vi "LNK223-429BLF-No2.vi"() -> ()   [LabVIEW 2018]
uses:
  vi/DualHeadTestStage.ctl
  <vilib>/DAQmx/write.llb/DAQmx Write (Digital Bool 1Line 1Point).vi
  <vilib>/DAQmx/write.llb/DAQmx Write (Digital 1D Bool 1Chan 1Samp).vi
  <vilib>/DAQmx/read.llb/DAQmx Read (Digital 1D Bool 1Chan 1Samp).vi
  <vilib>/DAQmx/read.llb/DAQmx Read (Digital Bool 1Line 1Point).vi
  <vilib>/DAQmx/miscellaneous.llb/DAQmx Fill In Error Info.vi
panel:
  in  "Operator Mode:":enum32{"Admin", "Technician", "Operator"}(radio)=enum."Operator" caption="Radio Buttons"
  out "message":string
  out "AllowToTest":bool
  in  "DataIn":T1={"W0-SN"="2022-09", "W1-CUSTOMER"="LNK", "W2-TEST_DATE"="11/07/2019-14:51:57", "W3-TESTER"="LNK908-220309LF", "W4-RESULT"="P", "W5-TEXT1"="10CB6S194-C-2 10193406", "W6-TEXT2"="995982-3406", "W7-TEXT3"="", "W8-TEXT4"="", "W9-OPNAME"="FCT1", "W10-CDATE"="11/07/2019-14:51:57", "W11-CRITERIA"="", "W12-SYMPTOM"="", "W13-OPERATOR"="", "W14-WORKORDER"="", "W15-FIXTURE_ID"="", "W16-APIWO"="", "W17-TESTDURATION"=""}
  out "NOTE":string
  out "Check SUM HEX":string
  out "Serial number (Hex)":string
  out "TestTimeStr":string
  out "ProjectShort":string
  out "Project908":string
  out "number 2":i32
  out "length":i32
  out "TESTING HEAD#":string
  out "LowLimit 2":string
  out "standard error":string
  out "standard output":string
  out "Avg4V8":dbl
  out "Avg2V9":dbl
  out "Avg2V1":dbl
  out "Avg1V3":dbl
  out "text":string
  out "PWIDTH":dbl format="%#_6f"
  out "MAX AMP":dbl format="%#_6f"
  out "E3643A":refnum<visa-resource-name>="USB0::0x0957::0xB318::MY52420094::INSTR"
  out "DSO1052B":refnum<visa-resource-name>="USB0::0x0957::0x0588::CN55040431::INSTR"
  out "Result(Boolean)":bool
  out "TDS2002B":refnum<visa-resource-name>="GPIB0::7::INSTR"
  out "concatenated string":string
  out "LogfileHeaderXLS":string
  out "LowLimitForIntValue":string
  out "HighLimitForIntValue":string
  out "LowLimitForPulseCnt+400":string
  out "HighLimitForPulseCnt+400":string
  out "SSI_HighLimit":string
  out "SSI_LowLimit":string
  out "Position Get SSI-Pos":sgl format="%.2f"
  out "Position Get SSI-Neg*-1":sgl format="%.2f"
  out "ADC val":sgl format="%.2f"
  out "DriveEnable":bool
  out "Result(Boolean) 4":bool
  out "Result(Boolean) 3":bool
  out "Result(Boolean) 2":bool
  out "Result(DecimalPoint)2":dbl
  out "MicroFlexRS232":refnum<visa-resource-name>="COM5"
  out "33210A":refnum<visa-resource-name>="USB0::0x0957::0xB318::MY52420094::INSTR"
  out "34461A":refnum<visa-resource-name>="USB0::0x0957::0xB318::MY52420094::INSTR"
  out "E3643A#3":refnum<visa-resource-name>="USB0::0x0957::0xB318::MY52420094::INSTR"
  out "E3643A#2":refnum<visa-resource-name>="USB0::0x0957::0xB318::MY52420094::INSTR"
  out "E3643A#1":refnum<visa-resource-name>="USB0::0x0957::0xB318::MY52420094::INSTR"
  out "KA3003P":refnum<visa-resource-name>
  out "Project index":i32
  out "KA6003P":refnum<visa-resource-name>
  out "A5114-12":refnum<visa-resource-name>
  out "A5116-02":refnum<visa-resource-name>
  out "SN-STS":i16
  out "TDS3012C":refnum<visa-resource-name>
  out "Result":string
  out "E3631A":refnum<visa-resource-name>="USB0::0x0957::0xB318::MY52420094::INSTR"
  out "Index TestTime":i16
  out "Break Step#":string
  in  "Clear list of break step":string[](array[string])
  out "RowSize":i32
  out "TestPlanDimensions":i32[](array[numeric])
  out "BreakStep#":string[](array[string])
  out "CMD":string
  out "Remark":string
  out "Equipment":string
  out "SetDelayResChk":i8
  out "Step#":string
  out "FailedFlag":i8
  out "TestLoop":string
  out "Return CMD":string
  out "Status of Set CMD":bool
  out "COMPST":string
  out "Reading":string
  out "UPL":string
  out "LWL":string
  out "Step&Description":string
  out "SeqFileSts":bool
  out "Start Time":dbl
  out "Comment":string
  out "StartTime":string
  out "Project":string
  out "CUSTOMER":string
  out "FIRMWARE REV":string
  out "SOFTWARE REV":string
  out "UNIT  PASS/FAIL STATUS":string
  out "TESTER ID":string
  out "LineLogFile":string
  out "SumDisp_Low_Inc":i32
  out "All Test Status in Sum Disp":string
  out "Test Step# >> Sum Disp":string
  out "Action":string
  out "Unit":string
  out "HighLimit":string
  out "LowLimit":string
  out "FailedCode":string
  out "Status >> Sum Disp":string
  out "Reading >> Sum Disp":string
  out "TESTPLAN ARRAY":string[][](array[string])
  out "BarCode Exit":bool
  out "TestPlan_Row_Inc":i32
  out "Ok STS":bool
  out "Project Model":string
  in  "Tab Control":T2(tab)
  out "TESTPLAN ARRAY Display":string[][](table) caption="Table Control"
  in  "Test Modes":enum32{"Auto", "Step"}(radio) caption="Test Mode:"
  out "ID STS":bool
  in  "ID OK":bool
  in  "Operator ID":string
  in  "stop":bool
  out "PASS/FAIL STATUS":bool caption="PASSED"
  out "Test Time (Sec)":dbl
  out "Serial Number":string
  in  "RunAllSeq?":bool
  in  "Break step#":string(combo)="Index"
  out "Index":string
  out "InitialValueAfter":i32
  out "FailedCdDisp":string
  out "ProjectFull":string
  out "Result(Boolean) 1":bool
  in  "RS485 RECEIVER":refnum<visa-resource-name>="COM7"
  out "Numeric":i32
  out "trimmed string":string
  out "number":dbl
  out "Username":string
  in  "Tab Control 2":enum32{"Test result", "Waveform"}(tab)
  out "Summary Display":string[][](table) caption="Table Control"
  out "WF_CCW":cluster{"Numeric":dbl, "Numeric":dbl}[](graph)
  out "WF_CW":cluster{"Numeric":dbl, "Numeric":dbl}[](graph)
  in  "SERIAL NUMBER HEAD 1":string
  in  "SERIAL NUMBER HEAD 2":string
  out "Test Time HEAD 1":dbl
  out "Test Time HEAD 2":dbl
  out "HEAD 1":u8(slide) scale=0.0..71.0
  out "HEAD 2":u8(slide) scale=0.0..71.0
  out "PASS/FAIL STATUS  HEAD 1":bool caption="PASSED"
  out "PASS/FAIL STATUS  HEAD 2":bool
  out "FailedCdDisp H1":string
  out "FailedCdDisp H2":string
  out "Result(DecimalPoint)":sgl format="%#_10g"
  out "Description":string
  out "App Firmware":string=" -openD:\\20161122\\LNK01E-213300ALF\\LNK213-300ALF\\SW0077076V1-04.hex"
  out "MUX RELAY":refnum<visa-resource-name>
  out "34450A":refnum<visa-resource-name>="USB0::0x0957::0xB318::MY52420094::INSTR"
  in  "34410A":refnum<visa-resource-name>="USB0::0x0957::0x0607::MY53018867::INSTR"
  out "Test time report":string[][](array[string])
  out "TestDesc+TestTime":string
  out "GeneralHeader":string
  out "TestDataHeader":string
  out "LogfileHeaderCSV":string
  out "FailedStep":string
  out "InitialValue":i32
  in  "Station":string="FCT1"
  in  "Fixture/PalletteID":string="1"
  in  "Note":string
  in  "Reserve#1":string
  in  "Reserve#2":string
  in  "TestSoftwareVersion":string="V1.0"
  out "Result(Number)":i32
  out "Result(string)":string
  out "VAR_TYPE":string
  out "Result(Number)2":i32
  in  "RUNTEST":bool
  in  "RESET_ICT100":bool
  in  "OK Button 2":bool
  in  "OK Button":bool
  out "Fail Test Param":string
  out "Stop_Buffer":bool
  # "1"
  # "0"
  # "USB0::0x0957::0x0607::MY53018867::INSTR"
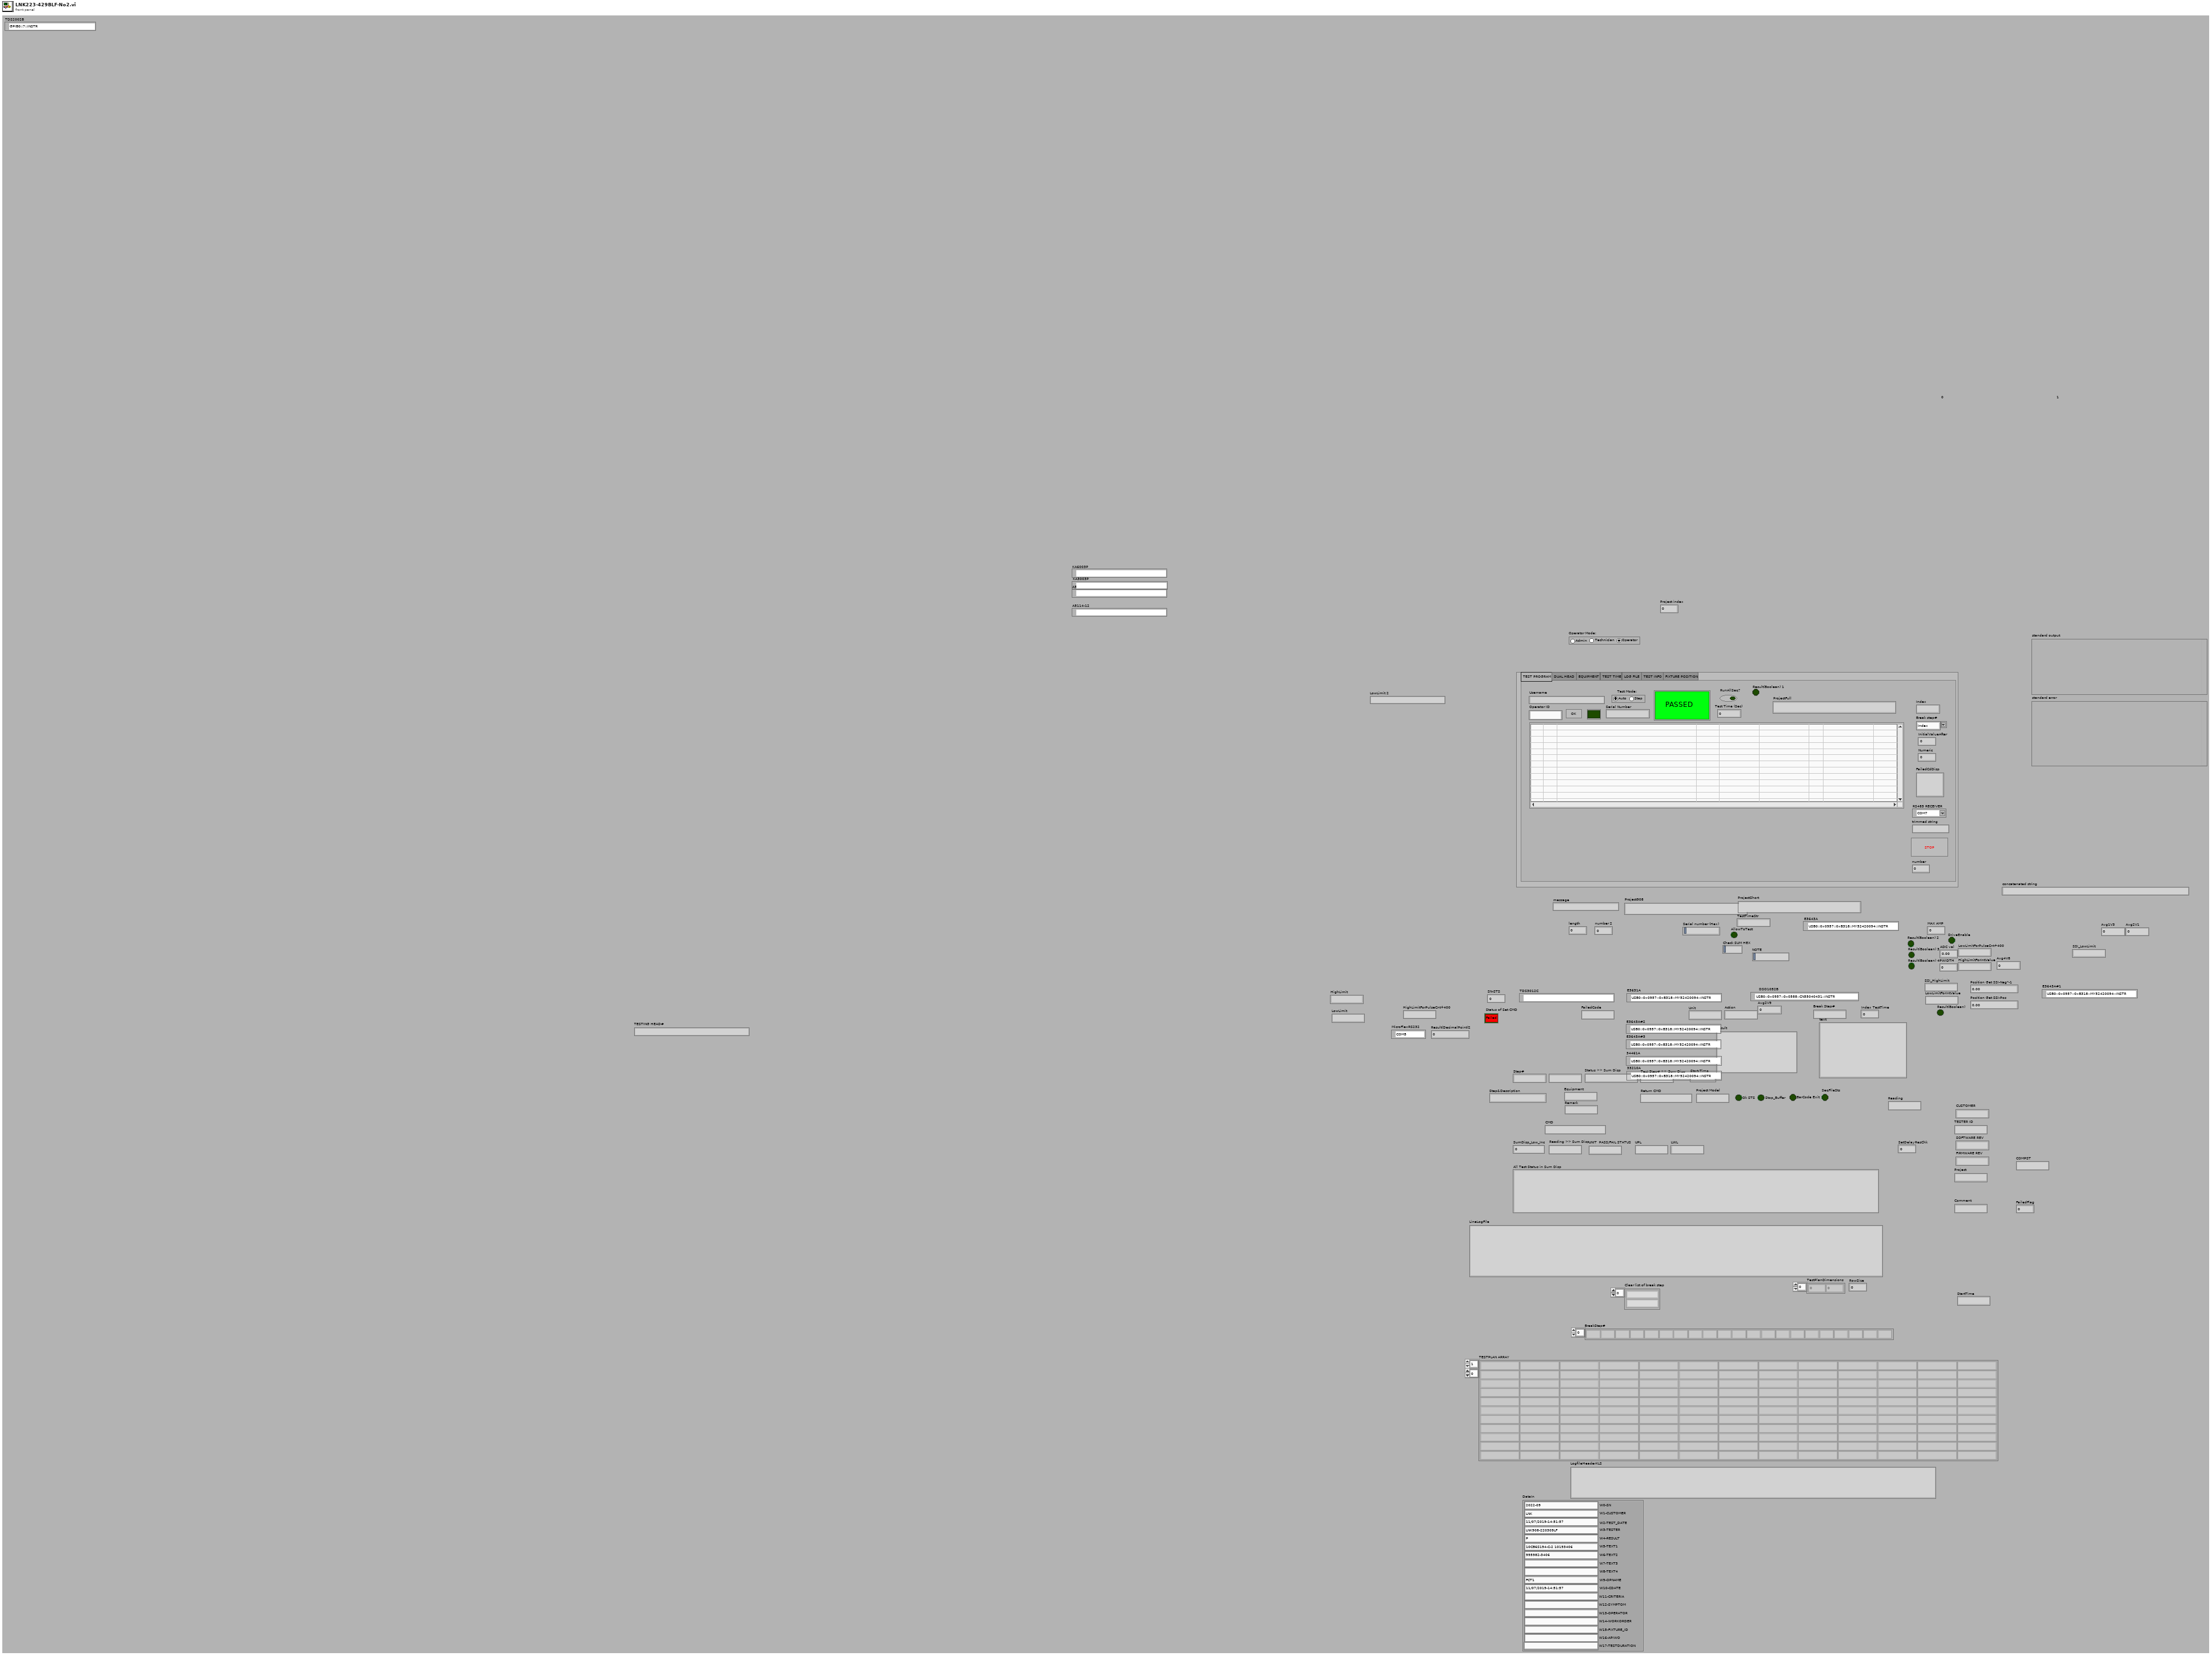
[diagram p1: front panel]
types:
  T1 = cluster{"W0-SN":string, "W1-CUSTOMER":string, "W2-TEST_DATE":string, "W3-TESTER":string, "W4-RESULT":string, "W5-TEXT1":string, "W6-TEXT2":string, "W7-TEXT3":string, "W8-TEXT4":string, "W9-OPNAME":string, "W10-CDATE":string, "W11-CRITERIA":string, "W12-SYMPTOM":string, "W13-OPERATOR":string, "W14-WORKORDER":string, "W15-FIXTURE_ID":string, "W16-APIWO":string, "W17-TESTDURATION":string}
  T2 = enum32{"TEST PROGRAM", "DUAL HEAD", "EQUIPMENT", "TEST TIME", "LOG FILE", "TEST INFO", "FIXTURE POSITION"}
  T3 = enum32{"1", "10", "20", "50", "100", "500", "1000"}
  T4 = enum32{"Set Relay", "Append Relay", "Clear Relay", "Manual Cmd"}
  T5 = typedef "DualHeadTestStage.ctl" = enum16{"Initial", "CheckHead1", "CheckHead2", "LoadTestPlanHead1", "LoadTestPlanHead2", "StartTest"}
  T6 = enum16{"FREQUENCY", "MEAN", "PERIOD", "PK2PK", "MIN", "MAX", "RISE", "FALL", "CRMS", "PWIDTH", "NWIDTH", "NONE"}
  T7 = enum16{"MEAS1", "MEAS2", "MEAS3", "MEAS4", "MEAS5"}
  T8 = cluster{"disabled index (col)":i32, "disabled index (col)":i32}
  T9 = cluster{"TestPlan_Row_Inc":i32, "disabled index (col)":i32}
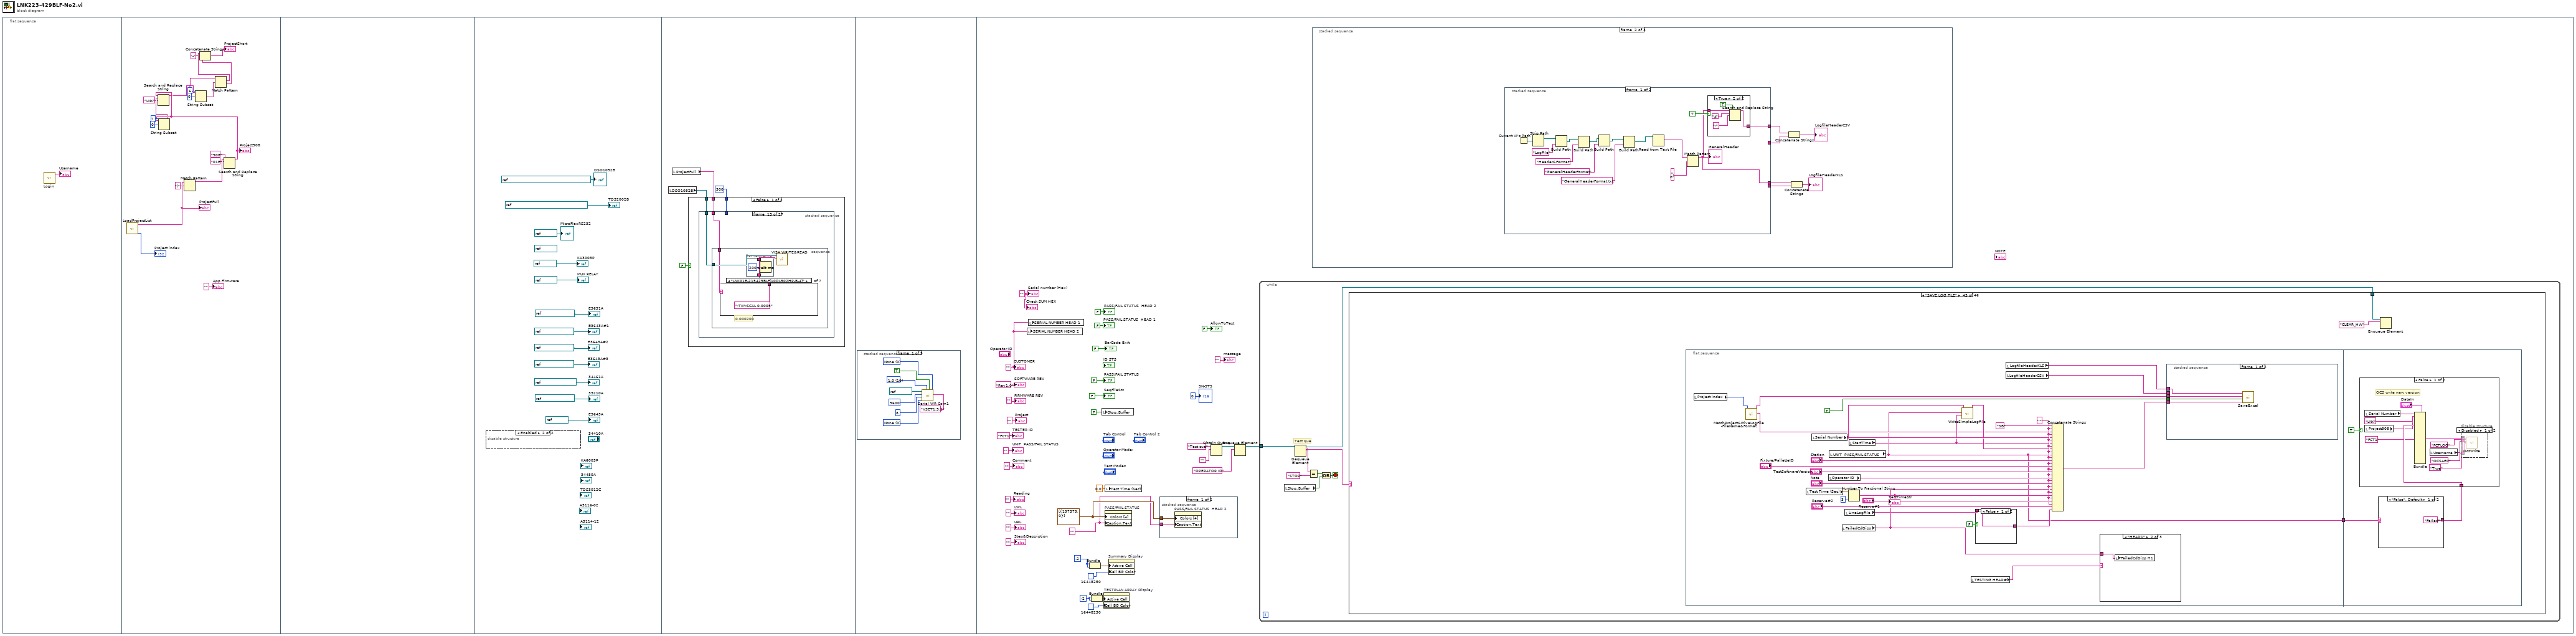
[diagram p0: block diagram]
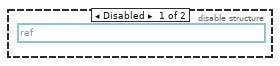
[diagram p2: hidden frame]
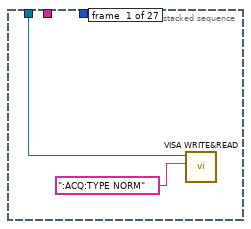
[diagram p3: hidden frame]
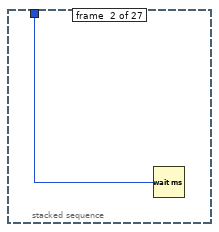
[diagram p4: hidden frame]
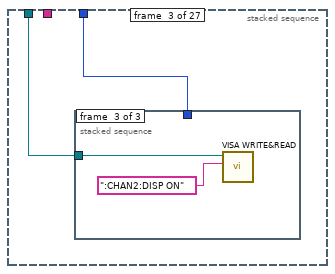
[diagram p5: hidden frame]
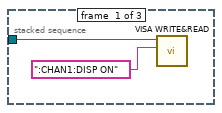
[diagram p6: hidden frame]
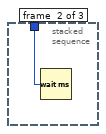
[diagram p7: hidden frame]
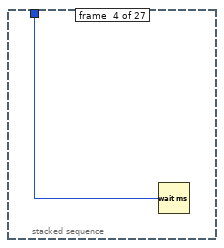
[diagram p8: hidden frame]
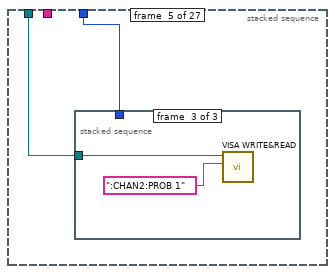
[diagram p9: hidden frame]
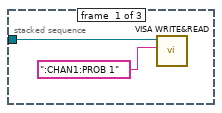
[diagram p10: hidden frame]
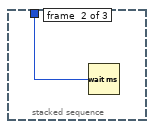
[diagram p11: hidden frame]
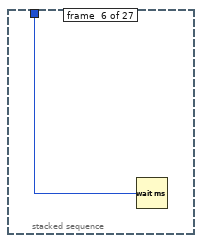
[diagram p12: hidden frame]
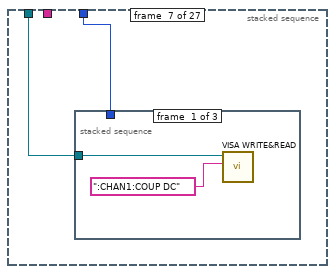
[diagram p13: hidden frame]
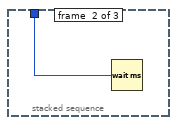
[diagram p14: hidden frame]
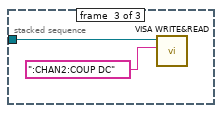
[diagram p15: hidden frame]
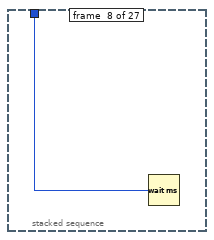
[diagram p16: hidden frame]
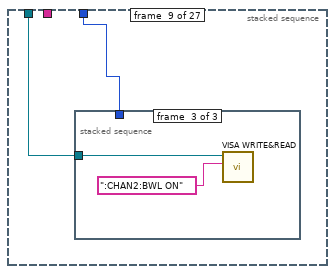
[diagram p17: hidden frame]
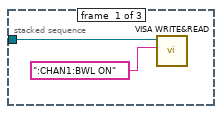
[diagram p18: hidden frame]
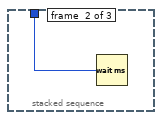
[diagram p19: hidden frame]
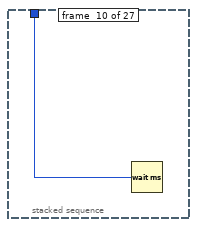
[diagram p20: hidden frame]
diagram:
  n1 = flat-sequence {
    frame #0 {
      n2 = call "Login.vi"() -> ("Username"=→"Username":string)  [unwired: 11 in]
    }
    frame #1 {
      n3 = call "LoadProjectList.vi"() -> ("Index"=→"Project index":i32, "SelectedProject"=w20:string)  [unwired: 10 out]
      "ProjectFull" <- w20
      n4 = Match Pattern(string=w20, regular expression="(") -> (before substring=w18:string)  [unwired: 1 in, 3 out]
      n5 = Search and Replace String(input string=w18, search string="01E", replace string="908" ("replace string (\"\")")) -> (result string=w12:string)  [unwired: 5 in, 3 out]
      "Project908" <- w12
      n6 = String Subset(string=w12, offset (0)=0, length (rest)=7 ("length (rest)")) -> (substring=w13:string)
      n7 = Search and Replace String(input string=w12, search string=w13, replace string="LNK" ("replace string (\"\")")) -> (result string=w8:string)  [unwired: 5 in, 3 out]
      n8 = String Subset(string=w8, offset (0)=0, length (rest)=6 ("length (rest)")) -> (substring=w7:string)
      n9 = Match Pattern(string=w8, regular expression=w7) -> (match substring=w6:string, after substring=w5:string)  [unwired: 1 in, 2 out]
      n10 = Concatenate Strings(w6, "-" ("string"), w5) -> (→"ProjectShort":string)
      "App Firmware" <- "" ("App Firmware")
    }
    frame #2 {
    }
    frame #3 {
      (unwired) refnum<visa-resource-name> "COM1" ("SPK RELAY")
      n11 = disable-structure shown="Enabled" {
        frame Disabled {
          (unwired) refnum<visa-resource-name> "USB0::0x0957::0x0607::MY53018867::INSTR" ("E3631A")
        }
        frame Enabled {
        }
      }
      "MUX RELAY" <- refnum<visa-resource-name> "COM1" ("SPK RELAY")
      "E3631A" <- refnum<visa-resource-name> "GPIB0::1::INSTR" ("E3631A")
      "KA3003P" <- refnum<visa-resource-name> "COM2" ("SPK RELAY")
      "E3643A#1" <- refnum<visa-resource-name> "GPIB0::2::INSTR" ("E3631A")
      "E3643A#2" <- refnum<visa-resource-name> "GPIB0::3::INSTR" ("E3631A")
      "E3643A#3" <- refnum<visa-resource-name> "GPIB0::4::INSTR" ("E3631A")
      "34461A" <- refnum<visa-resource-name> "GPIB0::22::INSTR" ("E3631A")
      "33210A" <- refnum<visa-resource-name> "GPIB0::6::INSTR" ("E3631A")
      "MicroFlexRS232" <- refnum<visa-resource-name> "COM5" ("SPK RELAY")
      "TDS2002B" <- refnum<visa-resource-name> "USB0::0x0699::0x03A1::C041443::INSTR" ("TDS1001B")
      "DSO1052B" <- refnum<visa-resource-name> "USB0::0x0957::0x0588::CN56489397::INSTR" ("VISA resource name In")
      "E3643A" <- refnum<visa-resource-name> "COM3" ("E3643A#1 2")
    }
    frame #4 {
      n12 = local read "DSO1052B"() -> (w36:refnum<visa-resource-name>)
      n13 = local read "ProjectFull"() -> (w34:string)
      n14 = case shown="False" FALSE {
        tunnel: w36 -> [w40 _]
        tunnel: u32 300 ("milliseconds to wait") -> [w39 _]
        tunnel: w34 -> [w38 _]
        frame False {
          n15 = stacked-sequence {
            tunnel: w40 -> [w42 _ w45 _ w53 _ w61 _ w69 _ w77 _ w85 _ w100 _ w104 _ w108 _ w113 _ w123 _ w132 w148 w154]
            tunnel: w39 -> [_ w43 w44 w51 w52 w59 w60 w67 w68 w75 w76 w83 _ w99 _ w103 _ w107 _ w111 _ w121 w122 w129 w131 w149 w153]
            tunnel: w38 -> [_ _ _ _ _ _ _ _ _ _ _ _ w84 _ _ _ _ _ _ _ w112 _ _ _ w130 _ _]
            frame #0 {
              n16 = call "VISA WRITE&READ.vi"("write buffer"=":ACQ:TYPE NORM", "VISA resource name In"=w42) -> ()  [unwired: 7 in, 3 out]
            }
            frame #1 {
              n17 = Wait (ms)(milliseconds to wait=w43) -> ()  [unwired: 1 out]
            }
            frame #2 {
              n18 = stacked-sequence {
                tunnel: w45 -> [w47 _ w50]
                tunnel: w44 -> [_ w48 _]
                frame #0 {
                  n19 = call "VISA WRITE&READ.vi"("write buffer"=":CHAN1:DISP ON", "VISA resource name In"=w47) -> ()  [unwired: 7 in, 3 out]
                }
                frame #1 {
                  n20 = Wait (ms)(milliseconds to wait=w48) -> ()  [unwired: 1 out]
                }
                frame #2 {
                  n21 = call "VISA WRITE&READ.vi"("write buffer"=":CHAN2:DISP ON", "VISA resource name In"=w50) -> ()  [unwired: 7 in, 3 out]
                }
              }
            }
            frame #3 {
              n22 = Wait (ms)(milliseconds to wait=w51) -> ()  [unwired: 1 out]
            }
            frame #4 {
              n23 = stacked-sequence {
                tunnel: w53 -> [w55 _ w58]
                tunnel: w52 -> [_ w56 _]
                frame #0 {
                  n24 = call "VISA WRITE&READ.vi"("write buffer"=":CHAN1:PROB 1", "VISA resource name In"=w55) -> ()  [unwired: 7 in, 3 out]
                }
                frame #1 {
                  n25 = Wait (ms)(milliseconds to wait=w56) -> ()  [unwired: 1 out]
                }
                frame #2 {
                  n26 = call "VISA WRITE&READ.vi"("write buffer"=":CHAN2:PROB 1", "VISA resource name In"=w58) -> ()  [unwired: 7 in, 3 out]
                }
              }
            }
            frame #5 {
              n27 = Wait (ms)(milliseconds to wait=w59) -> ()  [unwired: 1 out]
            }
            frame #6 {
              n28 = stacked-sequence {
                tunnel: w61 -> [w63 _ w66]
                tunnel: w60 -> [_ w64 _]
                frame #0 {
                  n29 = call "VISA WRITE&READ.vi"("write buffer"=":CHAN1:COUP DC", "VISA resource name In"=w63) -> ()  [unwired: 7 in, 3 out]
                }
                frame #1 {
                  n30 = Wait (ms)(milliseconds to wait=w64) -> ()  [unwired: 1 out]
                }
                frame #2 {
                  n31 = call "VISA WRITE&READ.vi"("write buffer"=":CHAN2:COUP DC", "VISA resource name In"=w66) -> ()  [unwired: 7 in, 3 out]
                }
              }
            }
            frame #7 {
              n32 = Wait (ms)(milliseconds to wait=w67) -> ()  [unwired: 1 out]
            }
            frame #8 {
              n33 = stacked-sequence {
                tunnel: w69 -> [w71 _ w74]
                tunnel: w68 -> [_ w72 _]
                frame #0 {
                  n34 = call "VISA WRITE&READ.vi"("write buffer"=":CHAN1:BWL ON", "VISA resource name In"=w71) -> ()  [unwired: 7 in, 3 out]
                }
                frame #1 {
                  n35 = Wait (ms)(milliseconds to wait=w72) -> ()  [unwired: 1 out]
                }
                frame #2 {
                  n36 = call "VISA WRITE&READ.vi"("write buffer"=":CHAN2:BWL ON", "VISA resource name In"=w74) -> ()  [unwired: 7 in, 3 out]
                }
              }
            }
            frame #9 {
              n37 = Wait (ms)(milliseconds to wait=w75) -> ()  [unwired: 1 out]
            }
            frame #10 {
              n38 = stacked-sequence {
                tunnel: w77 -> [w79 _ w82]
                tunnel: w76 -> [_ w80 _]
                frame #0 {
                  n39 = call "VISA WRITE&READ.vi"("write buffer"=":CHAN1:INV OFF", "VISA resource name In"=w79) -> ()  [unwired: 7 in, 3 out]
                }
                frame #1 {
                  n40 = Wait (ms)(milliseconds to wait=w80) -> ()  [unwired: 1 out]
                }
                frame #2 {
                  n41 = call "VISA WRITE&READ.vi"("write buffer"=":CHAN2:INV OFF", "VISA resource name In"=w82) -> ()  [unwired: 7 in, 3 out]
                }
              }
            }
            frame #11 {
              n42 = Wait (ms)(milliseconds to wait=w83) -> ()  [unwired: 1 out]
            }
            frame #12 {
              n43 = stacked-sequence {
                tunnel: w85 -> [w89]
                tunnel: w84 -> [w88]
                frame #0 {
                  # "0.000200"
                  n44 = case shown="\"LNK01E-215429BLF(10DL502HP-B-4)\"" w88 {
                    tunnel: [":TIM:SCAL 0.01" ("write buffer") ":TIM:SCAL 0.005" ("write buffer") ":TIM:SCAL 0.01" ("write buffer") ":TIM:SCAL 0.0005" ("write buffer") ":TIM:SCAL 0.0005" ("write buffer") ":TIM:SCAL 0.0005" ("write buffer") ":TIM:SCAL 0.0005" ("write buffer")] -> w86
                    frame "False", Default {
                    }
                    frame "LNK01E-213299LF(10DL5H)" {
                    }
                    frame "LNK01E-213301LF(10DL4H)" {
                    }
                    frame "LNK01E-213300ALF(10DL12H)" {
                    }
                    frame "LNK01E-215429ALF(10DL502HP)" {
                    }
                    frame "LNK01E-223429BLF(10DL502HP-D-0)" {
                    }
                    frame "LNK01E-215429BLF(10DL502HP-B-4)" {
                    }
                  }
                  n45 = flat-sequence {
                    tunnel: [w91] -> w87
                    tunnel: w86 -> [w91]
                    frame #0 {
                      n46 = Wait (ms)(milliseconds to wait=u32 200) -> ()  [unwired: 1 out]
                    }
                  }
                  n47 = call "VISA WRITE&READ.vi"("write buffer"=w87, "VISA resource name In"=w89) -> ()  [unwired: 7 in, 3 out]
                }
              }
            }
            frame #13 {
              n48 = Wait (ms)(milliseconds to wait=w99) -> ()  [unwired: 1 out]
            }
            frame #14 {
              n49 = stacked-sequence {
                tunnel: w100 -> [w102]
                frame #0 {
                  n50 = call "VISA WRITE&READ.vi"("write buffer"=":TRIG:MODE EDGE", "VISA resource name In"=w102) -> ()  [unwired: 7 in, 3 out]
                }
              }
            }
            frame #15 {
              n51 = Wait (ms)(milliseconds to wait=w103) -> ()  [unwired: 1 out]
            }
            frame #16 {
              n52 = stacked-sequence {
                tunnel: w104 -> [w106]
                frame #0 {
                  n53 = call "VISA WRITE&READ.vi"("write buffer"=":TRIG:EDGE:SLOP POS", "VISA resource name In"=w106) -> ()  [unwired: 7 in, 3 out]
                }
              }
            }
            frame #17 {
              n54 = Wait (ms)(milliseconds to wait=w107) -> ()  [unwired: 1 out]
            }
            frame #18 {
              n55 = stacked-sequence {
                tunnel: w108 -> [w110]
                frame #0 {
                  n56 = call "VISA WRITE&READ.vi"("write buffer"=":TRIG:EDGE:SOUR CHAN2", "VISA resource name In"=w110) -> ()  [unwired: 7 in, 3 out]
                }
              }
            }
            frame #19 {
              n57 = Wait (ms)(milliseconds to wait=w111) -> ()  [unwired: 1 out]
            }
            frame #20 {
              n58 = stacked-sequence {
                tunnel: w113 -> [w116]
                tunnel: w112 -> [w114]
                frame #0 {
                  n59 = case shown="\"LNK01E-213300LF(10DL12H)\"" w114 {
                    tunnel: [":TRIG:EDGE:LEV 2.5" ("write buffer") ":TRIG:EDGE:LEV 8" ("write buffer") ":TRIG:EDGE:LEV 2.5" ("write buffer") ":TRIG:EDGE:LEV 4" ("write buffer")] -> w115
                    frame "False", Default {
                    }
                    frame "LNK01E-213299LF(10DL5H)" {
                    }
                    frame "LNK01E-213301LF(10DL4H)" {
                    }
                    frame "LNK01E-213300LF(10DL12H)" {
                    }
                  }
                  n60 = call "VISA WRITE&READ.vi"("write buffer"=w115, "VISA resource name In"=w116) -> ()  [unwired: 7 in, 3 out]
                }
              }
            }
            frame #21 {
              n61 = Wait (ms)(milliseconds to wait=w121) -> ()  [unwired: 1 out]
            }
            frame #22 {
              n62 = stacked-sequence {
                tunnel: w123 -> [w125 _ w128]
                tunnel: w122 -> [_ w126 _]
                frame #0 {
                  n63 = call "VISA WRITE&READ.vi"("write buffer"=":CHAN1:SCAL 2", "VISA resource name In"=w125) -> ()  [unwired: 7 in, 3 out]
                }
                frame #1 {
                  n64 = Wait (ms)(milliseconds to wait=w126) -> ()  [unwired: 1 out]
                }
                frame #2 {
                  n65 = call "VISA WRITE&READ.vi"("write buffer"=":CHAN2:SCAL 2", "VISA resource name In"=w128) -> ()  [unwired: 7 in, 3 out]
                }
              }
            }
            frame #23 {
              n66 = Wait (ms)(milliseconds to wait=w129) -> ()  [unwired: 1 out]
            }
            frame #24 {
              n67 = stacked-sequence {
                tunnel: w132 -> [w135 _ w143]
                tunnel: w131 -> [_ w140 _]
                tunnel: w130 -> [w134 _ w141]
                frame #0 {
                  n68 = case shown="\"LNK01E-213300LF(10DL12H)\"" w134 {
                    tunnel: [":CHAN1:OFFS -6" ("write buffer") ":CHAN1:OFFS -6" ("write buffer") ":CHAN1:OFFS -6" ("write buffer") ":CHAN1:OFFS 0" ("write buffer")] -> w133
                    frame "False", Default {
                    }
                    frame "LNK01E-213299LF(10DL5H)" {
                    }
                    frame "LNK01E-213301LF(10DL4H)" {
                    }
                    frame "LNK01E-213300LF(10DL12H)" {
                    }
                  }
                  n69 = call "VISA WRITE&READ.vi"("write buffer"=w133, "VISA resource name In"=w135) -> ()  [unwired: 7 in, 3 out]
                }
                frame #1 {
                  n70 = Wait (ms)(milliseconds to wait=w140) -> ()  [unwired: 1 out]
                }
                frame #2 {
                  n71 = case shown="\"LNK01E-213300LF(10DL12H)\"" w141 {
                    tunnel: [":CHAN2:OFFS -6" ("write buffer") ":CHAN2:OFFS -6" ("write buffer") ":CHAN2:OFFS -6" ("write buffer") ":CHAN2:OFFS 0" ("write buffer")] -> w142
                    frame "False", Default {
                    }
                    frame "LNK01E-213299LF(10DL5H)" {
                    }
                    frame "LNK01E-213301LF(10DL4H)" {
                    }
                    frame "LNK01E-213300LF(10DL12H)" {
                    }
                  }
                  n72 = call "VISA WRITE&READ.vi"("write buffer"=w142, "VISA resource name In"=w143) -> ()  [unwired: 7 in, 3 out]
                }
              }
            }
            frame #25 {
              n73 = stacked-sequence {
                tunnel: w149 -> [w150 _]
                tunnel: w148 -> [_ w152]
                frame #0 {
                  n74 = Wait (ms)(milliseconds to wait=w150) -> ()  [unwired: 1 out]
                }
                frame #1 {
                  n75 = call "VISA WRITE&READ.vi"("write buffer"=":TIM:MAIN:OFFS  0", "VISA resource name In"=w152) -> ()  [unwired: 7 in, 3 out]
                }
              }
            }
            frame #26 {
              n76 = stacked-sequence {
                tunnel: w154 -> [w156 _ w159]
                tunnel: w153 -> [_ w157 _]
                frame #0 {
                  n77 = call "DSO1072B_WaveformCMD1.vi"("DSO1072B CMD"=":WAV:POIN:MODE MAX", "VISA resource name In"=w156) -> ()  [unwired: 7 in, 3 out]
                }
                frame #1 {
                  n78 = Wait (ms)(milliseconds to wait=w157) -> ()  [unwired: 1 out]
                }
                frame #2 {
                  n79 = call "DSO1072B_WaveformCMD1.vi"("DSO1072B CMD"=":WAV:FORM BYTE", "VISA resource name In"=w159) -> ()  [unwired: 7 in, 3 out]
                }
              }
            }
          }
        }
        frame True {
          n80 = stacked-sequence {
            frame #0 {
              n81 = local read "TDS2002B"() -> (w160:refnum<visa-resource-name>)
              n82 = call "RUN-STOP-SING SEQ.vi"("VISA"=w160, "ACQUIRE"=enum32{"RUN", "SINGLE SEQ"}."RUN") -> ()
            }
            frame #1 {
              n83 = local read "TDS2002B"() -> (w163:refnum<visa-resource-name>)
              n84 = call "ACQMODE.vi"("ACQ MODE"=enum16{"SAMPLE", "PEAK DETECT", "AVERAGE"}."PEAK DETECT", "VISA resource name"=w163) -> ()  [unwired: 1 in]
            }
            frame #2 {
              n85 = local read "TDS2002B"() -> (w164:refnum<visa-resource-name>)
              n86 = call "SELECT_CHANEL.vi"("VISA resource name"=w164, "CH4"=FALSE, "CH3"=FALSE, "CH2"=TRUE, "CH1"=TRUE) -> ()
            }
            frame #3 {
              n87 = stacked-sequence {
                frame #0 {
                  n88 = local read "TDS2002B"() -> (w171:refnum<visa-resource-name>)
                  n89 = call "PROB ATTEN SETTING.vi"("ATTENUATIONs:"=T3."1", "CHANNEL"=enum32{"CH 1", "CH 2", "CH 3", "CH 4"}."CH 1", "VISA resource name 2"=w171) -> ()  [unwired: 9 in]
                }
                frame #1 {
                  n90 = local read "TDS2002B"() -> (w174:refnum<visa-resource-name>)
                  n91 = call "PROB ATTEN SETTING.vi"("ATTENUATIONs:"=T3."1", "CHANNEL"=enum32{"CH 1", "CH 2", "CH 3", "CH 4"}."CH 2", "VISA resource name 2"=w174) -> ()  [unwired: 9 in]
                }
              }
            }
            frame #4 {
              n92 = stacked-sequence {
                frame #0 {
                  n93 = local read "TDS2002B"() -> (w177:refnum<visa-resource-name>)
                  n94 = call "CH COUPLING SETTING.vi"("COUPLING:"=enum32{"AC", "DC", "GND"}."DC", "CHANNEL"=enum32{"CH 1", "CH 2", "CH 3", "CH 4"}."CH 1", "VISA resource name 2"=w177) -> ()  [unwired: 9 out]
                }
                frame #1 {
                  n95 = local read "TDS2002B"() -> (w180:refnum<visa-resource-name>)
                  n96 = call "CH COUPLING SETTING.vi"("COUPLING:"=enum32{"AC", "DC", "GND"}."DC", "CHANNEL"=enum32{"CH 1", "CH 2", "CH 3", "CH 4"}."CH 2", "VISA resource name 2"=w180) -> ()  [unwired: 9 out]
                }
              }
            }
            frame #5 {
              n97 = stacked-sequence {
                frame #0 {
                  n98 = local read "TDS2002B"() -> (w181:refnum<visa-resource-name>)
                  n99 = call "PROBE INV SETTING.vi"("INV / NON INV"=enum16{"NON INV", "INV"}."NON INV", "CH"=enum16{"CH 1", "CH 2", "CH 3", "CH 4"}."CH 1", "VISA TSD2014B"=w181) -> ()  [unwired: 9 in]
                }
                frame #1 {
                  n100 = local read "TDS2002B"() -> (w184:refnum<visa-resource-name>)
                  n101 = call "PROBE INV SETTING.vi"("INV / NON INV"=enum16{"NON INV", "INV"}."NON INV", "CH"=enum16{"CH 1", "CH 2", "CH 3", "CH 4"}."CH 2", "VISA TSD2014B"=w184) -> ()  [unwired: 9 out]
                }
              }
            }
            frame #6 {
              n102 = local read "TDS2002B"() -> (w187:refnum<visa-resource-name>)
              n103 = call "HOR_POS_SETTING.vi"("VISA TDS1012"=w187, "HOR_POS (SEC)   LEFT=+  RIGHT=-"="0") -> ()
            }
            frame #7 {
              n104 = local read "TDS2002B"() -> (w190:refnum<visa-resource-name>)
              n105 = call "HOR_SCALE_SETTING.vi"("VISA TDS1012"=w190, "HOR_SCAIL"="5E-3") -> ()
            }
            frame #8 {
              n106 = local read "TDS2002B"() -> (w193:refnum<visa-resource-name>)
              n107 = call "TRIGER_EDGE.vi"("TRIGGER EDGE"=enum32{"SLOPE RISE", "SLOPE FALL"}."SLOPE RISE", "SOURCE"=enum32{"CH 1", "CH 2", "CH 3", "CH 4"}."CH 1", "VISA TDS1012"=w193) -> ()
            }
            frame #9 {
              n108 = local read "TDS2002B"() -> (w196:refnum<visa-resource-name>)
              n109 = call "TRIGER_LEVEL.vi"("VISA resource name"=w196, "V Unit"=enum32{"mVOLT", "VOLT"}."VOLT", "TRIGER MAIN LEVEL"="2.5") -> ()
            }
            frame #10 {
              n110 = stacked-sequence {
                frame #0 {
                  n111 = local read "TDS2002B"() -> (w199:refnum<visa-resource-name>)
                  n112 = call "VER_POS_SETTING.vi"("VER POS"="1", "VOLTS/DIV"=enum32{"CH1", "CH2", "CH3", "CH4"}."CH1", "VISA resource name"=w199) -> ()
                }
                frame #1 {
                  n113 = local read "TDS2002B"() -> (w202:refnum<visa-resource-name>)
                  n114 = call "VER_SCALE_SETTING.vi"("VER RANGE"="2", "VOLTS/DIV"=enum32{"CH 1", "CH 2", "CH 3", "CH 4"}."CH 1", "VISA resource name"=w202) -> ()
                }
              }
            }
            frame #11 {
              n115 = stacked-sequence {
                frame #0 {
                  n116 = local read "TDS2002B"() -> (w205:refnum<visa-resource-name>)
                  n117 = call "VER_POS_SETTING.vi"("VER POS"="-3", "VOLTS/DIV"=enum32{"CH1", "CH2", "CH3", "CH4"}."CH2", "VISA resource name"=w205) -> ()
                }
                frame #1 {
                  n118 = local read "TDS2002B"() -> (w208:refnum<visa-resource-name>)
                  n119 = call "VER_SCALE_SETTING.vi"("VER RANGE"="2", "VOLTS/DIV"=enum32{"CH 1", "CH 2", "CH 3", "CH 4"}."CH 2", "VISA resource name"=w208) -> ()
                }
              }
            }
          }
        }
      }
    }
    frame #5 {
      n120 = stacked-sequence {
        frame #0 {
          w211 = u16 0 items=["None"=0, "XON/XOFF"=1, "RTS/CTS"=2, "DTR/DSR"=4] ("flow control")
          w213 = u16 10 items=["1.0"=10, "1.5"=15, "2.0"=20] ("stop bits")
          w214 = u16 0 items=["None", "Odd", "Even", "Mark", "Space"] ("parity")
          n121 = call "Serial WR Com1.vi"("string to write"="VSET1:5.1", "flow control"=w211, "write"=TRUE, "stop bits"=w213, "parity"=w214, "data bits"=u16 8, "baud rate"=u32 9600, "VISA resource name"=refnum<visa-resource-name> "COM2") -> ()  [unwired: 2 in, 2 out]
        }
        frame #1 {
          w222 = u16 0 items=["None"=0, "XON/XOFF"=1, "RTS/CTS"=2, "DTR/DSR"=4] ("flow control")
          w220 = u16 10 items=["1.0"=10, "1.5"=15, "2.0"=20] ("stop bits")
          w219 = u16 0 items=["None", "Odd", "Even", "Mark", "Space"] ("parity")
          n122 = call "Serial WR Com1.vi"("string to write"="ISET1:0.05", "flow control"=w222, "write"=TRUE, "stop bits"=w220, "parity"=w219, "data bits"=u16 8, "baud rate"=u32 9600, "VISA resource name"=refnum<visa-resource-name> "COM2") -> ()  [unwired: 2 in, 2 out]
        }
        frame #2 {
          w227 = u16 0 items=["None"=0, "XON/XOFF"=1, "RTS/CTS"=2, "DTR/DSR"=4] ("flow control")
          w229 = u16 10 items=["1.0"=10, "1.5"=15, "2.0"=20] ("stop bits")
          w230 = u16 0 items=["None", "Odd", "Even", "Mark", "Space"] ("parity")
          n123 = call "Serial WR Com1.vi"("string to write"="OUT1", "flow control"=w227, "write"=TRUE, "stop bits"=w229, "parity"=w230, "data bits"=u16 8, "baud rate"=u32 9600, "VISA resource name"=refnum<visa-resource-name> "COM2") -> ()  [unwired: 2 in, 2 out]
        }
        frame #3 {
          w241 = u16 0 items=["None"=0, "XON/XOFF"=1, "RTS/CTS"=2, "DTR/DSR"=4] ("flow control")
          w239 = u16 10 items=["1.0"=10, "1.5"=15, "2.0"=20] ("stop bits")
          w238 = u16 0 items=["None", "Odd", "Even", "Mark", "Space"] ("parity")
          n124 = Concatenate Strings("APPL 13.2,0.1" ("string to write"), "\r\n") -> (w234:string)
          n125 = call "Serial WR Com1.vi"("string to write"=w234, "flow control"=w241, "write"=TRUE, "stop bits"=w239, "parity"=w238, "data bits"=u16 8, "baud rate"=u32 9600, "VISA resource name"=refnum<visa-resource-name> "COM3") -> ()  [unwired: 2 in, 2 out]
        }
        frame #4 {
          w251 = u16 0 items=["None"=0, "XON/XOFF"=1, "RTS/CTS"=2, "DTR/DSR"=4] ("flow control")
          w249 = u16 10 items=["1.0"=10, "1.5"=15, "2.0"=20] ("stop bits")
          w248 = u16 0 items=["None", "Odd", "Even", "Mark", "Space"] ("parity")
          n126 = Concatenate Strings("OUTP ON" ("string to write"), "\r\n") -> (w244:string)
          n127 = call "Serial WR Com1.vi"("string to write"=w244, "flow control"=w251, "write"=TRUE, "stop bits"=w249, "parity"=w248, "data bits"=u16 8, "baud rate"=u32 9600, "VISA resource name"=refnum<visa-resource-name> "COM3") -> ()  [unwired: 2 in, 2 out]
        }
      }
    }
    frame #6 {
      w255 = "" ("Serial number (Hex)")
      w262 = -2 ("disabled index (col)")
      w266 = -2
      w257 = "" ("Caption.Text")
      w258 = cluster{u32, u32}[] [{197379, 0}] ("Colors [4]")
      w256 = "" ("SOFTWARE REV")
      n128 = local write "SERIAL NUMBER HEAD 2"(w256) -> ()
      n129 = local write "SERIAL NUMBER HEAD 1"(w256) -> ()
      n130 = Bundle(w266, w266) -> (w267:cluster{i32, i32})  [unwired: 1 out]
      n131 = Bundle("disabled index (col)"=w262, "disabled index (col)"=w262) -> (w263:T8)  [unwired: 1 out]
      n132 = local write "Stop_Buffer"(FALSE ("Stop_Buffer")) -> ()
      n133 = property on="TESTPLAN ARRAY Display" class="Tbl (strict)"("Active Cell"=w263, "Cell BG Color"=u32 16448250) -> ()  [unwired: 2 in, 2 out]
      n134 = property on="PASS/FAIL STATUS" class="Bool (strict)"("Colors [4]"=w258, "Caption.Text"=w257) -> ()  [unwired: 2 in, 2 out]
      n135 = local write "Test Time (Sec)"(0.0 ("Cycle Time (Sec)")) -> ()
      n136 = property on="Summary Display" class="Tbl (strict)"("Active Cell"=w267, "Cell BG Color"=u32 16448250) -> ()  [unwired: 2 in, 2 out]
      n137 = stacked-sequence {
        tunnel: w258 -> [w289 w291]
        tunnel: w257 -> [w288 w290]
        frame #0 {
          n138 = property on="PASS/FAIL STATUS  HEAD 2" class="Bool (strict)"("Colors [4]"=w289, "Caption.Text"=w288) -> ()  [unwired: 2 in, 2 out]
        }
        frame #1 {
          n139 = property on="PASS/FAIL STATUS  HEAD 1" class="Bool (strict)"("Colors [4]"=w291, "Caption.Text"=w290) -> ()  [unwired: 2 in, 2 out]
        }
      }
      n140 = Obtain Queue(name (unnamed)="Test cue", element data type="") -> (queue out=w286:refnum<queue>)  [unwired: 3 in, 2 out]
      n141 = Enqueue Element(queue=w286, element="OPERATOR ID") -> (queue out=w283:refnum<queue>)  [unwired: 1 in, 3 out]
      n142 = while {
        tunnel: w283 -> [w416]
        stop <- w412 stop-if-true
        # "Test que"
        n143 = local read "Stop_Buffer"() -> (w411:bool)
        n144 = Dequeue Element(queue=w416) -> (queue out=w413:refnum<queue>, element=w414:string)  [unwired: 1 in, 3 out]
        n145 = Equal?(x=w414, y="STOP") -> (x = y?=w410:bool)
        n146 = Or(x=w410, y=w411) -> (x .or. y?=w412:bool)
        n147 = case shown="\"SAVE LOG FILE\"" w414 {
          tunnel: w413 -> [_ w418 w572 w639 w806 w930 w947 w959 w990 w1018 w1034 w1046 w1152 w1377 w1430 w1449 w1563 w1571 w1583 w1586 w1588 w1596 w1610 w1613 w1636 w1671 w1706 w1741 w1776 w1807 w1832 w1843 w1858 w1903 w2036 w2051 w2087 w2173 w2184 w2186 w2319 w2473 w2509 _ w2595 w2606]
          frame "False", Default {
            n148 = One Button Dialog(message="There is a wrong command or text error in test sequence file, Please check! ") -> ()  [unwired: 2 out]
          }
          frame "DUAL-HEAD-TESTING" {
            n149 = while {
              shift-right: [w422] -> _
              shift-left: DualHeadTestStage."Initial" ("DualHeadTestStage") -> [w423]
              tunnel: w418 -> [w421]
              stop <- w420 stop-if-true
              n150 = case shown="\"CheckHead2\"" w423 {
                tunnel: [DualHeadTestStage."CheckHead1" ("DualHeadTestStage") w434 w451 w463 w478 DualHeadTestStage."Initial" ("DualHeadTestStage")] -> w422
                tunnel: w421 -> [_ _ _ _ _ w570]
                tunnel: [FALSE FALSE FALSE FALSE FALSE TRUE] -> w420
                frame "Initial", Default {
                  w424 = u8 0 ("HEAD 2")
                  n151 = local write "HEAD 1"(w424) -> ()
                  n152 = local write "HEAD 2"(w424) -> ()
                  "TESTING HEAD#" <- "" ("TESTING HEAD#")
                }
                frame "CheckHead1" {
                  n153 = local read "ProjectFull"() -> (w439:string)
                  n154 = case shown="\"False\", Default" w439 {
                    tunnel: [0 ("y") 37 ("y") 17 ("y")] -> w428
                    frame "False", Default {
                    }
                    frame "LNK01E-223429BLF(10DL502HP-D-0)" {
                    }
                    frame "LNK01E-215429BLF(10DL502HP-B-4)" {
                    }
                  }
                  "number 2" <- w428
                  n155 = String Length(string="SERIAL NUMBER HEAD 1") -> (length=w432:i32)
                  "length" <- w432
                  n156 = call "DAQ Assistant"() -> ("data"=w437:bool[])  [unwired: 17 in, 2 out]
                  n157 = Equal?(x=w432, y=w428) -> (x = y?=w431:bool)
                  n158 = Index Array(array=w437, index=0) -> (element=w429:bool)
                  n159 = Not(x=w429) -> (.not. x?=w430:bool)
                  n160 = And(x=w431, y=w430) -> (x .and. y?=w435:bool)
                  n161 = case shown="True" w435 {
                    tunnel: [DualHeadTestStage."CheckHead2" ("DualHeadTestStage") DualHeadTestStage."LoadTestPlanHead1" ("DualHeadTestStage")] -> w434
                    frame False {
                    }
                    frame True {
                    }
                  }
                }
                frame "CheckHead2" {
                  n162 = local read "ProjectFull"() -> (w455:string)
                  n163 = case shown="\"LNK01E-223429BLF(10DL502HP-D-0)\"" w455 {
                    tunnel: [0 ("y") 17 ("y") 37 ("y")] -> w445
                    frame "False", Default {
                    }
                    frame "LNK01E-215429BLF(10DL502HP-B-4)" {
                    }
                    frame "LNK01E-223429BLF(10DL502HP-D-0)" {
                    }
                  }
                  n164 = String Length(string="SERIAL NUMBER HEAD 2") -> (length=w449:i32)
                  n165 = call "DAQ Assistant2"() -> ("data"=w454:bool[])  [unwired: 17 in, 2 out]
                  n166 = Equal?(x=w449, y=w445) -> (x = y?=w448:bool)
                  n167 = Index Array(array=w454, index=0) -> (element=w446:bool)
                  n168 = Not(x=w446) -> (.not. x?=w447:bool)
                  n169 = And(x=w448, y=w447) -> (x .and. y?=w452:bool)
                  n170 = case shown="False" w452 {
                    tunnel: [DualHeadTestStage."CheckHead1" ("DualHeadTestStage") DualHeadTestStage."LoadTestPlanHead2" ("DualHeadTestStage")] -> w451
                    frame False {
                    }
                    frame True {
                    }
                  }
                }
                frame "LoadTestPlanHead1" {
                  n171 = stacked-sequence {
                    tunnel: [_ _ DualHeadTestStage."StartTest" ("DualHeadTestStage")] -> w463
                    frame #0 {
                    }
                    frame #1 {
                    }
                    frame #2 {
                      n172 = flat-sequence {
                        frame #0 {
                          w466 = "" ("Caption.Text")
                          w465 = cluster{u32, u32}[] [{197379, 197379}] ("Colors [4]")
                          n173 = property on="PASS/FAIL STATUS" class="Bool (strict)"("Colors [4]"=w465, "Caption.Text"=w466) -> ()  [unwired: 2 in, 2 out]
                          n174 = property on="PASS/FAIL STATUS  HEAD 1" class="Bool (strict)"("Colors [4]"=w465, "Caption.Text"=w466) -> ()  [unwired: 2 in, 2 out]
                        }
                        frame #1 {
                          n175 = local read "MUX RELAY"() -> (w468:refnum<visa-resource-name>)
                          n176 = call "ControlRelay_ver10.vi"("VISA session"=w468, "write buffer"="Bb000", "Relay Setting"=T4."Manual Cmd") -> ()  [unwired: 10 in, 7 out]
                        }
                        frame #2 {
                          n177 = local write "TESTING HEAD#"("HEAD1" ("TESTING HEAD#")) -> ()
                          "FailedCdDisp H1" <- "" ("FailedCdDisp H1")
                        }
                        frame #3 {
                          n178 = while {
                            i -> [w476]
                            stop <- w473 stop-if-true
                            n179 = Wait (ms)(milliseconds to wait=u32 1) -> ()  [unwired: 1 out]
                            n180 = property on="SERIAL NUMBER HEAD 2" class="Str"("Key Focus"=TRUE) -> ()  [unwired: 2 in, 2 out]
                            n181 = Equal?(x=w476, y=5) -> (x = y?=w473:bool)
                          }
                        }
                      }
                    }
                  }
                }
                frame "LoadTestPlanHead2" {
                  n182 = stacked-sequence {
                    tunnel: [_ _ DualHeadTestStage."StartTest" ("DualHeadTestStage")] -> w478
                    frame #0 {
                    }
                    frame #1 {
                    }
                    frame #2 {
                      n183 = flat-sequence {
                        frame #0 {
                          w481 = "" ("Caption.Text")
                          w480 = cluster{u32, u32}[] [{197379, 197379}] ("Colors [4]")
                          n184 = property on="PASS/FAIL STATUS" class="Bool (strict)"("Colors [4]"=w480, "Caption.Text"=w481) -> ()  [unwired: 2 in, 2 out]
                          n185 = property on="PASS/FAIL STATUS  HEAD 2" class="Bool (strict)"("Colors [4]"=w480, "Caption.Text"=w481) -> ()  [unwired: 2 in, 2 out]
                        }
                        frame #1 {
                          n186 = local read "MUX RELAY"() -> (w483:refnum<visa-resource-name>)
                          n187 = call "ControlRelay_ver10.vi"("VISA session"=w483, "write buffer"="Bb000", "Relay Setting"=T4."Manual Cmd") -> ()  [unwired: 10 in, 7 out]
                        }
                        frame #2 {
                          n188 = local write "TESTING HEAD#"("HEAD2" ("TESTING HEAD#")) -> ()
                          n189 = Wait (ms)(milliseconds to wait=u32 50) -> ()  [unwired: 1 out]
                          "FailedCdDisp H2" <- "" ("FailedCdDisp H2")
                        }
                        frame #3 {
                          n190 = local read "ProjectFull"() -> (w488:string)
                          n191 = case shown="\"LNK01E-223429BLF(10DL502HP-D-0)\"" w488 {
                            frame "False", Default {
                            }
                            frame "LNK01E-213299LF(10DL5H)" {
                              # "SWAP TO TEST HEAD 2"
                              n192 = local read "MUX RELAY"() -> (w490:refnum<visa-resource-name>)
                              n193 = call "ControlRelay_ver10.vi"("VISA session"=w490, "write buffer"="@b041t", "Relay Setting"=T4."Manual Cmd") -> ()  [unwired: 10 in, 7 out]
                            }
                            frame "LNK01E-213300LF(10DL12H)" {
                              # "SWAP TO TEST HEAD 2"
                              n194 = flat-sequence {
                                tunnel: [w494] -> w493
                                tunnel: w493 -> [w498]
                                tunnel: [w498] -> w492
                                tunnel: w492 -> [w499]
                                frame #0 {
                                n195 = local read "MUX RELAY"() -> (w494:refnum<visa-resource-name>)
                                n196 = call "ControlRelay_ver10.vi"("VISA session"=w494, "write buffer"="@b013t", "Relay Setting"=T4."Manual Cmd") -> ()  [unwired: 10 in, 7 out]
                                }
                                frame #1 {
                                n197 = Wait (ms)(milliseconds to wait=u32 1000) -> ()  [unwired: 1 out]
                                }
                                frame #2 {
                                n198 = call "ControlRelay_ver10.vi"("VISA session"=w499, "write buffer"="@b020t", "Relay Setting"=T4."Manual Cmd") -> ()  [unwired: 10 in, 7 out]
                                }
                              }
                            }
                            frame "LNK01E-213300ALF(10DL12H)" {
                              # "SWAP TO TEST HEAD 2"
                              n199 = flat-sequence {
                                tunnel: [w504] -> w503
                                tunnel: w503 -> [w508]
                                tunnel: [w508] -> w502
                                tunnel: w502 -> [w509]
                                frame #0 {
                                n200 = local read "MUX RELAY"() -> (w504:refnum<visa-resource-name>)
                                n201 = call "ControlRelay_ver10.vi"("VISA session"=w504, "write buffer"="@b013t", "Relay Setting"=T4."Manual Cmd") -> ()  [unwired: 10 in, 7 out]
                                }
                                frame #1 {
                                n202 = Wait (ms)(milliseconds to wait=u32 1000) -> ()  [unwired: 1 out]
                                }
                                frame #2 {
                                n203 = call "ControlRelay_ver10.vi"("VISA session"=w509, "write buffer"="@b020t", "Relay Setting"=T4."Manual Cmd") -> ()  [unwired: 10 in, 7 out]
                                }
                              }
                            }
                            frame "LNK01E-215429ALF(10DL502HP)" {
                              # "SWAP TO TEST HEAD 2"
                              n204 = flat-sequence {
                                tunnel: [w515] -> w513
                                tunnel: w513 -> [w519]
                                tunnel: [w519] -> w512
                                tunnel: w512 -> [w521]
                                frame #0 {
                                n205 = local read "MUX RELAY"() -> (w515:refnum<visa-resource-name>)
                                n206 = call "ControlRelay_ver10.vi"("VISA session"=w515, "baud rate (9600)"=u32 19200, "write buffer"="Bb013t", "Relay Setting"=T4."Manual Cmd") -> ()  [unwired: 9 in, 7 out]
                                }
                                frame #1 {
                                n207 = Wait (ms)(milliseconds to wait=u32 1000) -> ()  [unwired: 1 out]
                                }
                                frame #2 {
                                n208 = call "ControlRelay_ver10.vi"("VISA session"=w521, "baud rate (9600)"=u32 19200, "write buffer"="Bb020t", "Relay Setting"=T4."Manual Cmd") -> ()  [unwired: 9 in, 7 out]
                                }
                              }
                            }
                            frame "LNK01E-223429BLF(10DL502HP-D-0)" {
                              # "SWAP TO TEST HEAD 2"
                              n209 = flat-sequence {
                                tunnel: [w527] -> w525
                                tunnel: w525 -> [w531]
                                tunnel: [w531] -> w524
                                tunnel: w524 -> [w533]
                                frame #0 {
                                n210 = local read "MUX RELAY"() -> (w527:refnum<visa-resource-name>)
                                n211 = call "ControlRelay_ver10.vi"("VISA session"=w527, "baud rate (9600)"=u32 19200, "write buffer"="Bb013t", "Relay Setting"=T4."Manual Cmd") -> ()  [unwired: 9 in, 7 out]
                                }
                                frame #1 {
                                n212 = Wait (ms)(milliseconds to wait=u32 1000) -> ()  [unwired: 1 out]
                                }
                                frame #2 {
                                n213 = call "ControlRelay_ver10.vi"("VISA session"=w533, "baud rate (9600)"=u32 19200, "write buffer"="Bb020t", "Relay Setting"=T4."Manual Cmd") -> ()  [unwired: 9 in, 7 out]
                                }
                              }
                            }
                            frame "LNK01E-215429BLF(10DL502HP-B-4)" {
                              # "SWAP TO TEST HEAD 2"
                              n214 = flat-sequence {
                                tunnel: [w539] -> w537
                                tunnel: w537 -> [w543]
                                tunnel: [w543] -> w536
                                tunnel: w536 -> [w545]
                                frame #0 {
                                n215 = local read "MUX RELAY"() -> (w539:refnum<visa-resource-name>)
                                n216 = call "ControlRelay_ver10.vi"("VISA session"=w539, "baud rate (9600)"=u32 19200, "write buffer"="Bb013t", "Relay Setting"=T4."Manual Cmd") -> ()  [unwired: 9 in, 7 out]
                                }
                                frame #1 {
                                n217 = Wait (ms)(milliseconds to wait=u32 1000) -> ()  [unwired: 1 out]
                                }
                                frame #2 {
                                n218 = call "ControlRelay_ver10.vi"("VISA session"=w545, "baud rate (9600)"=u32 19200, "write buffer"="Bb020t", "Relay Setting"=T4."Manual Cmd") -> ()  [unwired: 9 in, 7 out]
                                }
                              }
                            }
                            frame "LNK908-215429LF(10DL501HP)" {
                              # "SWAP TO TEST HEAD 2"
                              n219 = flat-sequence {
                                frame #0 {
                                n220 = local read "MUX RELAY"() -> (w548:refnum<visa-resource-name>)
                                n221 = call "ControlRelay_ver10.vi"("VISA session"=w548, "write buffer"="@b007t", "Relay Setting"=T4."Manual Cmd") -> ()  [unwired: 10 in, 7 out]
                                }
                                frame #1 {
                                n222 = Wait (ms)(milliseconds to wait=u32 1000) -> ()  [unwired: 1 out]
                                }
                                frame #2 {
                                n223 = local read "MUX RELAY"() -> (w554:refnum<visa-resource-name>)
                                n224 = call "ControlRelay_ver10.vi"("VISA session"=w554, "write buffer"="@b013t", "Relay Setting"=T4."Manual Cmd") -> ()  [unwired: 10 in, 7 out]
                                }
                                frame #3 {
                                n225 = Wait (ms)(milliseconds to wait=u32 1000) -> ()  [unwired: 1 out]
                                }
                                frame #4 {
                                n226 = local read "MUX RELAY"() -> (w556:refnum<visa-resource-name>)
                                n227 = call "ControlRelay_ver10.vi"("VISA session"=w556, "write buffer"="@b043t", "Relay Setting"=T4."Manual Cmd") -> ()  [unwired: 10 in, 7 out]
                                }
                              }
                            }
                            frame "LNK01E-213301LF(10DL4H)" {
                              # "SWAP TO TEST HEAD 2"
                              n228 = local read "MUX RELAY"() -> (w560:refnum<visa-resource-name>)
                              n229 = call "ControlRelay_ver10.vi"("VISA session"=w560, "write buffer"="@b042t", "Relay Setting"=T4."Manual Cmd") -> ()  [unwired: 10 in, 7 out]
                            }
                          }
                        }
                        frame #4 {
                          n230 = while {
                            i -> [w565]
                            stop <- w562 stop-if-true
                            n231 = Wait (ms)(milliseconds to wait=u32 1) -> ()  [unwired: 1 out]
                            n232 = property on="SERIAL NUMBER HEAD 1" class="Str"("Key Focus"=TRUE) -> ()  [unwired: 2 in, 2 out]
                            n233 = Equal?(x=w565, y=5) -> (x = y?=w562:bool)
                          }
                        }
                      }
                    }
                  }
                }
                frame "StartTest" {
                  w567 = 0.0
                  n234 = local write "Test Time HEAD 2"(w567) -> ()
                  n235 = local write "Test Time HEAD 1"(w567) -> ()
                  n236 = Enqueue Element(queue=w570, element="BARCODE SCANER") -> ()  [unwired: 1 in, 4 out]
                }
              }
            }
          }
          frame "OPERATOR ID" {
            n237 = flat-sequence {
              tunnel: w572 -> [w626]
              frame #0 {
                n238 = while {
                  stop <- w575 stop-if-true
                  n239 = flat-sequence {
                    tunnel: [w584] -> w576
                    tunnel: w576 -> [w606]
                    tunnel: [w605] -> w574
                    frame #0 {
                      n240 = while {
                        i -> [w582]
                        stop <- w580 stop-if-true
                        n241 = Equal?(x=3, y=w582) -> (x = y?=w580:bool)
                        n242 = property on="Operator ID" class="Str"("Key Focus"=TRUE) -> ()  [unwired: 2 in, 2 out]
                        n243 = Wait (ms)(milliseconds to wait=u32 250) -> ()  [unwired: 1 out]
                      }
                      n244 = local write "Operator ID"("" ("Operator ID")) -> ()
                      n245 = local write "ID STS"(FALSE ("Boolean")) -> ()
                    }
                    frame #1 {
                      n246 = while {
                        tunnel: [w586] -> w584
                        stop <- w587 stop-if-true
                        n247 = local read "SeqFileSts"() -> (w585:bool)
                        n248 = case shown="False" w585 {
                          tunnel: ["ID OK" w590] -> w586
                          frame False {
                          }
                          frame True {
                            n249 = flat-sequence {
                              tunnel: [FALSE ("ID OK")] -> w590
                              frame #0 {
                                n250 = Stop(stop? (T)=TRUE) -> ()
                              }
                              frame #1 {
                              }
                            }
                          }
                        }
                        n251 = local read "Stop_Buffer"() -> (w588:bool)
                        n252 = Or(x=w586, y=w588) -> (x .or. y?=w587:bool)
                      }
                    }
                    frame #2 {
                      n253 = Current VI's Path() -> (path=w594:path)
                      n254 = local read "Operator Mode:"() -> (w607:enum32{"Admin", "Technician", "Operator"})
                      n255 = Strip Path(path=w594) -> (stripped path=w595:path)  [unwired: 1 out]
                      n256 = Build Path(base path=w595, name or relative path="SwConfig") -> (appended path=w598:path)
                      n257 = Build Path(base path=w598, name or relative path="SoftwareConfigulation.txt") -> (appended path=w599:path)
                      n258 = Read from Text File(file (use dialog)=w599) -> (text=w600:string)  [unwired: 1 in, 5 out]
                      n259 = Match Pattern(string=w600, regular expression="OperatorId=" ("name or relative path")) -> (after substring=w602:string)  [unwired: 4 out]
                      n260 = Match Pattern(string=w602, regular expression="\n" ("name or relative path")) -> (before substring=w604:string)  [unwired: 4 out]
                      n261 = Decimal String To Number(string=w604) -> (number=w593:i32)  [unwired: 3 out]
                      n262 = case shown="\"Operator\"" w607 {
                        tunnel: w606 -> [w608 w609 w612]
                        tunnel: [w608 w609 w611] -> w605
                        tunnel: w593 -> [_ _ w610]
                        frame "Admin", Default {
                        }
                        frame "Technician" {
                        }
                        frame "Operator" {
                          n263 = case shown="True" w612 {
                            tunnel: [FALSE w615] -> w611
                            tunnel: w610 -> [_ w614]
                            frame False {
                            }
                            frame True {
                              n264 = local read "Operator ID"() -> (w618:string)
                              n265 = String Length(string=w618) -> (length=w617:i32)
                              n266 = Equal?(x=w617, y=w614) -> (x = y?=w616:bool)
                              n267 = case shown="False" w616 {
                                tunnel: [w619 w623] -> w615
                                frame False {
                                n268 = stacked-sequence {
                                tunnel: [_ _ FALSE] -> w619
                                frame #0 {
                                n269 = One Button Dialog(message="Please enter 5 digits of operator ID!\nFor example : 12345      ") -> ()  [unwired: 2 out]
                                }
                                frame #1 {
                                n270 = local write "ID STS"(FALSE ("Boolean")) -> ()
                                }
                                frame #2 {
                                }
                                }
                                }
                                frame True {
                                n271 = stacked-sequence {
                                tunnel: [_ TRUE] -> w623
                                frame #0 {
                                n272 = local write "ID STS"(TRUE ("Boolean")) -> ()
                                }
                                frame #1 {
                                }
                                }
                                }
                              }
                            }
                          }
                        }
                      }
                    }
                  }
                  n273 = local read "Stop_Buffer"() -> (w573:bool)
                  n274 = Or(x=w574, y=w573) -> (x .or. y?=w575:bool)
                }
              }
              frame #1 {
                n275 = flat-sequence {
                  tunnel: w626 -> [w634]
                  frame #0 {
                    n276 = Wait (ms)(milliseconds to wait=u32 500) -> ()  [unwired: 1 out]
                  }
                  frame #1 {
                    n277 = while {
                      i -> [w632]
                      stop <- w629 stop-if-true
                      n278 = Wait (ms)(milliseconds to wait=u32 1) -> ()  [unwired: 1 out]
                      n279 = property on="SERIAL NUMBER HEAD 1" class="Str"("Key Focus"=TRUE) -> ()  [unwired: 2 in, 2 out]
                      n280 = Equal?(x=w632, y=15) -> (x = y?=w629:bool)
                    }
                  }
                  frame #2 {
                    n281 = local read "Stop_Buffer"() -> (w633:bool)
                    n282 = case shown="False" w633 {
                      tunnel: w634 -> [w636 w637]
                      frame False {
                        (unwired) "BARCODE SCANER" ("element")
                        n283 = Enqueue Element(queue=w636, element="DUAL-HEAD-TESTING") -> ()  [unwired: 1 in, 4 out]
                      }
                      frame True {
                        n284 = Enqueue Element(queue=w637, element="STOP") -> ()  [unwired: 1 in, 4 out]
                      }
                    }
                  }
                }
              }
            }
          }
          frame "BARCODE SCANER" {
            n285 = flat-sequence {
              tunnel: w639 -> [w729]
              frame #0 {
                n286 = case shown="True" FALSE {
                  frame False {
                    n287 = disable-structure shown="Enabled" {
                      frame Disabled {
                        n288 = local read "SERIAL NUMBER HEAD 1"() -> (w649:string)
                        n289 = Empty String/Path?(string/path=w649) -> (empty?=w644:bool)
                        n290 = case shown="True" w644 {
                          tunnel: w649 -> [w654 _]
                          tunnel: [w654 w655] -> w648
                          frame False {
                          }
                          frame True {
                            n291 = local read "SERIAL NUMBER HEAD 2"() -> (w655:string)
                          }
                        }
                        n292 = local read "Username"() -> (w642:string)
                        n293 = call "APIGet-Mis.vi"("SerialNumber"=w648, "OpName"="FCT1", "Operator"=w642, "PopUp"="False", "OcsSever"="OCSAEC") -> ("AllowToTest"=w645:bool, "Message"=w643:string)  [unwired: 9 in, 4 out]
                        n294 = case shown="False" w645 {
                          tunnel: w644 -> [w651 _]
                          tunnel: w643 -> [w650 _]
                          frame False {
                            n295 = case shown="True" w651 {
                              frame False {
                                n296 = local write "SERIAL NUMBER HEAD 1"("" ("SERIAL NUMBER HEAD 1")) -> ()
                              }
                              frame True {
                                n297 = local write "SERIAL NUMBER HEAD 2"("" ("SERIAL NUMBER HEAD 2")) -> ()
                              }
                            }
                            n298 = One Button Dialog(message=w650) -> ()  [unwired: 1 in, 1 out]
                          }
                          frame True {
                          }
                        }
                        n299 = local write "AllowToTest"(w645) -> ()
                      }
                      frame Enabled {
                        n300 = local write "AllowToTest"(TRUE ("AllowToTest")) -> ()
                      }
                    }
                  }
                  frame True {
                    n301 = stacked-sequence {
                      frame #0 {
                        n302 = local read "Test Modes"() -> (w657:enum32{"Auto", "Step"})
                        n303 = case shown="\"Auto\", Default" w657 {
                          frame "Auto", Default {
                            # "OperatorId=5\nSerialNumber=1\nSerialNumber299=1\nSerialNumber300=2\nSerialNumber301=3"
                            n304 = local read "ProjectFull"() -> (w660:string)
                            n305 = Current VI's Path() -> (path=w670:path)
                            n306 = Strip Path(path=w670) -> (stripped path=w669:path)  [unwired: 1 out]
                            n307 = case shown="\"LNK01E-223429BLF(10DL502HP-D-0)\"" w660 {
                              tunnel: ["" ("name or relative path") "SerialNumber299=" ("name or relative path") "SerialNumber299=" ("name or relative path") "SerialNumber300=" ("name or relative path") "SerialNumber300A=" ("name or relative path") "SerialNumber429=" ("name or relative path") "SerialNumber429A=" ("name or relative path") "SerialNumber429B=" ("name or relative path") "SerialNumber429B=" ("name or relative path")] -> w659
                              frame "False", Default {
                              }
                              frame "LNK01E-213299LF(10DL5H)" {
                              }
                              frame "LNK01E-213301LF(10DL4H)" {
                              }
                              frame "LNK01E-213300LF(10DL12H)" {
                              }
                              frame "LNK01E-213300ALF(10DL12H)" {
                              }
                              frame "LNK908-215429LF(10DL501HP)" {
                              }
                              frame "LNK01E-215429ALF(10DL502HP)" {
                              }
                              frame "LNK01E-215429BLF(10DL502HP-B-4)" {
                              }
                              frame "LNK01E-223429BLF(10DL502HP-D-0)" {
                              }
                            }
                            n308 = Build Path(base path=w669, name or relative path="SwConfig") -> (appended path=w666:path)
                            n309 = Build Path(base path=w666, name or relative path="SoftwareConfigulation.txt") -> (appended path=w665:path)
                            n310 = Read from Text File(file (use dialog)=w665) -> (text=w664:string)  [unwired: 1 in, 5 out]
                            "text" <- w664
                            n311 = Match Pattern(string=w664, regular expression=w659) -> (after substring=w663:string)  [unwired: 4 out]
                            n312 = call "BarCode.vi"("BC DIGIT"=1) -> ("Project Model"=→"Project Model":string, "Ok STS"=→"Ok STS":bool, "BarCode_Out"=→"Serial Number":string, "BarCode Exit"=w672:bool)  [unwired: 4 out]
                            n313 = local write "BarCode Exit"(w672) -> ()
                            n314 = Match Pattern(string=w663, regular expression="\n" ("name or relative path")) -> (before substring=w661:string)  [unwired: 4 out]
                            n315 = Decimal String To Number(string=w661) -> ()  [unwired: 4 out]
                          }
                          frame "Step" {
                          }
                        }
                      }
                      frame #1 {
                      }
                      frame #2 {
                      }
                    }
                  }
                }
              }
              frame #1 {
                w684 = "" ("Serial number (Hex)")
                w687 = i8 0 ("FailFlag")
                w685 = "" ("Result")
                w689 = "" ("FailedParam")
                n316 = local write "Serial number (Hex)"(w684) -> ()
                n317 = local write "Check SUM HEX"(w684) -> ()
                n318 = disable-structure shown="Enabled" {
                  frame Disabled {
                    w709 = "" ("Caption.Text")
                    w708 = cluster{u32, u32}[] [{197379, 197379}] ("Colors [4]")
                    n319 = property on="PASS/FAIL STATUS" class="Bool (strict)"("Colors [4]"=w708, "Caption.Text"=w709) -> ()  [unwired: 2 in, 2 out]
                    n320 = stacked-sequence {
                      tunnel: w708 -> [w711 w713]
                      tunnel: w709 -> [w710 w712]
                      frame #0 {
                        n321 = property on="PASS/FAIL STATUS  HEAD 2" class="Bool (strict)"("Colors [4]"=w711, "Caption.Text"=w710) -> ()  [unwired: 2 in, 2 out]
                      }
                      frame #1 {
                        n322 = property on="PASS/FAIL STATUS  HEAD 1" class="Bool (strict)"("Colors [4]"=w713, "Caption.Text"=w712) -> ()  [unwired: 2 in, 2 out]
                      }
                    }
                  }
                  frame Enabled {
                  }
                }
                n323 = stacked-sequence {
                  frame #0 {
                    w715 = 0
                    n324 = Bundle(w715, w715) -> (w714:cluster{i32, i32})  [unwired: 1 out]
                    n325 = property on="TESTPLAN ARRAY Display" class="Tbl (strict)"("Active Cell"=w714, "Index Values"=w714) -> ()  [unwired: 2 in, 2 out]
                    n326 = property on="Summary Display" class="Tbl (strict)"("Active Cell"=w714, "Index Values"=w714) -> ()  [unwired: 2 in, 2 out]
                  }
                  frame #1 {
                    n327 = Initialize Array("" ("Project"), 1000 ("dimension size"), 3 ("dimension size")) -> (→"Test time report":string[][])
                  }
                  frame #2 {
                    w722 = -2 ("disabled index (col)")
                    n328 = Bundle("disabled index (col)"=w722, "disabled index (col)"=w722) -> (w721:T8)  [unwired: 1 out]
                    n329 = property on="TESTPLAN ARRAY Display" class="Tbl (strict)"("Active Cell"=w721, "Cell BG Color"=u32 16448250) -> ()  [unwired: 2 in, 2 out]
                  }
                  frame #3 {
                    w724 = -2
                    n330 = Bundle(w724, w724) -> (w725:cluster{i32, i32})  [unwired: 1 out]
                    n331 = property on="Summary Display" class="Tbl (strict)"("Active Cell"=w725, "Cell BG Color"=u32 16448250) -> ()  [unwired: 2 in, 2 out]
                  }
                }
                n332 = Initialize Array("") -> (w695:string[][])  [unwired: 2 out]
                n333 = property on="Summary Display" class="Tbl (strict)"("Val(Sgnl)"=string[][] [] ("Value (Signaling)")) -> ()  [unwired: 2 in, 2 out]
                n334 = local write "LineLogFile"("" ("LineLogFile")) -> ()
                n335 = local write "UNIT  PASS/FAIL STATUS"("" ("UNIT  PASS/FAIL STATUS TXT")) -> ()
                n336 = Spreadsheet String To Array(delimiter (Tab)="\t", format string="%s", spreadsheet string="", array type (2D Dbl)=w695) -> (array=w697:string[][])
                n337 = local write "Step#"(w689) -> ()
                n338 = local write "Summary Display"(w697) -> ()
                n339 = Format Date/Time String(time format string (%c)="%d/%m/%Y-%H:%M:%S") -> (date/time string=→"StartTime":string)  [unwired: 2 out]
                "TestPlan_Row_Inc" <- 6 ("TestPlan_Row_Inc")
                "Reading >> Sum Disp" <- "" ("Result")
                "Status >> Sum Disp" <- "" ("Status")
                "Test Step# >> Sum Disp" <- "" ("Test Step#>>Sum Disp")
                "All Test Status in Sum Disp" <- "" ("Test Step#>>Sum Disp")
                "SumDisp_Low_Inc" <- 0 ("Summ")
                "LineLogFile" <- "" ("Result")
                "FailedStep" <- w689
                "FailedCdDisp" <- w685
                "Fail Test Param" <- "" ("Project")
                "TestDesc+TestTime" <- w685
                "FailedFlag" <- w687
                "SetDelayResChk" <- w687
                "Index TestTime" <- i16 0 ("Index TestTime")
              }
              frame #2 {
                n340 = local read "Stop_Buffer"() -> (w726:bool)
                n341 = local read "BarCode Exit"() -> (w727:bool)
                n342 = Or(x=w727, y=w726) -> (x .or. y?=w728:bool)
                n343 = case shown="False" w728 {
                  tunnel: w729 -> [w731 w745]
                  frame False {
                    n344 = local read "Test Modes"() -> (w730:enum32{"Auto", "Step"})
                    n345 = case shown="\"Auto\", Default" w730 {
                      tunnel: w731 -> [w739 w743]
                      frame "Auto", Default {
                        n346 = local read "TESTING HEAD#"() -> (w737:string)
                        n347 = case shown="\"HEAD1\"" w737 {
                          tunnel: ["" ("BARCODE HEAD 2") w741 w742] -> w736
                          frame "False", Default {
                          }
                          frame "HEAD1" {
                            n348 = local read "SERIAL NUMBER HEAD 1"() -> (w741:string)
                          }
                          frame "HEAD2" {
                            n349 = local read "SERIAL NUMBER HEAD 2"() -> (w742:string)
                          }
                        }
                        n350 = local write "Serial Number"(w736) -> ()
                        n351 = local read "AllowToTest"() -> (w734:bool)
                        n352 = Tick Count (ms)() -> (millisecond timer value=→"Start Time":u32)
                        n353 = Select(t="START" ("element"), s=w734, f="DUAL-HEAD-TESTING" ("element")) -> (s? t:f=w732:string)
                        n354 = Enqueue Element(queue=w739, element=w732) -> ()  [unwired: 1 in, 4 out]
                      }
                      frame "Step" {
                        n355 = Enqueue Element(queue=w743, element="SINGLE STEP") -> ()  [unwired: 1 in, 4 out]
                      }
                    }
                  }
                  frame True {
                    n356 = Enqueue Element(queue=w745, element="STOP") -> ()  [unwired: 1 in, 4 out]
                  }
                }
              }
            }
          }
          frame "START" {
            w768 = "" ("y")
            n357 = stacked-sequence {
              tunnel: [w844 _] -> w770
              tunnel: [w843 _] -> w751
              frame #0 {
                n358 = flat-sequence {
                  tunnel: [w845] -> w844
                  tunnel: [w864] -> w843
                  frame #0 {
                    n359 = stacked-sequence {
                      tunnel: [w847 _] -> w845
                      frame #0 {
                        n360 = local read "Start Time"() -> (w851:dbl)
                        n361 = Tick Count (ms)() -> (millisecond timer value=w852:u32)
                        n362 = local read "TESTING HEAD#"() -> (w848:string)
                        n363 = Subtract(x=w852, y=w851) -> (x-y=w849:dbl)
                        n364 = Divide(x=w849, y=1000.0) -> (x/y=w846:dbl)
                        "Test Time (Sec)" <- w846
                        n365 = case shown="\"HEAD2\"" w848 {
                          tunnel: [w853 w854 w855] -> w847
                          tunnel: w846 -> [w853 w854 w855]
                          frame "False", Default {
                          }
                          frame "HEAD1" {
                            "Test Time HEAD 1" <- w854
                          }
                          frame "HEAD2" {
                            "Test Time HEAD 2" <- w855
                          }
                        }
                      }
                      frame #1 {
                        w856 = "TESTING" ("Caption.Text")
                        w857 = cluster{u32, u32}[] [{15759887, 15759887}] ("Colors [4]")
                        n366 = local write "UNIT  PASS/FAIL STATUS"(w856) -> ()
                        n367 = property on="PASS/FAIL STATUS" class="Bool (strict)"("Colors [4]"=w857, "Caption.Text"=w856) -> ()  [unwired: 2 in, 2 out]
                        n368 = local read "TESTING HEAD#"() -> (w858:string)
                        n369 = case shown="\"HEAD2\"" w858 {
                          tunnel: w857 -> [_ w860 w862]
                          tunnel: w856 -> [_ w859 w861]
                          frame "False", Default {
                          }
                          frame "HEAD1" {
                            n370 = property on="PASS/FAIL STATUS  HEAD 1" class="Bool (strict)"("Colors [4]"=w860, "Caption.Text"=w859) -> ()  [unwired: 2 in, 2 out]
                          }
                          frame "HEAD2" {
                            n371 = property on="PASS/FAIL STATUS  HEAD 2" class="Bool (strict)"("Colors [4]"=w862, "Caption.Text"=w861) -> ()  [unwired: 2 in, 2 out]
                          }
                        }
                      }
                    }
                  }
                  frame #1 {
                    n372 = local read "TestPlan_Row_Inc"() -> (w864:i32)
                    n373 = Bundle("TestPlan_Row_Inc"=w864, "disabled index (col)"=-2) -> (w866:T9)  [unwired: 1 out]
                    n374 = property on="TESTPLAN ARRAY Display" class="Tbl (strict)"("Active Cell"=w866, "Cell BG Color"=u32 16777224) -> ()  [unwired: 2 in, 2 out]
                  }
                }
              }
              frame #1 {
                n375 = flat-sequence {
                  frame #0 {
                  }
                  frame #1 {
                    n376 = property on="Break step#" class="CmbBox"() -> ("Value"=→"Break Step#":string)  [unwired: 2 in, 2 out]
                  }
                }
              }
            }
            n377 = local read "TESTPLAN ARRAY Display"() -> (w758:string[][])
            n378 = Bundle("TestPlan_Row_Inc"=w751, "disabled index (col)"=0) -> (w804:T9)  [unwired: 1 out]
            n379 = property on="TESTPLAN ARRAY Display" class="Tbl (strict)"("Active Cell"=w804, "Index Values"=w804) -> ()  [unwired: 2 in, 2 out]
            n380 = call "ArrayToElement.vi"("disabled index (row)"=w751, "disabled index (col)"=2, "array"=w758) -> ("element"=w764:string)
            "Description" <- w764
            n381 = call "ArrayToElement.vi"("disabled index (row)"=w751, "disabled index (col)"=0, "array"=w758) -> ("element"=w748:string)
            "Index" <- w748
            n382 = call "ArrayToElement.vi"("disabled index (row)"=w751, "disabled index (col)"=1, "array"=w758) -> ("element"=w765:string)
            "Step#" <- w765
            n383 = call "ArrayToElement.vi"("disabled index (row)"=w751, "disabled index (col)"=3, "array"=w758) -> ("element"=→"FailedCode":string)
            n384 = call "ArrayToElement.vi"("disabled index (row)"=w751, "disabled index (col)"=4, "array"=w758) -> ("element"=w760:string)
            n385 = call "ArrayToElement.vi"("disabled index (row)"=w751, "disabled index (col)"=5, "array"=w758) -> ("element"=w779:string)
            n386 = call "ArrayToElement.vi"("disabled index (row)"=w751, "disabled index (col)"=6, "array"=w758) -> ("element"=w778:string)
            n387 = call "ArrayToElement.vi"("disabled index (row)"=w751, "disabled index (col)"=7, "array"=w758) -> ("element"=→"LowLimit":string)
            n388 = call "ArrayToElement.vi"("disabled index (row)"=w751, "disabled index (col)"=8, "array"=w758) -> ("element"=→"HighLimit":string)
            n389 = call "ArrayToElement.vi"("disabled index (row)"=w751, "disabled index (col)"=9, "array"=w758) -> ("element"=→"Unit":string)
            n390 = call "ArrayToElement.vi"("disabled index (row)"=w751, "disabled index (col)"=11, "array"=w758) -> ("element"=→"TestLoop":string)
            n391 = call "ArrayToElement.vi"("disabled index (row)"=w751, "disabled index (col)"=12, "array"=w758) -> ("element"=w775:string)
            n392 = call "ArrayToElement.vi"("disabled index (row)"=w751, "disabled index (col)"=13, "array"=w758) -> ("element"=→"Remark":string)
            n393 = call "ArrayToElement.vi"("disabled index (row)"=w751, "disabled index (col)"=10, "array"=w758) -> ("element"=→"VAR_TYPE":string)
            n394 = To Upper Case(1:w778) -> (0:w792:string)
            n395 = To Upper Case(1:w760) -> (0:w761:string)
            "Equipment" <- w761
            n396 = Search and Replace String(input string=w775, search string="\"", replace string="" ("replace string (\"\")")) -> (result string=w788:string)  [unwired: 1 in, 7 out]
            n397 = Search and Replace String(input string=w792, search string="\"", replace string="" ("replace string (\"\")")) -> (result string=w797:string)  [unwired: 1 in, 7 out]
            n398 = Search and Replace String(input string=w779, search string="\"", replace string="" ("replace string (\"\")")) -> (result string=w799:string)  [unwired: 1 in, 7 out]
            n399 = Search and Replace String(input string=w788, search string="\"", replace string="" ("replace string (\"\")")) -> (result string=→"COMPST":string)  [unwired: 1 in, 7 out]
            n400 = Search and Replace String(input string=w797, search string="\"", replace string="" ("replace string (\"\")")) -> (result string=w771:string)  [unwired: 1 in, 7 out]
            "Action" <- w771
            n401 = Search and Replace String(input string=w799, search string="\"", replace string="" ("replace string (\"\")")) -> (result string=→"CMD":string)  [unwired: 1 in, 7 out]
            n402 = Decimal String To Number(string=w748) -> (number=w747:i32)  [unwired: 2 in, 1 out]
            n403 = local read "TESTING HEAD#"() -> (w749:string)
            n404 = case shown="\"HEAD2\"" w749 {
              tunnel: w747 -> [_ w814 w815]
              frame "False", Default {
              }
              frame "HEAD1" {
                "HEAD 1" <- w814
              }
              frame "HEAD2" {
                "HEAD 2" <- w815
              }
            }
            n405 = Number To Fractional String(number=w770) -> (F-format string=w767:string)  [unwired: 3 out]
            n406 = local read "TestDesc+TestTime"() -> (w766:string)
            n407 = local read "Break Step#"() -> (w757:string)
            n408 = Equal?(x=w766, y=w768) -> (x = y?=w769:bool)
            n409 = Not Equal?(x=w764, y=w768) -> (x != y?=w791:bool)
            n410 = Equal?(x=w748, y=w757) -> (x = y?=w756:bool)
            n411 = case shown="True" w791 {
              tunnel: w765 -> [_ w885]
              frame False {
              }
              frame True {
                n412 = local read "Description"() -> (w886:string)
                n413 = Concatenate Strings("[", w885, "]", "-", w886) -> (w887:string)
                n414 = local write "Step&Description"(w887) -> ()
              }
            }
            n415 = case shown="\"TEST\"" w771 {
              tunnel: w806 -> [w895 w897 w905 _ w912]
              tunnel: w761 -> [_ w896 _ _ _]
              frame "FALSE", Default {
                n416 = local read "TestPlan_Row_Inc"() -> (w893:i32)
                n417 = Increment(x=w893) -> (x+1=w892:i32)
                n418 = local write "TestPlan_Row_Inc"(w892) -> ()
                n419 = One Button Dialog(message="No action  ?????? ") -> ()  [unwired: 1 in, 1 out]
                n420 = Enqueue Element(queue=w895, element="START") -> ()  [unwired: 1 in, 4 out]
              }
              frame "TEST" {
                n421 = local read "TestPlan_Row_Inc"() -> (w899:i32)
                n422 = Increment(x=w899) -> (x+1=w898:i32)
                n423 = local write "TestPlan_Row_Inc"(w898) -> ()
                n424 = Enqueue Element(queue=w897, element=w896) -> ()  [unwired: 1 in, 4 out]
              }
              frame "STEP" {
                n425 = local read "Description"() -> (w901:string)
                n426 = local read "TestPlan_Row_Inc"() -> (w907:i32)
                n427 = Concatenate Strings("[", w901, "]") -> (w900:string)
                n428 = Increment(x=w907) -> (x+1=w906:i32)
                n429 = local write "Test Step# >> Sum Disp"(w900) -> ()
                n430 = local write "TestPlan_Row_Inc"(w906) -> ()
                n431 = Enqueue Element(queue=w905, element="STATUS DATA") -> ()  [unwired: 1 in, 4 out]
              }
              frame "BREAK" {
              }
              frame "END" {
                n432 = local read "FailedFlag"() -> (w909:i8)
                n433 = Equal?(x=w909, y=i8 0) -> (x = y?=w910:bool)
                n434 = case shown="True" w910 {
                  frame False {
                    w913 = "FAILED" ("Caption.Text")
                    w914 = cluster{u32, u32}[] [{16711680, 16711680}] ("Colors [4]")
                    n435 = local write "PASS/FAIL STATUS"(FALSE ("PASS/FAIL STATUS LED")) -> ()
                    n436 = property on="PASS/FAIL STATUS" class="Bool (strict)"("Colors [4]"=w914, "Caption.Text"=w913) -> ()  [unwired: 2 in, 2 out]
                    n437 = local read "TESTING HEAD#"() -> (w915:string)
                    n438 = local write "UNIT  PASS/FAIL STATUS"(w913) -> ()
                    n439 = case shown="\"HEAD1\"" w915 {
                      tunnel: w914 -> [_ w918 w920]
                      tunnel: w913 -> [_ w917 w919]
                      frame "False", Default {
                      }
                      frame "HEAD1" {
                        n440 = property on="PASS/FAIL STATUS  HEAD 1" class="Bool (strict)"("Colors [4]"=w918, "Caption.Text"=w917) -> ()  [unwired: 2 in, 2 out]
                      }
                      frame "HEAD2" {
                        n441 = property on="PASS/FAIL STATUS  HEAD 2" class="Bool (strict)"("Colors [4]"=w920, "Caption.Text"=w919) -> ()  [unwired: 2 in, 2 out]
                      }
                    }
                  }
                  frame True {
                    w922 = "PASSED" ("Caption.Text")
                    w921 = cluster{u32, u32}[] [{65295, 65295}] ("Colors [4]")
                    n442 = local write "UNIT  PASS/FAIL STATUS"(w922) -> ()
                    n443 = local write "PASS/FAIL STATUS"(TRUE ("PASS/FAIL STATUS LED")) -> ()
                    n444 = local read "TESTING HEAD#"() -> (w923:string)
                    n445 = property on="PASS/FAIL STATUS" class="Bool (strict)"("Colors [4]"=w921, "Caption.Text"=w922) -> ()  [unwired: 2 in, 2 out]
                    n446 = case shown="\"HEAD1\"" w923 {
                      tunnel: w921 -> [_ w926 w928]
                      tunnel: w922 -> [_ w925 w927]
                      frame "False", Default {
                      }
                      frame "HEAD1" {
                        n447 = property on="PASS/FAIL STATUS  HEAD 1" class="Bool (strict)"("Colors [4]"=w926, "Caption.Text"=w925) -> ()  [unwired: 2 in, 2 out]
                      }
                      frame "HEAD2" {
                        n448 = property on="PASS/FAIL STATUS  HEAD 2" class="Bool (strict)"("Colors [4]"=w928, "Caption.Text"=w927) -> ()  [unwired: 2 in, 2 out]
                      }
                    }
                  }
                }
                n449 = Enqueue Element(queue=w912, element="SAVE LOG FILE") -> ()  [unwired: 1 in, 4 out]
              }
            }
            n450 = case shown="False" w769 {
              tunnel: w764 -> [w870 w880]
              tunnel: w767 -> [w869 w879]
              tunnel: [w875 w882] -> w755
              tunnel: w766 -> [w877 _]
              tunnel: [w870 w880] -> w753
              tunnel: [w869 w879] -> w752
              tunnel: [w868 i16 0] -> w754
              frame False {
                n451 = local read "Index TestTime"() -> (w871:i16)
                n452 = Increment(x=w871) -> (x+1=w868:i16)
                n453 = Concatenate Strings(w870, "\t", w869) -> (w876:string)
                n454 = local write "Index TestTime"(w868) -> ()
                n455 = Concatenate Strings(w877, w876) -> (w874:string)
                n456 = Concatenate Strings(w874, "\n" ("string")) -> (w875:string)
              }
              frame True {
                n457 = Concatenate Strings(w880, "\t", w879) -> (w884:string)
                n458 = Concatenate Strings(w884, "\n" ("string")) -> (w882:string)
              }
            }
            n459 = case shown="True" w756 {
              frame False {
              }
              frame True {
                n460 = One Button Dialog(message="BREAK !!!") -> ()  [unwired: 1 in, 1 out]
              }
            }
            n461 = stacked-sequence {
              tunnel: w755 -> [_ _ _]
              tunnel: w754 -> [w816 w821 w828]
              tunnel: w753 -> [w817 _ _]
              tunnel: w752 -> [_ w822 _]
              frame #0 {
                n462 = local read "Test time report"() -> (w819:string[][])
                n463 = Replace Array Subset(array=w819, new element=w817, index (row)=w816, index (col)=0 ("disabled index (col)")) -> (w820:string[][])
                n464 = local write "Test time report"(w820) -> ()
              }
              frame #1 {
                n465 = local read "Test time report"() -> (w824:string[][])
                n466 = Replace Array Subset(array=w824, new element=w822, index (row)=w821, index (col)=1 ("disabled index (col)")) -> (w825:string[][])
                n467 = local write "Test time report"(w825) -> ()
              }
              frame #2 {
                n468 = Equal?(x=w828, y=i16 0) -> (x = y?=w826:bool)
                n469 = case shown="True" w826 {
                  frame False {
                    w840 = 1 ("disabled index (col)")
                    n470 = local read "Test time report"() -> (w841:string[][])
                    n471 = local read "Index TestTime"() -> (w839:i16)
                    n472 = Decrement(x=w839) -> (x-1=w831:i16)
                    n473 = Index Array(array=w841, index (row)=w831, index (col)=w840) -> (element=w838:string)
                    n474 = Index Array(array=w841, index (row)=w839, index (col)=w840) -> (element=w837:string)
                    n475 = Fract/Exp String To Number(string=w837) -> (number=w836:dbl)  [unwired: 4 out]
                    n476 = Fract/Exp String To Number(string=w838) -> (number=w835:dbl)  [unwired: 4 out]
                    n477 = Subtract(x=w836, y=w835) -> (x-y=w834:dbl)
                    n478 = Number To Fractional String(number=w834, precision (6)=i16 5) -> (F-format string=w829:string)  [unwired: 2 out]
                    n479 = Replace Array Subset(array=w841, new element=w829, index (row)=w831, index (col)=2 ("disabled index (col)")) -> (w832:string[][])
                    n480 = local write "Test time report"(w832) -> ()
                  }
                  frame True {
                  }
                }
              }
            }
            n481 = local write "TestDesc+TestTime"(w755) -> ()
          }
          frame "RELAY" {
            n482 = local read "CMD"() -> (w929:string)
            n483 = flat-sequence {
              tunnel: w929 -> [w932]
              tunnel: w930 -> [w941]
              frame #0 {
                n484 = case shown="True" TRUE {
                  tunnel: w932 -> [_ w934]
                  frame False {
                  }
                  frame True {
                    n485 = local read "MUX RELAY"() -> (w935:refnum<visa-resource-name>)
                    n486 = call "ControlRelay_ver10.vi"("VISA session"=w935, "baud rate (9600)"=u32 19200, "write buffer"=w934, "Relay Setting"=T4."Manual Cmd") -> ("Status of Set CMD"=→"Status of Set CMD":bool, "ReturnCMD"=→"Return CMD":string)  [unwired: 9 in, 5 out]
                  }
                }
              }
              frame #1 {
                n487 = case shown="True" TRUE {
                  frame False {
                  }
                  frame True {
                    n488 = Wait (ms)(milliseconds to wait=u32 150) -> ()  [unwired: 1 out]
                  }
                }
              }
              frame #2 {
                n489 = local read "Test Modes"() -> (w942:enum32{"Auto", "Step"})
                n490 = case shown="\"Auto\", Default" w942 {
                  tunnel: w941 -> [w943 w945]
                  frame "Auto", Default {
                    n491 = Enqueue Element(queue=w943, element="START") -> ()  [unwired: 1 in, 4 out]
                  }
                  frame "Step" {
                    n492 = Enqueue Element(queue=w945, element="SINGLE STEP") -> ()  [unwired: 1 in, 4 out]
                  }
                }
              }
            }
          }
          frame "DELAY" {
            n493 = flat-sequence {
              tunnel: w947 -> [w950]
              frame #0 {
                n494 = local read "CMD"() -> (w949:string)
                n495 = Decimal String To Number(string=w949) -> (number=w948:i32)  [unwired: 3 out]
                n496 = Wait (ms)(milliseconds to wait=w948) -> ()  [unwired: 1 out]
              }
              frame #1 {
                n497 = local read "Test Modes"() -> (w951:enum32{"Auto", "Step"})
                n498 = case shown="\"Auto\", Default" w951 {
                  tunnel: w950 -> [w952 w954]
                  frame "Auto", Default {
                    n499 = Enqueue Element(queue=w952, element="START") -> ()  [unwired: 1 in, 4 out]
                  }
                  frame "Step" {
                    n500 = Enqueue Element(queue=w954, element="SINGLE STEP") -> ()  [unwired: 1 in, 4 out]
                  }
                }
              }
            }
          }
          frame "KA6003P" {
            # "OUT0"
            # "OUT1"
            # "ISET1:2.225"
            # "VSET1:20.50"
            n501 = local read "KA6003P"() -> (w957:refnum<visa-resource-name>)
            n502 = local read "CMD"() -> (w956:string)
            n503 = while {
              tunnel: [w966] -> w958
              tunnel: w957 -> [w965]
              tunnel: w956 -> [w963]
              i -> [w962]
              stop <- w960 stop-if-true
              w974 = "?" ("regular expression")
              w972 = u16 0 items=["None"=0, "XON/XOFF"=1, "RTS/CTS"=2, "DTR/DSR"=4] ("flow control")
              w970 = u16 10 items=["1.0"=10, "1.5"=15, "2.0"=20] ("stop bits")
              w969 = u16 0 items=["None", "Odd", "Even", "Mark", "Space"] ("parity")
              n504 = Match Pattern(string=w963, regular expression=w974) -> (match substring=w973:string)  [unwired: 4 out]
              n505 = Equal?(x=w973, y=w974) -> (x = y?=w975:bool)
              n506 = case shown="True" w975 {
                tunnel: [FALSE ("read") TRUE ("read")] -> w966
                tunnel: [u32 0 ("delay before read (ms)") u32 1000 ("delay before read (ms)")] -> w976
                frame False {
                }
                frame True {
                }
              }
              n507 = call "Serial WR Com1.vi"("string to write"=w963, "flow control"=w972, "read"=w966, "write"=TRUE, "delay before read (ms)"=w976, "stop bits"=w970, "parity"=w969, "data bits"=u16 8, "baud rate"=u32 9600, "VISA resource name"=w965) -> ("read string"=w977:string)  [unwired: 1 out]
              n508 = call <vilib>:"Trim Whitespace.vi"("string"=w977) -> ("trimmed string"=w964:string)  [unwired: 1 in]
              n509 = local write "Result"(w964) -> ()
              n510 = stacked-sequence {
                frame #0 {
                  n511 = Wait (ms)(milliseconds to wait=u32 500) -> ()  [unwired: 1 out]
                }
              }
              n512 = Equal?(x=w962, y=2) -> (x = y?=w960:bool)
            }
            n513 = case shown="True" w958 {
              tunnel: w959 -> [w983 w985]
              frame False {
                n514 = Enqueue Element(queue=w983, element="START") -> ()  [unwired: 1 in, 4 out]
              }
              frame True {
                n515 = Enqueue Element(queue=w985, element="COMPARE") -> ()  [unwired: 1 in, 4 out]
              }
            }
          }
          frame "KA3003P" {
            # "OUT0"
            # "OUT1"
            # "ISET1:2.225"
            # "VSET1:20.50"
            n516 = local read "KA3003P"() -> (w988:refnum<visa-resource-name>)
            n517 = local read "CMD"() -> (w987:string)
            n518 = while {
              tunnel: [w997] -> w989
              tunnel: w988 -> [w996]
              tunnel: w987 -> [w994]
              i -> [w993]
              stop <- w991 stop-if-true
              w1005 = "?" ("regular expression")
              w1003 = u16 0 items=["None"=0, "XON/XOFF"=1, "RTS/CTS"=2, "DTR/DSR"=4] ("flow control")
              w1001 = u16 10 items=["1.0"=10, "1.5"=15, "2.0"=20] ("stop bits")
              w1000 = u16 0 items=["None", "Odd", "Even", "Mark", "Space"] ("parity")
              n519 = Match Pattern(string=w994, regular expression=w1005) -> (match substring=w1004:string)  [unwired: 4 out]
              n520 = Equal?(x=w1004, y=w1005) -> (x = y?=w1006:bool)
              n521 = case shown="True" w1006 {
                tunnel: [FALSE ("read") TRUE ("read")] -> w997
                tunnel: [u32 0 ("delay before read (ms)") u32 1000 ("delay before read (ms)")] -> w1007
                frame False {
                }
                frame True {
                }
              }
              n522 = call "Serial WR Com1.vi"("string to write"=w994, "flow control"=w1003, "read"=w997, "write"=TRUE, "delay before read (ms)"=w1007, "stop bits"=w1001, "parity"=w1000, "data bits"=u16 8, "baud rate"=u32 9600, "VISA resource name"=w996) -> ("read string"=w1008:string)  [unwired: 1 out]
              n523 = call <vilib>:"Trim Whitespace.vi"("string"=w1008) -> ("trimmed string"=w995:string)  [unwired: 1 in]
              n524 = local write "Result"(w995) -> ()
              n525 = stacked-sequence {
                frame #0 {
                  n526 = Wait (ms)(milliseconds to wait=u32 500) -> ()  [unwired: 1 out]
                }
              }
              n527 = Equal?(x=w993, y=2) -> (x = y?=w991:bool)
            }
            n528 = case shown="True" w989 {
              tunnel: w990 -> [w1014 w1016]
              frame False {
                n529 = Enqueue Element(queue=w1014, element="START") -> ()  [unwired: 1 in, 4 out]
              }
              frame True {
                n530 = Enqueue Element(queue=w1016, element="COMPARE") -> ()  [unwired: 1 in, 4 out]
              }
            }
          }
          frame "A5116-02" {
            w1030 = u16 0 items=["None"=0, "XON/XOFF"=1, "RTS/CTS"=2, "DTR/DSR"=4] ("flow control")
            w1026 = u16 10 items=["1.0"=10, "1.5"=15, "2.0"=20] ("stop bits")
            w1025 = u16 0 items=["None", "Odd", "Even", "Mark", "Space"] ("parity")
            n531 = local read "A5116-02"() -> (w1020:refnum<visa-resource-name>)
            n532 = local read "CMD"() -> (w1021:string)
            n533 = Concatenate Strings(w1021, "\r\n") -> (w1032:string)
            n534 = call "Serial WR Com1.vi"("string to write"=w1032, "flow control"=w1030, "read"=TRUE, "write"=TRUE, "delay before read (ms)"=u32 40, "stop bits"=w1026, "parity"=w1025, "data bits"=u16 8, "baud rate"=u32 9600, "VISA resource name"=w1020) -> ("read string"=w1033:string)  [unwired: 1 out]
            n535 = call <vilib>:"Trim Whitespace.vi"("string"=w1033) -> ("trimmed string"=w1022:string)  [unwired: 1 in]
            n536 = local write "Result"(w1022) -> ()
            n537 = Enqueue Element(queue=w1018, element="COMPARE") -> ()  [unwired: 1 in, 4 out]
          }
          frame "A5114-12" {
            w1041 = "<=" ("regular expression")
            n538 = local read "A5114-12"() -> (w1037:refnum<visa-resource-name>)
            n539 = call "A5114-2.vi"("device_id"=u8 23, "Comport"=w1037) -> ("Volt_data"=w1039:string)  [unwired: 9 out]
            n540 = Match Pattern(string=w1039, regular expression=w1041) -> (match substring=w1042:string)  [unwired: 4 out]
            n541 = Equal?(x=w1042, y=w1041) -> (x = y?=w1040:bool)
            n542 = case shown="False" w1040 {
              tunnel: [w1044 "OPEN" ("Volt_data")] -> w1038
              tunnel: w1039 -> [w1044 _]
              frame False {
              }
              frame True {
              }
            }
            n543 = call <vilib>:"Trim Whitespace.vi"("string"=w1038) -> ("trimmed string"=w1036:string)  [unwired: 1 in]
            n544 = local write "Result"(w1036) -> ()
            n545 = Enqueue Element(queue=w1034, element="COMPARE") -> ()  [unwired: 1 in, 4 out]
          }
          frame "NXT_MV_E100" {
            n546 = local read "CMD"() -> (w1047:string)
            n547 = case shown="\"ReadZLatch1\"" w1047 {
              tunnel: w1046 -> [_ w1048 w1053 w1065 w1080 w1082 w1093 w1105 w1110 w1115 w1120 w1125 w1130 w1135 w1140 w1145 w1150]
              frame "False", Default {
              }
              frame "SetUSBlink-ChkBuild&FwVer" {
                n548 = call "SetUSB-LINK&ChkBuild-FwVer.vi"() -> ("Error?"=→"Result(Boolean) 1":bool, "AAABuild"=→"Result(Number)":i32, "FirmwareVersion"=→"Result(string)":string)  [unwired: 11 in, 2 out]
                n549 = Enqueue Element(queue=w1048, element="START") -> ()  [unwired: 1 in, 4 out]
              }
              frame "DRIVE_ENABLE2" {
                n550 = while {
                  i -> [w1059]
                  stop <- w1060 stop-if-true
                  n551 = call "PBI_MFA_Interface_DriveEnable2.vi"() -> ("DriveEnableStatus"=w1055:bool, "DriveEnableError"=w1063:bool)  [unwired: 10 in]
                  n552 = Not(x=w1055) -> (.not. x?=w1056:bool)
                  n553 = Equal?(x=w1055, y=TRUE) -> (x = y?=w1061:bool)
                  n554 = Equal?(x=w1059, y=2) -> (x = y?=w1057:bool)
                  n555 = local write "Result(Boolean) 3"(w1063) -> ()
                  n556 = local write "Result(Boolean) 4"(w1056) -> ()
                  n557 = Or(x=w1061, y=w1057) -> (x .or. y?=w1060:bool)
                  n558 = flat-sequence {
                    frame #0 {
                      n559 = Wait (ms)(milliseconds to wait=u32 300) -> ()  [unwired: 1 out]
                    }
                  }
                }
                n560 = Enqueue Element(queue=w1053, element="START") -> ()  [unwired: 1 in, 4 out]
              }
              frame "DRIVE_ENABLE2-Axis1" {
                n561 = while {
                  i -> [w1071]
                  stop <- w1072 stop-if-true
                  n562 = call "PBI_MFA_Interface_DriveEnable2-Axis1.vi"() -> ("DriveEnableStatus"=w1067:bool, "DriveEnableError"=w1075:bool)  [unwired: 10 in]
                  n563 = Not(x=w1067) -> (.not. x?=w1068:bool)
                  n564 = Equal?(x=w1067, y=TRUE) -> (x = y?=w1073:bool)
                  n565 = Equal?(x=w1071, y=2) -> (x = y?=w1069:bool)
                  n566 = local write "Result(Boolean) 3"(w1075) -> ()
                  n567 = local write "Result(Boolean) 4"(w1068) -> ()
                  n568 = Or(x=w1073, y=w1069) -> (x .or. y?=w1072:bool)
                  n569 = flat-sequence {
                    frame #0 {
                      n570 = Wait (ms)(milliseconds to wait=u32 300) -> ()  [unwired: 1 out]
                    }
                  }
                }
                n571 = Enqueue Element(queue=w1065, element="START") -> ()  [unwired: 1 in, 4 out]
              }
              frame "ENC0-SET-ZERO" {
                n572 = call "FB_MFA_Set_Position1Enc0 -NxtMve.vi"("Position Put"=sgl 0.0) -> ("Position Get"=w1077:sgl, "SetPositionError"=w1078:bool)  [unwired: 9 in]
                n573 = local write "Result(Boolean) 1"(w1078) -> ()
                n574 = local write "Result(DecimalPoint)"(w1077) -> ()
                n575 = Enqueue Element(queue=w1080, element="START") -> ()  [unwired: 1 in, 4 out]
              }
              frame "ReadZLatch0" {
                n576 = while {
                  i -> [w1090]
                  stop <- w1088 stop-if-true
                  n577 = call "FB_MFA_Read_Z_Latch1 - NxtMv.vi"() -> ("EncoderZLatch"=w1086:bool)  [unwired: 11 in]
                  n578 = Equal?(x=w1086, y=FALSE) -> (x = y?=w1084:bool)
                  n579 = Not(x=w1086) -> (.not. x?=w1091:bool)
                  n580 = local write "Result(Boolean) 1"(w1091) -> ()
                  n581 = Equal?(x=w1090, y=3) -> (x = y?=w1087:bool)
                  n582 = flat-sequence {
                    frame #0 {
                      n583 = Wait (ms)(milliseconds to wait=u32 350) -> ()  [unwired: 1 out]
                    }
                  }
                  n584 = Or(x=w1084, y=w1087) -> (x .or. y?=w1088:bool)
                }
                n585 = Enqueue Element(queue=w1082, element="START") -> ()  [unwired: 1 in, 4 out]
              }
              frame "ReadZLatch1" {
                n586 = while {
                  i -> [w1101]
                  stop <- w1099 stop-if-true
                  n587 = call "FB_MFA_Read_Z_Latch1 - NxtMv.vi"() -> ("EncoderZLatch"=w1097:bool)  [unwired: 11 in]
                  n588 = Equal?(x=w1097, y=TRUE) -> (x = y?=w1095:bool)
                  n589 = Not(x=w1097) -> (.not. x?=w1102:bool)
                  n590 = local write "Result(Boolean) 1"(w1102) -> ()
                  n591 = Equal?(x=w1101, y=3) -> (x = y?=w1098:bool)
                  n592 = flat-sequence {
                    frame #0 {
                      n593 = Wait (ms)(milliseconds to wait=u32 350) -> ()  [unwired: 1 out]
                    }
                  }
                  n594 = Or(x=w1095, y=w1098) -> (x .or. y?=w1099:bool)
                }
                n595 = Enqueue Element(queue=w1093, element="START") -> ()  [unwired: 1 in, 4 out]
              }
              frame "Enc0-Read" {
                n596 = call "FB_MFA_Read_Position_ENC.vi"() -> ("Position Get"=w1104:sgl)  [unwired: 11 in]
                n597 = local write "Result(DecimalPoint)"(w1104) -> ()
                n598 = Enqueue Element(queue=w1105, element="START") -> ()  [unwired: 1 in, 4 out]
              }
              frame "STEPPER-MOVE(56000)" {
                n599 = call "FB_MFA_StepperMove -NxtMv.vi"("Position Put"=sgl 56000.0) -> ("DoGOError"=w1107:bool, "SetMoveError"=w1108:bool)  [unwired: 9 in]
                n600 = local write "Result(Boolean) 1"(w1108) -> ()
                n601 = local write "Result(Boolean) 2"(w1107) -> ()
                n602 = Enqueue Element(queue=w1110, element="START") -> ()  [unwired: 1 in, 4 out]
              }
              frame "STEPPER-MOVE(56000)-Axis1" {
                n603 = call "FB_MFA_StepperMove -NxtMv Axis1.vi"("Position Put"=sgl 56000.0) -> ("DoGOError"=w1112:bool, "SetMoveError"=w1113:bool)  [unwired: 9 in]
                n604 = local write "Result(Boolean) 1"(w1113) -> ()
                n605 = local write "Result(Boolean) 2"(w1112) -> ()
                n606 = Enqueue Element(queue=w1115, element="START") -> ()  [unwired: 1 in, 4 out]
              }
              frame "STEPPER-MOVE(-56000)" {
                n607 = call "FB_MFA_StepperMove -NxtMv.vi"("Position Put"=sgl -56000.0) -> ("DoGOError"=w1117:bool, "SetMoveError"=w1118:bool)  [unwired: 9 in]
                n608 = local write "Result(Boolean) 1"(w1118) -> ()
                n609 = local write "Result(Boolean) 2"(w1117) -> ()
                n610 = Enqueue Element(queue=w1120, element="START") -> ()  [unwired: 1 in, 4 out]
              }
              frame "STEPPER-MOVE(-56000)-Axis1" {
                n611 = call "FB_MFA_StepperMove -NxtMv Axis1.vi"("Position Put"=sgl -56000.0) -> ("DoGOError"=w1122:bool, "SetMoveError"=w1123:bool)  [unwired: 9 in]
                n612 = local write "Result(Boolean) 1"(w1123) -> ()
                n613 = local write "Result(Boolean) 2"(w1122) -> ()
                n614 = Enqueue Element(queue=w1125, element="START") -> ()  [unwired: 1 in, 4 out]
              }
              frame "STEPPER-MOVE(4500)" {
                n615 = call "FB_MFA_StepperMove -NxtMv.vi"("Position Put"=sgl 4500.0) -> ("DoGOError"=w1128:bool, "SetMoveError"=w1129:bool)  [unwired: 9 in]
                n616 = local write "Result(Boolean) 1"(w1129) -> ()
                n617 = local write "Result(Boolean) 2"(w1128) -> ()
                n618 = Enqueue Element(queue=w1130, element="START") -> ()  [unwired: 1 in, 4 out]
              }
              frame "STEPPER-MOVE(9000)" {
                n619 = call "FB_MFA_StepperMove -NxtMv.vi"("Position Put"=sgl 9000.0) -> ("DoGOError"=w1133:bool, "SetMoveError"=w1134:bool)  [unwired: 9 in]
                n620 = local write "Result(Boolean) 1"(w1134) -> ()
                n621 = local write "Result(Boolean) 2"(w1133) -> ()
                n622 = Enqueue Element(queue=w1135, element="START") -> ()  [unwired: 1 in, 4 out]
              }
              frame "STEPPER-MOVE(13500)" {
                n623 = call "FB_MFA_StepperMove -NxtMv.vi"("Position Put"=sgl 13500.0) -> ("DoGOError"=w1138:bool, "SetMoveError"=w1139:bool)  [unwired: 9 in]
                n624 = local write "Result(Boolean) 1"(w1139) -> ()
                n625 = local write "Result(Boolean) 2"(w1138) -> ()
                n626 = Enqueue Element(queue=w1140, element="START") -> ()  [unwired: 1 in, 4 out]
              }
              frame "STEPPER-MOVE(18000)" {
                n627 = call "FB_MFA_StepperMove -NxtMv.vi"("Position Put"=sgl 18000.0) -> ("DoGOError"=w1143:bool, "SetMoveError"=w1144:bool)  [unwired: 9 in]
                n628 = local write "Result(Boolean) 1"(w1144) -> ()
                n629 = local write "Result(Boolean) 2"(w1143) -> ()
                n630 = Enqueue Element(queue=w1145, element="START") -> ()  [unwired: 1 in, 4 out]
              }
              frame "STEPPER-MOVE(22500)" {
                n631 = call "FB_MFA_StepperMove -NxtMv.vi"("Position Put"=sgl 22500.0) -> ("DoGOError"=w1148:bool, "SetMoveError"=w1149:bool)  [unwired: 9 in]
                n632 = local write "Result(Boolean) 1"(w1149) -> ()
                n633 = local write "Result(Boolean) 2"(w1148) -> ()
                n634 = Enqueue Element(queue=w1150, element="START") -> ()  [unwired: 1 in, 4 out]
              }
            }
          }
          frame "MICRO_FLEX" {
            n635 = local read "CMD"() -> (w1153:string)
            n636 = case shown="\"Com&StsCheck\"" w1153 {
              tunnel: w1152 -> [_ w1157 w1159 w1161 w1163 w1165 w1168 w1170 w1181 w1201 w1206 w1211 w1216 w1221 w1229 w1235 w1237 w1242 w1249 w1255 w1257 w1262 w1275 w1293 w1299 w1303 w1308 w1313 w1318 w1320 w1331 w1343 w1346 w1348 w1351 w1357 w1361]
              frame "False", Default {
              }
              frame "Com&StsCheck" {
                n637 = call "CS_MFA_Coms_and_Status_Check.vi"() -> ("Temperature"=→"Result(DecimalPoint)2":sgl, "DriveRatedCurrent"=w1155:sgl, "AAABuild"=w1156:i32)  [unwired: 9 in]
                n638 = local write "Result(Number)"(w1156) -> ()
                n639 = local write "Result(DecimalPoint)"(w1155) -> ()
                n640 = Enqueue Element(queue=w1157, element="START") -> ()  [unwired: 1 in, 4 out]
              }
              frame "LED_D2_OFF" {
                n641 = call "CS_MFA_LED_Status_D2-OFF.vi"() -> ()  [unwired: 12 in]
                n642 = Enqueue Element(queue=w1159, element="START") -> ()  [unwired: 1 in, 4 out]
              }
              frame "LED_D2_GREEN" {
                n643 = call "CS_MFA_LED_Status_D2-GREEN.vi"() -> ()  [unwired: 12 in]
                n644 = Enqueue Element(queue=w1161, element="START") -> ()  [unwired: 1 in, 4 out]
              }
              frame "LED_D2_RED" {
                n645 = call "CS_MFA_LED_Status_D2-RED.vi"() -> ()  [unwired: 12 in]
                n646 = Enqueue Element(queue=w1163, element="START") -> ()  [unwired: 1 in, 4 out]
              }
              frame "LED_D2_FLASH" {
                n647 = call "CS_MFA_LED_Status_D2-FLASH.vi"() -> ()  [unwired: 12 in]
                n648 = Enqueue Element(queue=w1165, element="START") -> ()  [unwired: 1 in, 4 out]
              }
              frame "DCBUS_MEAS" {
                n649 = call "PBI_MFA_Interface_DriveBusVolts1.vi"() -> ("DriveBusVolts_0V"=w1167:sgl)  [unwired: 11 in]
                n650 = local write "Result(DecimalPoint)"(w1167) -> ()
                n651 = Enqueue Element(queue=w1168, element="COMPARE") -> ()  [unwired: 1 in, 4 out]
              }
              frame "DRIVE-AXIS_ERROR" {
                n652 = while {
                  i -> [w1175]
                  stop <- w1173 stop-if-true
                  n653 = call "DriveEN.vi"() -> ("AxisError"=→"Result(Number)2":i32, "DriveError"=w1178:i16, "DoCancleErrorStatus"=w1177:bool)  [unwired: 9 in]
                  n654 = local write "Result(Boolean) 1"(w1177) -> ()
                  n655 = local write "Result(Number)"(w1178) -> ()
                  n656 = Equal?(x=w1175, y=1) -> (x = y?=w1172:bool)
                  n657 = flat-sequence {
                    tunnel: [w1180] -> w1173
                    tunnel: w1172 -> [w1180]
                    frame #0 {
                      n658 = Wait (ms)(milliseconds to wait=u32 1000) -> ()  [unwired: 1 out]
                    }
                  }
                }
                n659 = Enqueue Element(queue=w1170, element="START") -> ()  [unwired: 1 in, 4 out]
              }
              frame "DRIVE-ENABLE" {
                n660 = while {
                  i -> [w1188]
                  stop <- w1185 stop-if-true
                  n661 = Equal?(x=w1188, y=1) -> (x = y?=w1186:bool)
                  n662 = call "PBI_MFA_Interface_DriveEnable1.vi"() -> ("DriveEnableStatus"=w1192:bool, "DriveEnableError"=w1194:bool, "DoCancleError"=→"Result(Boolean) 2":bool, "BurnInError"=w1197:bool)  [unwired: 8 in]
                  "Result(Boolean) 3" <- w1194
                  n663 = Not(x=w1192) -> (.not. x?=→"Result(Boolean) 4":bool)
                  n664 = local write "Result(Boolean) 1"(w1197) -> ()
                  n665 = Not Equal?(x=w1194, y=TRUE) -> (x != y?=w1190:bool)
                  n666 = Not Equal?(x=w1192, y=FALSE) -> (x != y?=w1189:bool)
                  n667 = And(x=w1190, y=w1189) -> (x .and. y?=w1184:bool)
                  n668 = case shown="False" w1184 {
                    selector: w1184 -> [w1198 w1200]
                    tunnel: [w1198 w1200] -> w1183
                    frame False {
                      n669 = Wait (ms)(milliseconds to wait=u32 500) -> ()  [unwired: 1 out]
                    }
                    frame True {
                    }
                  }
                  n670 = Or(x=w1183, y=w1186) -> (x .or. y?=w1185:bool)
                }
                n671 = Enqueue Element(queue=w1181, element="START") -> ()  [unwired: 1 in, 4 out]
              }
              frame "PWM-NEW_VAL=1" {
                w1204 = FALSE ("newValue2")
                n672 = call "PBI_MFA_Interface_PWM_Signals1.vi"("newValue0"=w1204, "newValue3"=w1204, "newValue2"=w1204, "newValue 1"=TRUE) -> ("MotTstMd1"=w1203:bool)  [unwired: 4 in, 3 out]
                n673 = local write "Result(Boolean) 1"(w1203) -> ()
                n674 = Enqueue Element(queue=w1201, element="START") -> ()  [unwired: 1 in, 4 out]
              }
              frame "PWM-NEW_VAL=2" {
                w1209 = FALSE ("newValue 1")
                n675 = call "PBI_MFA_Interface_PWM_Signals1.vi"("newValue0"=w1209, "newValue3"=w1209, "newValue2"=TRUE, "newValue 1"=w1209) -> ("MotTstMd2"=w1208:bool)  [unwired: 4 in, 3 out]
                n676 = local write "Result(Boolean) 1"(w1208) -> ()
                n677 = Enqueue Element(queue=w1206, element="START") -> ()  [unwired: 1 in, 4 out]
              }
              frame "PWM-NEW_VAL=3" {
                w1214 = FALSE ("newValue 1")
                n678 = call "PBI_MFA_Interface_PWM_Signals1.vi"("newValue0"=w1214, "newValue3"=TRUE ("newValue2"), "newValue2"=w1214, "newValue 1"=w1214) -> ("MotTstMd3"=w1213:bool)  [unwired: 4 in, 3 out]
                n679 = local write "Result(Boolean) 1"(w1213) -> ()
                n680 = Enqueue Element(queue=w1211, element="START") -> ()  [unwired: 1 in, 4 out]
              }
              frame "PWM-NEW_VAL=0" {
                w1219 = FALSE ("newValue 1")
                n681 = call "PBI_MFA_Interface_PWM_Signals1.vi"("newValue0"=TRUE ("newValue2"), "newValue3"=w1219, "newValue2"=w1219, "newValue 1"=w1219) -> ("MotTstMd0"=w1218:bool)  [unwired: 4 in, 3 out]
                n682 = local write "Result(Boolean) 1"(w1218) -> ()
                n683 = Enqueue Element(queue=w1216, element="START") -> ()  [unwired: 1 in, 4 out]
              }
              frame "DRIVE-DISABLE" {
                n684 = call "PBI_MFA_Interface_DriveDisable.vi"() -> ("DriveEnable"=w1225:bool, "status"=w1223:bool)  [unwired: 10 in]
                "DriveEnable" <- w1225
                n685 = Not(x=w1225) -> (.not. x?=w1224:bool)
                n686 = local write "Result(Boolean) 1"(w1223) -> ()
                n687 = local write "Result(Boolean) 2"(w1224) -> ()
                n688 = Enqueue Element(queue=w1221, element="START") -> ()  [unwired: 1 in, 4 out]
              }
              frame "FAC_DEF" {
                n689 = call "PBI_MFA_Interface_IACT_InitialSetup1_DefaultFactory.vi"("Meas Curr"=FALSE, "FacDefault"=TRUE) -> ("FactoryDefaultError"=w1228:bool)  [unwired: 7 in, 2 out]
                n690 = local write "Result(Boolean) 1"(w1228) -> ()
                n691 = Enqueue Element(queue=w1229, element="START") -> ()  [unwired: 1 in, 4 out]
              }
              frame "IACT_U&IACT_V" {
                n692 = call "PBI_MFA_Interface_IACT_InitialSetup1_DefaultFactory.vi"("Meas Curr"=TRUE, "FacDefault"=FALSE) -> ("CurrentMeas2_at5V"=w1231:sgl, "CurrentMeas1_at5V"=w1232:sgl)  [unwired: 7 in, 1 out]
                n693 = local write "Result(DecimalPoint)2"(w1231) -> ()
                n694 = local write "Result(DecimalPoint)"(w1232) -> ()
                n695 = Enqueue Element(queue=w1235, element="START") -> ()  [unwired: 1 in, 4 out]
              }
              frame "DriveEnableSwitch" {
                n696 = call "IO_MFA_DIN_Read_DigitalInput_DriveEnableSwitch.vi"() -> ("DriveEnableSwitch"=w1240:bool)  [unwired: 11 in]
                n697 = Not(x=w1240) -> (.not. x?=w1239:bool)
                n698 = local write "Result(Boolean) 1"(w1239) -> ()
                n699 = Enqueue Element(queue=w1237, element="COMPARE") -> ()  [unwired: 1 in, 4 out]
              }
              frame "InStateX" {
                n700 = call "IO_MFA_DIN_Read_DigitalInput_InStateX.vi"() -> ("DriveEnableSwitch"=w1241:bool)  [unwired: 11 in]
                n701 = Not(x=w1241) -> (.not. x?=w1244:bool)
                n702 = local write "Result(Boolean) 1"(w1244) -> ()
                n703 = Enqueue Element(queue=w1242, element="COMPARE") -> ()  [unwired: 1 in, 4 out]
              }
              frame "OutputActiveLevel0" {
                n704 = call "IO_MFA_DOUT_Read_DigitalOutput1.vi"("O/P Actlevel1"=FALSE, "O/P Actlevel0"=TRUE) -> ("OutputActiveLevel 0"=w1245:i32, "ErrorActLvl0"=w1246:bool)  [unwired: 6 in, 2 out]
                n705 = local write "Result(Boolean) 1"(w1246) -> ()
                n706 = local write "Result(Number)"(w1245) -> ()
                n707 = Enqueue Element(queue=w1249, element="START") -> ()  [unwired: 1 in, 4 out]
              }
              frame "OutputActiveLevel1" {
                n708 = call "IO_MFA_DOUT_Read_DigitalOutput1.vi"("O/P Actlevel1"=TRUE, "O/P Actlevel0"=FALSE) -> ("OutputActiveLevel 1"=w1252:i32, "ErrorActLvl1"=w1251:bool)  [unwired: 6 in, 2 out]
                n709 = local write "Result(Boolean) 1"(w1251) -> ()
                n710 = local write "Result(Number)"(w1252) -> ()
                n711 = Enqueue Element(queue=w1255, element="START") -> ()  [unwired: 1 in, 4 out]
              }
              frame "PulseCounterBe" {
                n712 = flat-sequence {
                  frame #0 {
                    w1259 = ""
                    n713 = local write "LowLimitForIntValue"(w1259) -> ()
                    n714 = local write "HighLimitForIntValue"(w1259) -> ()
                  }
                  frame #1 {
                    n715 = call "IO_MFA_StepDir_Read_PulseCount1.vi"() -> ("PulseCounter Init"=w1261:i32)  [unwired: 11 in]
                    "InitialValue" <- w1261
                    n716 = Number To Decimal String(number=w1261) -> (decimal integer string=→"HighLimitForIntValue" →"LowLimitForIntValue":string)  [unwired: 1 in]
                    n717 = local write "Result(Number)"(w1261) -> ()
                  }
                }
                n718 = Enqueue Element(queue=w1257, element="START") -> ()  [unwired: 1 in, 4 out]
              }
              frame "PulseCounterAf" {
                n719 = while {
                  i -> [w1269]
                  stop <- w1264 stop-if-true
                  n720 = call "IO_MFA_StepDir_Read_PulseCount1.vi"() -> ("PulseCounter Init"=w1271:i32)  [unwired: 11 in]
                  "InitialValueAfter" <- w1271
                  n721 = Less Or Equal?(x=w1271, y=1) -> (x <= y?=w1267:bool)
                  n722 = local write "Result(Number)"(w1271) -> ()
                  n723 = Equal?(x=w1269, y=7) -> (x = y?=w1266:bool)
                  n724 = Or(x=w1267, y=w1266) -> (x .or. y?=w1265:bool)
                  n725 = flat-sequence {
                    tunnel: [w1273] -> w1264
                    tunnel: w1265 -> [w1273]
                    frame #0 {
                      n726 = Wait (ms)(milliseconds to wait=u32 800) -> ()  [unwired: 1 out]
                    }
                  }
                }
                n727 = Enqueue Element(queue=w1262, element="START") -> ()  [unwired: 1 in, 4 out]
              }
              frame "PulseCounter+400" {
                w1274 = ""
                n728 = local write "HighLimitForPulseCnt+400"(w1274) -> ()
                n729 = local write "LowLimitForPulseCnt+400"(w1274) -> ()
                n730 = while {
                  tunnel: w1274 -> [_]
                  i -> [w1286]
                  stop <- w1281 stop-if-true
                  n731 = local read "InitialValue"() -> (w1280:i32)
                  n732 = call "IO_MFA_StepDir_Read_PulseCount1.vi"() -> ("PulseCounter Init"=w1289:i32)  [unwired: 11 in]
                  n733 = Add(x=w1280, y=w1289) -> (x+y=w1288:i32)
                  n734 = Add(x=w1280, y=400) -> (x+y=w1278:i32)
                  n735 = Greater Or Equal?(x=w1288, y=400) -> (x >= y?=w1283:bool)
                  n736 = Number To Decimal String(number=w1278) -> (decimal integer string=→"HighLimitForPulseCnt+400" →"LowLimitForPulseCnt+400":string)  [unwired: 1 in]
                  n737 = local write "Result(Number)"(w1288) -> ()
                  n738 = Equal?(x=w1286, y=7) -> (x = y?=w1284:bool)
                  n739 = Or(x=w1283, y=w1284) -> (x .or. y?=w1282:bool)
                  n740 = flat-sequence {
                    tunnel: w1282 -> [w1291]
                    tunnel: [w1291] -> w1281
                    frame #0 {
                      n741 = Wait (ms)(milliseconds to wait=u32 1000) -> ()  [unwired: 1 out]
                    }
                  }
                }
                n742 = Enqueue Element(queue=w1275, element="START") -> ()  [unwired: 1 in, 4 out]
              }
              frame "ADC" {
                n743 = call "IO_MFA_AIN_Read_AnalogueInput1.vi"() -> ("ADC"=w1292:sgl)  [unwired: 11 in]
                "ADC val" <- w1292
                n744 = local write "Result(DecimalPoint)"(w1292) -> ()
                n745 = Enqueue Element(queue=w1293, element="COMPARE") -> ()  [unwired: 1 in, 4 out]
              }
              frame "ADCOffset" {
                n746 = local read "ADC val"() -> (w1297:sgl)
                n747 = Multiply(x=w1297, y=sgl -1.0) -> (x*y=w1296:sgl)
                n748 = call "IO_MFA_AIN_Set_AdcOffset1.vi"("AdcOffset"=w1296) -> ("ADC Offset Error"=w1298:bool)  [unwired: 10 in]
                n749 = local write "Result(Boolean) 1"(w1298) -> ()
                n750 = Enqueue Element(queue=w1299, element="COMPARE") -> ()  [unwired: 1 in, 4 out]
              }
              frame "ADCOffsetZero" {
                n751 = call "IO_MFA_AIN_Set_AdcOffset1.vi"("AdcOffset"=sgl 0.0) -> ("ADC Offset Error"=w1302:bool)  [unwired: 10 in]
                n752 = local write "Result(Boolean) 1"(w1302) -> ()
                n753 = Enqueue Element(queue=w1303, element="COMPARE") -> ()  [unwired: 1 in, 4 out]
              }
              frame "MOT_FB" {
                n754 = call "FB_MFA_SetMotorFeedback_Type1.vi"("SetMotorFeedbackType"=i16 1) -> ("MotorFeedback"=w1305:i16, "MotFbError"=w1306:bool)  [unwired: 9 in]
                n755 = local write "Result(Number)"(w1305) -> ()
                n756 = local write "Result(Boolean) 1"(w1306) -> ()
                n757 = Enqueue Element(queue=w1308, element="START") -> ()  [unwired: 1 in, 4 out]
              }
              frame "MOT_FB_SSI" {
                n758 = call "FB_MFA_SetMotorFeedback_Type1.vi"("SetMotorFeedbackType"=i16 10) -> ("MotorFeedback"=w1310:i16, "MotFbError"=w1311:bool)  [unwired: 9 in]
                n759 = local write "Result(Number)"(w1310) -> ()
                n760 = local write "Result(Boolean) 1"(w1311) -> ()
                n761 = Enqueue Element(queue=w1313, element="START") -> ()  [unwired: 1 in, 4 out]
              }
              frame "PostionSetToZero" {
                n762 = call "FB_MFA_Set_Position1.vi"("Position Put"=sgl 0.0) -> ("Position Get"=w1316:sgl, "SetPositionError"=w1317:bool)  [unwired: 9 in]
                n763 = local write "Result(Boolean) 1"(w1317) -> ()
                n764 = local write "Result(DecimalPoint)"(w1316) -> ()
                n765 = Enqueue Element(queue=w1318, element="START") -> ()  [unwired: 1 in, 4 out]
              }
              frame "ReadZLatch0" {
                n766 = while {
                  i -> [w1324]
                  stop <- w1326 stop-if-true
                  n767 = call "FB_MFA_Read_Z_Latch1.vi"() -> ("EncoderZLatch"=w1328:bool)  [unwired: 11 in]
                  n768 = Equal?(x=w1328, y=FALSE) -> (x = y?=w1325:bool)
                  n769 = Not(x=w1328) -> (.not. x?=w1329:bool)
                  n770 = local write "Result(Boolean) 1"(w1329) -> ()
                  n771 = Equal?(x=w1324, y=3) -> (x = y?=w1322:bool)
                  n772 = Or(x=w1325, y=w1322) -> (x .or. y?=w1326:bool)
                  n773 = flat-sequence {
                    frame #0 {
                      n774 = Wait (ms)(milliseconds to wait=u32 300) -> ()  [unwired: 1 out]
                    }
                  }
                }
                n775 = Enqueue Element(queue=w1320, element="START") -> ()  [unwired: 1 in, 4 out]
              }
              frame "ReadZLatch1" {
                n776 = while {
                  i -> [w1335]
                  stop <- w1337 stop-if-true
                  n777 = call "FB_MFA_Read_Z_Latch1.vi"() -> ("EncoderZLatch"=w1339:bool)  [unwired: 11 in]
                  n778 = Equal?(x=w1339, y=TRUE) -> (x = y?=w1336:bool)
                  n779 = Not(x=w1339) -> (.not. x?=w1340:bool)
                  n780 = local write "Result(Boolean) 1"(w1340) -> ()
                  n781 = Equal?(x=w1335, y=3) -> (x = y?=w1333:bool)
                  n782 = Or(x=w1336, y=w1333) -> (x .or. y?=w1337:bool)
                  n783 = flat-sequence {
                    frame #0 {
                      n784 = Wait (ms)(milliseconds to wait=u32 300) -> ()  [unwired: 1 out]
                    }
                  }
                }
                n785 = Enqueue Element(queue=w1331, element="START") -> ()  [unwired: 1 in, 4 out]
              }
              frame "ReadPosPCBA" {
                n786 = call "FB_MFA_Read_Position_PCBA.vi"() -> ("Position Get"=w1342:sgl)  [unwired: 11 in]
                n787 = local write "Result(DecimalPoint)"(w1342) -> ()
                n788 = Enqueue Element(queue=w1343, element="START") -> ()  [unwired: 1 in, 4 out]
              }
              frame "ReadPosPCBA-Axis1" {
                n789 = call "FB_MFA_Read_Position_PCBA-Axis1.vi"() -> ("Position Get"=w1345:sgl)  [unwired: 11 in]
                n790 = local write "Result(DecimalPoint)"(w1345) -> ()
                n791 = Enqueue Element(queue=w1346, element="START") -> ()  [unwired: 1 in, 4 out]
              }
              frame "Hall" {
                n792 = call "FB_MFA_Read_Halls1.vi"() -> ("Hall Get"=w1350:i16)  [unwired: 11 in]
                n793 = local write "Result(Number)"(w1350) -> ()
                n794 = Enqueue Element(queue=w1348, element="START") -> ()  [unwired: 1 in, 4 out]
              }
              frame "ReadPosPCBA_SSI-Neg" {
                n795 = flat-sequence {
                  frame #0 {
                    n796 = local write "Position Get SSI-Neg*-1"(0.0) -> ()
                  }
                  frame #1 {
                    n797 = call "FB_MFA_Read_Position_PCBA.vi"() -> ("Position Get"=w1356:sgl)  [unwired: 11 in]
                    n798 = Multiply(x=w1356, y=sgl -1.0) -> (x*y=→"Position Get SSI-Neg*-1":sgl)
                    n799 = local write "Result(DecimalPoint)"(w1356) -> ()
                  }
                }
                n800 = Enqueue Element(queue=w1351, element="START") -> ()  [unwired: 1 in, 4 out]
              }
              frame "ReadPosPCBA_SSI-Pos" {
                n801 = flat-sequence {
                  frame #0 {
                    n802 = local write "Position Get SSI-Pos"(0.0) -> ()
                  }
                  frame #1 {
                    n803 = call "FB_MFA_Read_Position_PCBA.vi"() -> ("Position Get"=w1360:sgl)  [unwired: 11 in]
                    "Position Get SSI-Pos" <- w1360
                    n804 = local write "Result(DecimalPoint)"(w1360) -> ()
                  }
                }
                n805 = Enqueue Element(queue=w1357, element="START") -> ()  [unwired: 1 in, 4 out]
              }
              frame "CAL_LIMIT" {
                n806 = flat-sequence {
                  frame #0 {
                    w1369 = sgl 2.0 ("y")
                    n807 = local read "Position Get SSI-Pos"() -> (w1370:sgl)
                    n808 = Add(x=w1370, y=w1369) -> (x+y=w1367:sgl)
                    n809 = Subtract(x=w1370, y=w1369) -> (x-y=w1368:sgl)
                    n810 = Number To Fractional String(number=w1368, precision (6)=i16 3) -> (F-format string=→"SSI_LowLimit":string)  [unwired: 2 in]
                    n811 = Number To Fractional String(number=w1367, precision (6)=i16 3) -> (F-format string=→"SSI_HighLimit":string)  [unwired: 2 in]
                  }
                  frame #1 {
                  }
                }
                n812 = Enqueue Element(queue=w1361, element="START") -> ()  [unwired: 1 in, 4 out]
              }
            }
          }
          frame "TDS2002C" {
            w1373 = ";:" ("regular expression")
            n813 = local read "CMD"() -> (w1375:string)
            n814 = local read "TDS2002B"() -> (w1371:refnum<visa-resource-name>)
            n815 = Match Pattern(string=w1375, regular expression=w1373) -> (match substring=w1374:string)  [unwired: 1 in, 3 out]
            n816 = Equal?(x=w1374, y=w1373) -> (x = y?=w1372:bool)
            n817 = case shown="False" w1372 {
              tunnel: [w1380 TRUE] -> w1376
              tunnel: w1375 -> [w1379 w1423]
              tunnel: w1371 -> [w1378 w1424]
              frame False {
                n818 = while {
                  tunnel: [FALSE] -> w1380
                  tunnel: w1379 -> [w1382]
                  tunnel: w1378 -> [w1381]
                  i -> [w1386]
                  stop <- w1387 stop-if-true
                  w1400 = "," ("regular expression")
                  n819 = Match Pattern(string=w1382, regular expression=w1400) -> (before substring=w1399:string, after substring=w1401:string)  [unwired: 1 in, 2 out]
                  n820 = Match Pattern(string=w1401, regular expression=w1400) -> (before substring=w1398:string, after substring=w1395:string)  [unwired: 1 in, 2 out]
                  n821 = case shown="\"CH2\"" w1399 {
                    tunnel: [_ enum32{"CH 1", "CH 2", "CH 3", "CH 4"}."CH 1" ("CHANNEL") enum32{"CH 1", "CH 2", "CH 3", "CH 4"}."CH 2" ("CHANNEL")] -> w1402
                    frame "False", Default {
                    }
                    frame "CH1" {
                    }
                    frame "CH2" {
                    }
                  }
                  n822 = case shown="\"MEAS1\"" w1398 {
                    tunnel: [_ T7."MEAS1" ("MEASU") T7."MEAS2" ("MEASU") T7."MEAS3" ("MEASU") T7."MEAS4" ("MEASU") T7."MEAS5" ("MEASU")] -> w1397
                    frame "False", Default {
                    }
                    frame "MEAS1" {
                    }
                    frame "MEAS2" {
                    }
                    frame "MEAS3" {
                    }
                    frame "MEAS4" {
                    }
                    frame "MEAS5" {
                    }
                  }
                  n823 = case shown="\"PWIDTH\"" w1395 {
                    tunnel: [T6."NONE" ("MEAS TYPEs") T6."FREQUENCY" ("MEAS TYPEs") T6."MEAN" ("MEAS TYPEs") T6."PERIOD" ("MEAS TYPEs") T6."PK2PK" ("MEAS TYPEs") T6."MIN" ("MEAS TYPEs") T6."MAX" ("MEAS TYPEs") T6."RISE" ("MEAS TYPEs") T6."FALL" ("MEAS TYPEs") T6."CRMS" ("MEAS TYPEs") T6."PWIDTH" ("MEAS TYPEs") T6."NWIDTH" ("MEAS TYPEs")] -> w1396
                    frame "False", Default {
                    }
                    frame "FREQUENCY" {
                    }
                    frame "MEAN" {
                    }
                    frame "PERIOD" {
                    }
                    frame "PK2PK" {
                    }
                    frame "MIN" {
                    }
                    frame "MAX" {
                    }
                    frame "RISE" {
                    }
                    frame "FALL" {
                    }
                    frame "CRMS" {
                    }
                    frame "PWIDTH" {
                    }
                    frame "NWIDTH" {
                    }
                  }
                  n824 = local read "LowLimit"() -> (w1392:string)
                  n825 = call "MEASUREMENT FUNCTION.vi"("VISA resource name"=w1381, "CHANNEL"=w1402, "MEASU"=w1397, "MEAS TYPEs"=w1396) -> ("MEAS VALUE"=w1394:string)  [unwired: 6 in]
                  n826 = local read "HighLimit"() -> (w1391:string)
                  n827 = Fract/Exp String To Number(string=w1394) -> (number=w1393:dbl)  [unwired: 3 in, 1 out]
                  n828 = Fract/Exp String To Number(string=w1392) -> (number=w1389:dbl)  [unwired: 3 in, 1 out]
                  n829 = Fract/Exp String To Number(string=w1391) -> (number=w1390:dbl)  [unwired: 3 in, 1 out]
                  n830 = local write "Result(DecimalPoint)"(w1393) -> ()
                  n831 = Equal?(x=w1386, y=2) -> (x = y?=w1384:bool)
                  n832 = call "CompareMaxMin.vi"("Min"=w1389, "X"=w1393, "Max"=w1390) -> ("OutCompare"=w1388:bool)
                  n833 = Or(x=w1388, y=w1384) -> (x .or. y?=w1387:bool)
                }
              }
              frame True {
                # "CH1:COUP AC;:"
                n834 = call "GPIB_USB_WRITE+DEL READ_VISA IN_OUT(SubVI).vi"("VISA resource IN"=w1424, "GPIB/USB WRITE"=w1423, 4:FALSE) -> ()  [unwired: 3 in, 3 out]
              }
            }
            n835 = case shown="False" w1376 {
              tunnel: w1377 -> [w1426 w1428]
              frame False {
                n836 = Enqueue Element(queue=w1426, element="COMPARE") -> ()  [unwired: 1 in, 4 out]
              }
              frame True {
                n837 = Enqueue Element(queue=w1428, element="START") -> ()  [unwired: 1 in, 4 out]
              }
            }
          }
          frame "AAE908-207010ALF" {
            n838 = local read "CMD"() -> (w1432:string)
            n839 = case shown="\"RESET_ICT100\"" w1432 {
              frame "False", Default {
              }
              frame "RESET_ICT100" {
                n840 = flat-sequence {
                  tunnel: [w1435] -> w1433
                  tunnel: [w1437] -> w1434
                  tunnel: w1433 -> [w1437]
                  tunnel: w1434 -> [w1439]
                  frame #0 {
                    w1435 = refnum<k21> "RESET_ICT100" ("task/channels in")
                    # "low"
                    n841 = call-poly <vilib>:"DAQmx Write.vi"("task/channels in"=w1435, "data"=FALSE) -> ()  [unwired: 11 in, 3 out]
                  }
                  frame #1 {
                    n842 = Wait (ms)(milliseconds to wait=u32 200) -> ()  [unwired: 1 out]
                  }
                  frame #2 {
                    # "high"
                    n843 = call-poly <vilib>:"DAQmx Write.vi"("task/channels in"=w1439, "data"=TRUE) -> ()  [unwired: 11 in, 3 out]
                  }
                }
              }
              frame "RUNTEST" {
                n844 = flat-sequence {
                  tunnel: [w1443] -> w1442
                  tunnel: [w1445] -> w1441
                  tunnel: w1442 -> [w1445]
                  tunnel: w1441 -> [w1447]
                  frame #0 {
                    w1443 = refnum<k21> "RUNTEST" ("task/channels in")
                    # "LOW"
                    n845 = call-poly <vilib>:"DAQmx Write.vi"("task/channels in"=w1443, "data"=FALSE) -> ()  [unwired: 11 in, 3 out]
                  }
                  frame #1 {
                    n846 = Wait (ms)(milliseconds to wait=u32 200) -> ()  [unwired: 1 out]
                  }
                  frame #2 {
                    # "HIGH"
                    n847 = call-poly <vilib>:"DAQmx Write.vi"("task/channels in"=w1447, "data"=TRUE) -> ()  [unwired: 11 in, 3 out]
                  }
                }
              }
            }
            n848 = Enqueue Element(queue=w1430, element="START") -> ()  [unwired: 1 in, 4 out]
          }
          frame "NI-USB6501" {
            w1453 = "," ("regular expression")
            n849 = local read "CMD"() -> (w1456:string)
            n850 = Match Pattern(string=w1456, regular expression=w1453) -> (before substring=w1455:string, after substring=w1454:string)  [unwired: 1 in, 2 out]
            n851 = Match Pattern(string=w1454, regular expression=w1453) -> (before substring=w1452:string, after substring=w1451:string)  [unwired: 1 in, 2 out]
            n852 = case shown="\"S2\"" w1455 {
              tunnel: w1452 -> [_ w1459 w1463 _ _ _ _ _ _ _ _ _ _ _ _ _ _]
              tunnel: w1451 -> [_ w1458 w1462 _ _ _ _ _ _ _ _ _ _ _ _ _ _]
              frame "False", Default {
              }
              frame "S1" {
                n853 = call "S1&S2_CHECK.vi"("Message 2"=w1458, "MODE"=w1459, "task/channels in"=refnum<k21> "CHECK_STS_S1") -> ("S1Bit_out"=w1457:string)  [unwired: 8 in]
                n854 = local write "Result(string)"(w1457) -> ()
              }
              frame "S2" {
                # "S2,LOW,ปรับ S1 ทั้งหมดไปที่ตำแหน่งบน"
                n855 = call "S1&S2_CHECK.vi"("Message 2"=w1462, "MODE"=w1463, "task/channels in"=refnum<k21> "CHECK_STS_S2") -> ("S1Bit_out"=w1461:string)  [unwired: 8 in]
                n856 = local write "Result(string)"(w1461) -> ()
              }
              frame "S2_DEV1&J4_DEV2_0x55" {
                n857 = flat-sequence {
                  frame #0 {
                    # "B7"
                    # "B0"
                    n858 = call-poly <vilib>:"DAQmx Write.vi"("task/channels in"=refnum<k21> "Set0x55_P1", "data"=bool[] [FALSE, TRUE, FALSE, TRUE, FALSE, TRUE, FALSE, TRUE]) -> ()  [unwired: 11 in, 3 out]
                  }
                  frame #1 {
                    n859 = Wait (ms)(milliseconds to wait=u32 300) -> ()  [unwired: 1 out]
                  }
                  frame #2 {
                    n860 = call-poly <vilib>:"DAQmx Read.vi"("task/channels in"=refnum<k21> "CHECK_STS_IC4-J4") -> ("data"=w1469:bool[])  [unwired: 12 in, 2 out]
                    n861 = call "BooleanToBinary.vi"("data"=w1469) -> ("BinaryOut"=w1468:string)  [unwired: 10 in]
                    n862 = local write "Result(string)"(w1468) -> ()
                  }
                }
              }
              frame "S2_DEV1&J4_DEV2_0xAA" {
                n863 = flat-sequence {
                  frame #0 {
                    # "B7"
                    # "B0"
                    n864 = call-poly <vilib>:"DAQmx Write.vi"("task/channels in"=refnum<k21> "Set0x55_P1", "data"=bool[] [TRUE, FALSE, TRUE, FALSE, TRUE, FALSE, TRUE, FALSE]) -> ()  [unwired: 11 in, 3 out]
                  }
                  frame #1 {
                    n865 = Wait (ms)(milliseconds to wait=u32 300) -> ()  [unwired: 1 out]
                  }
                  frame #2 {
                    n866 = call-poly <vilib>:"DAQmx Read.vi"("task/channels in"=refnum<k21> "CHECK_STS_IC4-J4") -> ("data"=w1475:bool[])  [unwired: 12 in, 2 out]
                    n867 = call "BooleanToBinary.vi"("data"=w1475) -> ("BinaryOut"=w1474:string)  [unwired: 10 in]
                    n868 = local write "Result(string)"(w1474) -> ()
                  }
                }
              }
              frame "S1_DEV1&J4_DEV2_0x55" {
                n869 = flat-sequence {
                  frame #0 {
                    n870 = call-poly <vilib>:"DAQmx Write.vi"("task/channels in"=refnum<k21> "Set0x55_P0", "data"=bool[] [FALSE, TRUE, FALSE, TRUE, FALSE, TRUE, FALSE, TRUE]) -> ()  [unwired: 11 in, 3 out]
                  }
                  frame #1 {
                    n871 = Wait (ms)(milliseconds to wait=u32 300) -> ()  [unwired: 1 out]
                  }
                  frame #2 {
                    n872 = call-poly <vilib>:"DAQmx Read.vi"("task/channels in"=refnum<k21> "CHECK_STS_IC4-J4") -> ("data"=w1481:bool[])  [unwired: 12 in, 2 out]
                    n873 = call "BooleanToBinary.vi"("data"=w1481) -> ("BinaryOut"=w1480:string)  [unwired: 10 in]
                    n874 = local write "Result(string)"(w1480) -> ()
                  }
                }
              }
              frame "S1_DEV1&J4_DEV2_0xAA" {
                n875 = flat-sequence {
                  frame #0 {
                    n876 = call-poly <vilib>:"DAQmx Write.vi"("task/channels in"=refnum<k21> "Set0x55_P0", "data"=bool[] [TRUE, FALSE, TRUE, FALSE, TRUE, FALSE, TRUE, FALSE]) -> ()  [unwired: 11 in, 3 out]
                  }
                  frame #1 {
                    n877 = Wait (ms)(milliseconds to wait=u32 300) -> ()  [unwired: 1 out]
                  }
                  frame #2 {
                    n878 = call-poly <vilib>:"DAQmx Read.vi"("task/channels in"=refnum<k21> "CHECK_STS_IC4-J4") -> ("data"=w1487:bool[])  [unwired: 12 in, 2 out]
                    n879 = call "BooleanToBinary.vi"("data"=w1487) -> ("BinaryOut"=w1486:string)  [unwired: 10 in]
                    n880 = local write "Result(string)"(w1486) -> ()
                  }
                }
              }
              frame "OPTO-J4_DEV2" {
                n881 = while {
                  i -> [w1492]
                  stop <- w1490 stop-if-true
                  n882 = call-poly <vilib>:"DAQmx Read.vi"("task/channels in"=refnum<k21> "CHECK_STS_IC4-J4") -> ("data"=w1494:bool[])  [unwired: 12 in, 2 out]
                  n883 = call "BooleanToBinary.vi"("data"=w1494) -> ("BinaryOut"=w1493:string)  [unwired: 10 in]
                  n884 = Equal?(x=w1492, y=2) -> (x = y?=w1489:bool)
                  n885 = local write "Result(string)"(w1493) -> ()
                  n886 = flat-sequence {
                    tunnel: [w1497] -> w1490
                    tunnel: w1489 -> [w1497]
                    frame #0 {
                      n887 = Wait (ms)(milliseconds to wait=u32 350) -> ()  [unwired: 1 out]
                    }
                  }
                }
              }
              frame "DEV2_P1_J2_J7" {
                n888 = while {
                  i -> [w1501]
                  stop <- w1499 stop-if-true
                  n889 = call-poly <vilib>:"DAQmx Read.vi"("task/channels in"=refnum<k21> "DEV2_P1_J2_J7") -> ("data"=w1503:bool[])  [unwired: 12 in, 2 out]
                  n890 = call "BooleanToBinary.vi"("data"=w1503) -> ("BinaryOut"=w1502:string)  [unwired: 10 in]
                  n891 = Equal?(x=w1501, y=2) -> (x = y?=w1498:bool)
                  n892 = local write "Result(string)"(w1502) -> ()
                  n893 = flat-sequence {
                    tunnel: [w1506] -> w1499
                    tunnel: w1498 -> [w1506]
                    frame #0 {
                      n894 = Wait (ms)(milliseconds to wait=u32 250) -> ()  [unwired: 1 out]
                    }
                  }
                }
              }
              frame "ICT24_DEV2_P07" {
                n895 = while {
                  tunnel: refnum<k21> "ICT24_DEV2_P07" ("task/channels in") -> [w1513]
                  tunnel: [w1512] -> w1507
                  i -> [w1511]
                  stop <- w1509 stop-if-true
                  n896 = call-poly <vilib>:"DAQmx Read.vi"("task/channels in"=w1513) -> ("data"=w1512:bool)  [unwired: 12 in, 2 out]
                  n897 = Equal?(x=w1511, y=2) -> (x = y?=w1509:bool)
                }
                n898 = local write "Result(Boolean)"(w1507) -> ()
              }
              frame "ICT37_DEV2_P06" {
                n899 = while {
                  tunnel: refnum<k21> "ICT37_DEV2_P06" ("task/channels in") -> [w1520]
                  tunnel: [w1519] -> w1514
                  i -> [w1518]
                  stop <- w1516 stop-if-true
                  n900 = call-poly <vilib>:"DAQmx Read.vi"("task/channels in"=w1520) -> ("data"=w1519:bool)  [unwired: 12 in, 2 out]
                  n901 = Equal?(x=w1518, y=2) -> (x = y?=w1516:bool)
                }
                "Result(Boolean)" <- w1514
              }
              frame "ICT48_DEV2_P05" {
                n902 = while {
                  tunnel: refnum<k21> "ICT48_DEV2_P05" ("task/channels in") -> [w1527]
                  tunnel: [w1526] -> w1521
                  i -> [w1525]
                  stop <- w1523 stop-if-true
                  n903 = call-poly <vilib>:"DAQmx Read.vi"("task/channels in"=w1527) -> ("data"=w1526:bool)  [unwired: 12 in, 2 out]
                  n904 = Equal?(x=w1525, y=2) -> (x = y?=w1523:bool)
                }
                n905 = local write "Result(Boolean)"(w1521) -> ()
              }
              frame "ICT47_DEV2_P04" {
                n906 = while {
                  tunnel: refnum<k21> "ICT47_DEV2_P04" ("task/channels in") -> [w1534]
                  tunnel: [w1533] -> w1528
                  i -> [w1532]
                  stop <- w1530 stop-if-true
                  n907 = call-poly <vilib>:"DAQmx Read.vi"("task/channels in"=w1534) -> ("data"=w1533:bool)  [unwired: 12 in, 2 out]
                  n908 = Equal?(x=w1532, y=2) -> (x = y?=w1530:bool)
                }
                n909 = local write "Result(Boolean)"(w1528) -> ()
              }
              frame "ICT46_DEV2_P03" {
                n910 = while {
                  tunnel: refnum<k21> "ICT46_DEV2_P03" ("task/channels in") -> [w1541]
                  tunnel: [w1540] -> w1535
                  i -> [w1539]
                  stop <- w1537 stop-if-true
                  n911 = call-poly <vilib>:"DAQmx Read.vi"("task/channels in"=w1541) -> ("data"=w1540:bool)  [unwired: 12 in, 2 out]
                  n912 = Equal?(x=w1539, y=2) -> (x = y?=w1537:bool)
                }
                n913 = local write "Result(Boolean)"(w1535) -> ()
              }
              frame "ICT45_DEV2_P02" {
                n914 = while {
                  tunnel: refnum<k21> "ICT45_DEV2_P02" ("task/channels in") -> [w1548]
                  tunnel: [w1547] -> w1542
                  i -> [w1546]
                  stop <- w1544 stop-if-true
                  n915 = call-poly <vilib>:"DAQmx Read.vi"("task/channels in"=w1548) -> ("data"=w1547:bool)  [unwired: 12 in, 2 out]
                  n916 = Equal?(x=w1546, y=2) -> (x = y?=w1544:bool)
                }
                n917 = local write "Result(Boolean)"(w1542) -> ()
              }
              frame "ICT44_DEV2_P01" {
                n918 = while {
                  tunnel: refnum<k21> "ICT44_DEV2_P01" ("task/channels in") -> [w1555]
                  tunnel: [w1554] -> w1549
                  i -> [w1553]
                  stop <- w1551 stop-if-true
                  n919 = call-poly <vilib>:"DAQmx Read.vi"("task/channels in"=w1555) -> ("data"=w1554:bool)  [unwired: 12 in, 2 out]
                  n920 = Equal?(x=w1553, y=2) -> (x = y?=w1551:bool)
                }
                n921 = local write "Result(Boolean)"(w1549) -> ()
              }
              frame "ICT43_DEV2_P00" {
                n922 = while {
                  tunnel: refnum<k21> "ICT43_DEV2_P00" ("task/channels in") -> [w1562]
                  tunnel: [w1561] -> w1556
                  i -> [w1560]
                  stop <- w1558 stop-if-true
                  n923 = call-poly <vilib>:"DAQmx Read.vi"("task/channels in"=w1562) -> ("data"=w1561:bool)  [unwired: 12 in, 2 out]
                  n924 = Equal?(x=w1560, y=2) -> (x = y?=w1558:bool)
                }
                n925 = local write "Result(Boolean)"(w1556) -> ()
              }
            }
            n926 = Enqueue Element(queue=w1449, element="COMPARE") -> ()  [unwired: 1 in, 4 out]
          }
          frame "STM8" {
            n927 = flat-sequence {
              frame #0 {
                n928 = call "erasechip.vi"() -> ()  [unwired: 12 in]
              }
              frame #1 {
                n929 = Wait (ms)(milliseconds to wait=u32 0) -> ()  [unwired: 1 out]
              }
              frame #2 {
                n930 = local read "Serial Number"() -> (w1569:string)
                n931 = local read "Operator ID"() -> (w1570:string)
                n932 = call "Serial_numberExt.vi"("PCBA Barcode"=w1569, "Test Operator ID"=w1570) -> ("Check SUM HEX"=w1566:string, "Serial number (Hex)"=w1567:string, "ProgrammingResult"=w1568:bool)  [unwired: 7 in]
                n933 = local write "Serial number (Hex)"(w1567) -> ()
                n934 = local write "Check SUM HEX"(w1566) -> ()
                n935 = local write "Result(Boolean)"(w1568) -> ()
              }
            }
            n936 = Enqueue Element(queue=w1563, element="COMPARE") -> ()  [unwired: 1 in, 4 out]
          }
          frame "STM8_LNK215-429BLF" {
            n937 = flat-sequence {
              frame #0 {
                n938 = Wait (ms)(milliseconds to wait=u32 0) -> ()  [unwired: 1 out]
              }
              frame #1 {
                n939 = call "erasechip.vi"() -> ()  [unwired: 12 in]
              }
              frame #2 {
                n940 = Wait (ms)(milliseconds to wait=u32 0) -> ()  [unwired: 1 out]
              }
              frame #3 {
                # "Modify for 429B 26-08-2022"
                n941 = local read "Serial Number"() -> (w1578:string)
                n942 = local read "Operator ID"() -> (w1579:string)
                n943 = call "Serial_numberExt_429B.vi"("PCBA Barcode"=w1578, "Test Operator ID"=w1579) -> ("Check SUM HEX"=w1575:string, "Serial number (Hex)"=w1576:string, "ProgrammingResult"=w1577:bool)  [unwired: 7 in]
                n944 = local write "Result(Boolean)"(w1577) -> ()
                n945 = local write "Serial number (Hex)"(w1576) -> ()
                n946 = local write "Check SUM HEX"(w1575) -> ()
              }
              frame #4 {
                n947 = Wait (ms)(milliseconds to wait=u32 0) -> ()  [unwired: 1 out]
              }
            }
            n948 = Enqueue Element(queue=w1571, element="COMPARE") -> ()  [unwired: 1 in, 4 out]
          }
          frame "SNHEX" {
            n949 = local read "Serial number (Hex)"() -> (w1582:string)
            n950 = call "Hex to Str Hex.vi"("String"=w1582) -> ("hex integer string"=w1581:string)  [unwired: 10 in]
            n951 = local write "NOTE"(w1581) -> ()
            n952 = Enqueue Element(queue=w1583, element="COMPARE") -> ()  [unwired: 1 in, 4 out]
          }
          frame "SAMHEX" {
            n953 = local read "Check SUM HEX"() -> (w1585:string)
            n954 = local write "NOTE"(w1585) -> ()
            n955 = Enqueue Element(queue=w1586, element="COMPARE") -> ()  [unwired: 1 in, 4 out]
          }
          frame "APPLICATIONSW" {
            n956 = while {
              i -> [w1592]
              stop <- w1594 stop-if-true
              n957 = Equal?(x=w1592, y=15) -> (x = y?=w1593:bool)
              n958 = call "Programmingapplication.vi"() -> ("command line"=w1590:string, "Result"=w1595:bool)  [unwired: 10 in]
              n959 = Or(x=w1595, y=w1593) -> (x .or. y?=w1594:bool)
              n960 = local write "Result(Boolean)"(w1595) -> ()
              n961 = local write "App Firmware"(w1590) -> ()
            }
            n962 = Enqueue Element(queue=w1588, element="COMPARE") -> ()  [unwired: 1 in, 4 out]
          }
          frame "APPLICATIONSW_429B" {
            n963 = flat-sequence {
              frame #0 {
                n964 = Wait (ms)(milliseconds to wait=u32 0) -> ()  [unwired: 1 out]
              }
              frame #1 {
                n965 = while {
                  i -> [w1599]
                  stop <- w1600 stop-if-true
                  n966 = flat-sequence {
                    tunnel: [w1608] -> w1600
                    tunnel: w1599 -> [w1606]
                    frame #0 {
                      n967 = Delete(path (use dialog)=path "D:/Flasher Log/STM8.log") -> (error out=w1601:errorcluster)  [unwired: 4 in, 2 out]
                      n968 = call <vilib>:"Clear Errors.vi"("error in (no error)"=w1601) -> ()  [unwired: 5 in, 2 out]
                    }
                    frame #1 {
                      n969 = call "Programmingapplication_429B.vi"() -> ("command line"=w1603:string, "Result"=w1604:bool)  [unwired: 10 in]
                      n970 = Equal?(x=w1606, y=15) -> (x = y?=w1607:bool)
                      n971 = local write "App Firmware"(w1603) -> ()
                      n972 = Or(x=w1604, y=w1607) -> (x .or. y?=w1608:bool)
                      n973 = local write "Result(Boolean)"(w1604) -> ()
                    }
                    frame #2 {
                    }
                  }
                }
              }
              frame #2 {
                n974 = Wait (ms)(milliseconds to wait=u32 0) -> ()  [unwired: 1 out]
              }
            }
            n975 = Enqueue Element(queue=w1596, element="COMPARE") -> ()  [unwired: 1 in, 4 out]
          }
          frame "CHECK" {
            n976 = local read "App Firmware"() -> (w1612:string)
            n977 = local write "Result(string)"(w1612) -> ()
            n978 = Enqueue Element(queue=w1610, element="COMPARE") -> ()  [unwired: 1 in, 4 out]
          }
          frame "AAE908-207010ALF_RS485" {
            n979 = while {
              i -> [w1615]
              stop <- w1616 stop-if-true
              n980 = flat-sequence {
                tunnel: [w1625] -> w1616
                tunnel: w1615 -> [w1624]
                frame #0 {
                  n981 = local write "Result(Number)"(i8 0) -> ()
                }
                frame #1 {
                  n982 = local read "MUX RELAY"() -> (w1626:refnum<visa-resource-name>)
                  n983 = local read "CMD"() -> (w1628:string)
                  n984 = call "Untitled 2.vi"("RelayCMD"=w1628, "RelayCtrl"=w1626, "RS485 RECEIVER"="RS485 RECEIVER") -> ("RECEIVED DATA"=w1620:string)  [unwired: 8 in]
                  n985 = String Length(string=w1620) -> (length=w1618:i32)
                  n986 = Greater?(x=w1618, y=7) -> (0:w1621:bool)
                  n987 = local write "Result(Number)"(w1618) -> ()
                  n988 = Equal?(x=w1624, y=3) -> (x = y?=w1622:bool)
                  n989 = Or(x=w1621, y=w1622) -> (x .or. y?=w1625:bool)
                }
              }
            }
            n990 = Enqueue Element(queue=w1613, element="COMPARE") -> ()  [unwired: 1 in, 4 out]
          }
          frame "E3631A" {
            w1639 = "MEAS" ("regular expression")
            n991 = local read "CMD"() -> (w1637:string)
            n992 = Match Pattern(string=w1637, regular expression=w1639) -> (match substring=w1640:string)  [unwired: 4 out]
            n993 = Equal?(x=w1640, y=w1639) -> (x = y?=w1638:bool)
            n994 = case shown="False" w1638 {
              tunnel: [FALSE ("write") TRUE ("write")] -> w1631
              frame False {
              }
              frame True {
              }
            }
            n995 = local read "E3631A"() -> (w1633:refnum<visa-resource-name>)
            n996 = case shown="False" FALSE {
              tunnel: w1637 -> [w1645 w1651]
              tunnel: [w1642 w1649] -> w1635
              tunnel: w1633 -> [w1646 w1648]
              tunnel: [w1641 w1647] -> w1632
              tunnel: w1631 -> [w1641 w1647]
              frame False {
                n997 = call "VISA WRITE&READ.vi"("byte count"=u32 50, "Delay(mS)"=u32 50, "Read?"=w1641, "write buffer"=w1645, "VISA resource name In"=w1646) -> ("read buffer"=w1642:string)  [unwired: 4 in, 2 out]
              }
              frame True {
                w1654 = u16 10 items=["1.0"=10, "1.5"=15, "2.0"=20] ("stop bits")
                w1655 = u16 0 items=["None", "Odd", "Even", "Mark", "Space"] ("parity")
                n998 = Concatenate Strings(w1651, "\r\n") -> (w1650:string)
                n999 = call "Basic Serial Write and Read.vi"("VISA resource name"=w1648, "baud rate"=u32 9600, "data bits"=u16 8, "parity"=w1655, "stop bits"=w1654, "write"=TRUE, "read"=w1647, "string to write"=w1650) -> ("read string"=w1649:string)  [unwired: 1 in, 1 out]
              }
            }
            n1000 = call <vilib>:"Trim Whitespace.vi"("string"=w1635) -> ("trimmed string"=w1630:string)  [unwired: 1 in]
            "Result" <- w1630
            n1001 = Fract/Exp String To Number(string=w1630) -> (number=→"Result(DecimalPoint)":dbl)  [unwired: 3 in, 1 out]
            n1002 = case shown="True" w1632 {
              tunnel: w1636 -> [w1658 w1660]
              frame False {
                n1003 = Enqueue Element(queue=w1658, element="START") -> ()  [unwired: 1 in, 4 out]
              }
              frame True {
                n1004 = Enqueue Element(queue=w1660, element="COMPARE") -> ()  [unwired: 1 in, 4 out]
              }
            }
          }
          frame "E3634A#1" {
            w1674 = "MEAS" ("regular expression")
            n1005 = local read "CMD"() -> (w1672:string)
            n1006 = Match Pattern(string=w1672, regular expression=w1674) -> (match substring=w1675:string)  [unwired: 4 out]
            n1007 = Equal?(x=w1675, y=w1674) -> (x = y?=w1673:bool)
            n1008 = case shown="False" w1673 {
              tunnel: [FALSE ("write") TRUE ("write")] -> w1666
              frame False {
              }
              frame True {
              }
            }
            n1009 = local read "E3643A#1"() -> (w1668:refnum<visa-resource-name>)
            n1010 = case shown="True" FALSE {
              tunnel: w1672 -> [w1680 w1686]
              tunnel: [w1677 w1684] -> w1670
              tunnel: w1668 -> [w1681 w1683]
              tunnel: [w1676 w1682] -> w1667
              tunnel: w1666 -> [w1676 w1682]
              frame False {
                n1011 = call "VISA WRITE&READ.vi"("byte count"=u32 50, "Delay(mS)"=u32 100, "Read?"=w1676, "write buffer"=w1680, "VISA resource name In"=w1681) -> ("read buffer"=w1677:string)  [unwired: 4 in, 2 out]
              }
              frame True {
                w1689 = u16 10 items=["1.0"=10, "1.5"=15, "2.0"=20] ("stop bits")
                w1690 = u16 0 items=["None", "Odd", "Even", "Mark", "Space"] ("parity")
                n1012 = Concatenate Strings(w1686, "\r\n") -> (w1685:string)
                n1013 = call "Basic Serial Write and Read.vi"("VISA resource name"=w1683, "baud rate"=u32 9600, "data bits"=u16 8, "parity"=w1690, "stop bits"=w1689, "write"=TRUE, "read"=w1682, "string to write"=w1685) -> ("read string"=w1684:string)  [unwired: 1 in, 1 out]
              }
            }
            n1014 = call <vilib>:"Trim Whitespace.vi"("string"=w1670) -> ("trimmed string"=w1664:string)  [unwired: 1 in]
            n1015 = Fract/Exp String To Number(string=w1664) -> (number=w1665:dbl)  [unwired: 3 in, 1 out]
            n1016 = local write "Result(DecimalPoint)"(w1665) -> ()
            n1017 = case shown="True" w1667 {
              tunnel: w1671 -> [w1693 w1695]
              frame False {
                n1018 = Enqueue Element(queue=w1693, element="START") -> ()  [unwired: 1 in, 4 out]
              }
              frame True {
                n1019 = Enqueue Element(queue=w1695, element="COMPARE") -> ()  [unwired: 1 in, 4 out]
              }
            }
          }
          frame "E3643A" {
            w1709 = "MEAS" ("regular expression")
            n1020 = local read "CMD"() -> (w1707:string)
            n1021 = Match Pattern(string=w1707, regular expression=w1709) -> (match substring=w1710:string)  [unwired: 4 out]
            n1022 = Equal?(x=w1710, y=w1709) -> (x = y?=w1708:bool)
            n1023 = case shown="False" w1708 {
              tunnel: [FALSE ("write") TRUE ("write")] -> w1701
              frame False {
              }
              frame True {
              }
            }
            n1024 = local read "E3643A"() -> (w1703:refnum<visa-resource-name>)
            n1025 = case shown="True" TRUE {
              tunnel: w1707 -> [w1715 w1721]
              tunnel: [w1712 w1719] -> w1705
              tunnel: w1703 -> [w1716 w1718]
              tunnel: [w1711 w1717] -> w1702
              tunnel: w1701 -> [w1711 w1717]
              frame False {
                n1026 = call "VISA WRITE&READ.vi"("byte count"=u32 50, "Delay(mS)"=u32 100, "Read?"=w1711, "write buffer"=w1715, "VISA resource name In"=w1716) -> ("read buffer"=w1712:string)  [unwired: 4 in, 2 out]
              }
              frame True {
                w1724 = u16 10 items=["1.0"=10, "1.5"=15, "2.0"=20] ("stop bits")
                w1725 = u16 0 items=["None", "Odd", "Even", "Mark", "Space"] ("parity")
                n1027 = Concatenate Strings(w1721, "\r\n") -> (w1720:string)
                n1028 = call "Basic Serial Write and Read.vi"("VISA resource name"=w1718, "baud rate"=u32 9600, "data bits"=u16 8, "parity"=w1725, "stop bits"=w1724, "write"=TRUE, "read"=w1717, "string to write"=w1720) -> ("read string"=w1719:string)  [unwired: 1 in, 1 out]
              }
            }
            n1029 = call <vilib>:"Trim Whitespace.vi"("string"=w1705) -> ("trimmed string"=w1699:string)  [unwired: 1 in]
            n1030 = Fract/Exp String To Number(string=w1699) -> (number=w1700:dbl)  [unwired: 3 in, 1 out]
            n1031 = local write "Result(DecimalPoint)"(w1700) -> ()
            n1032 = case shown="True" w1702 {
              tunnel: w1706 -> [w1728 w1730]
              frame False {
                n1033 = Enqueue Element(queue=w1728, element="START") -> ()  [unwired: 1 in, 4 out]
              }
              frame True {
                n1034 = Enqueue Element(queue=w1730, element="COMPARE") -> ()  [unwired: 1 in, 4 out]
              }
            }
          }
          frame "E3634A#2" {
            w1744 = "MEAS" ("regular expression")
            n1035 = local read "CMD"() -> (w1742:string)
            n1036 = Match Pattern(string=w1742, regular expression=w1744) -> (match substring=w1745:string)  [unwired: 4 out]
            n1037 = Equal?(x=w1745, y=w1744) -> (x = y?=w1743:bool)
            n1038 = case shown="True" w1743 {
              tunnel: [FALSE ("write") TRUE ("write")] -> w1736
              frame False {
              }
              frame True {
              }
            }
            n1039 = local read "E3643A#2"() -> (w1738:refnum<visa-resource-name>)
            n1040 = case shown="False" FALSE {
              tunnel: w1742 -> [w1750 w1756]
              tunnel: [w1747 w1754] -> w1740
              tunnel: w1738 -> [w1751 w1753]
              tunnel: [w1746 w1752] -> w1737
              tunnel: w1736 -> [w1746 w1752]
              frame False {
                n1041 = call "VISA WRITE&READ.vi"("byte count"=u32 50, "Delay(mS)"=u32 50, "Read?"=w1746, "write buffer"=w1750, "VISA resource name In"=w1751) -> ("read buffer"=w1747:string)  [unwired: 4 in, 2 out]
              }
              frame True {
                w1759 = u16 10 items=["1.0"=10, "1.5"=15, "2.0"=20] ("stop bits")
                w1760 = u16 0 items=["None", "Odd", "Even", "Mark", "Space"] ("parity")
                n1042 = Concatenate Strings(w1756, "\r\n") -> (w1755:string)
                n1043 = call "Basic Serial Write and Read.vi"("VISA resource name"=w1753, "baud rate"=u32 9600, "data bits"=u16 8, "parity"=w1760, "stop bits"=w1759, "write"=TRUE, "read"=w1752, "string to write"=w1755) -> ("read string"=w1754:string)  [unwired: 1 in, 1 out]
              }
            }
            n1044 = call <vilib>:"Trim Whitespace.vi"("string"=w1740) -> ("trimmed string"=w1734:string)  [unwired: 1 in]
            n1045 = Fract/Exp String To Number(string=w1734) -> (number=w1735:dbl)  [unwired: 3 in, 1 out]
            n1046 = local write "Result(DecimalPoint)"(w1735) -> ()
            n1047 = case shown="True" w1737 {
              tunnel: w1741 -> [w1763 w1765]
              frame False {
                n1048 = Enqueue Element(queue=w1763, element="START") -> ()  [unwired: 1 in, 4 out]
              }
              frame True {
                n1049 = Enqueue Element(queue=w1765, element="COMPARE") -> ()  [unwired: 1 in, 4 out]
              }
            }
          }
          frame "E3634A#3" {
            w1779 = "MEAS" ("regular expression")
            n1050 = local read "CMD"() -> (w1777:string)
            n1051 = Match Pattern(string=w1777, regular expression=w1779) -> (match substring=w1780:string)  [unwired: 4 out]
            n1052 = Equal?(x=w1780, y=w1779) -> (x = y?=w1778:bool)
            n1053 = case shown="True" w1778 {
              tunnel: [FALSE ("write") TRUE ("write")] -> w1771
              frame False {
              }
              frame True {
              }
            }
            n1054 = local read "E3643A#3"() -> (w1773:refnum<visa-resource-name>)
            n1055 = case shown="False" FALSE {
              tunnel: w1777 -> [w1785 w1791]
              tunnel: [w1782 w1789] -> w1775
              tunnel: w1773 -> [w1786 w1788]
              tunnel: [w1781 w1787] -> w1772
              tunnel: w1771 -> [w1781 w1787]
              frame False {
                n1056 = call "VISA WRITE&READ.vi"("byte count"=u32 50, "Delay(mS)"=u32 50, "Read?"=w1781, "write buffer"=w1785, "VISA resource name In"=w1786) -> ("read buffer"=w1782:string)  [unwired: 4 in, 2 out]
              }
              frame True {
                w1794 = u16 10 items=["1.0"=10, "1.5"=15, "2.0"=20] ("stop bits")
                w1795 = u16 0 items=["None", "Odd", "Even", "Mark", "Space"] ("parity")
                n1057 = Concatenate Strings(w1791, "\r\n") -> (w1790:string)
                n1058 = call "Basic Serial Write and Read.vi"("VISA resource name"=w1788, "baud rate"=u32 9600, "data bits"=u16 8, "parity"=w1795, "stop bits"=w1794, "write"=TRUE, "read"=w1787, "string to write"=w1790) -> ("read string"=w1789:string)  [unwired: 1 in, 1 out]
              }
            }
            n1059 = call <vilib>:"Trim Whitespace.vi"("string"=w1775) -> ("trimmed string"=w1769:string)  [unwired: 1 in]
            n1060 = Fract/Exp String To Number(string=w1769) -> (number=w1770:dbl)  [unwired: 3 in, 1 out]
            n1061 = local write "Result(DecimalPoint)"(w1770) -> ()
            n1062 = case shown="True" w1772 {
              tunnel: w1776 -> [w1798 w1800]
              frame False {
                n1063 = Enqueue Element(queue=w1798, element="START") -> ()  [unwired: 1 in, 4 out]
              }
              frame True {
                n1064 = Enqueue Element(queue=w1800, element="COMPARE") -> ()  [unwired: 1 in, 4 out]
              }
            }
          }
          frame "34450A" {
            w1813 = ":DC:RES"
            w1815 = ":AC:RES"
            w1816 = "CONF"
            n1065 = local read "34450A"() -> (w1804:refnum<visa-resource-name>)
            n1066 = local read "CMD"() -> (w1805:string)
            n1067 = Match Pattern(string=w1805, regular expression=w1816) -> (match substring=w1821:string)  [unwired: 4 out]
            n1068 = Match Pattern(string=w1805, regular expression=w1815) -> (match substring=w1817:string)  [unwired: 4 out]
            n1069 = Match Pattern(string=w1805, regular expression=w1813) -> (match substring=w1812:string)  [unwired: 4 out]
            n1070 = Equal?(x=w1821, y=w1816) -> (x = y?=w1810:bool)
            n1071 = Equal?(x=w1817, y=w1815) -> (x = y?=w1811:bool)
            n1072 = Equal?(x=w1812, y=w1813) -> (x = y?=w1809:bool)
            n1073 = Compound Arithmetic op=OR(w1810, w1811, w1809) -> (w1806:bool)
            n1074 = case shown="True" w1806 {
              tunnel: [u32 500 ("Delay(mS)") u32 0 ("Delay(mS)")] -> w1820
              frame False {
              }
              frame True {
              }
            }
            n1075 = Not(x=w1806) -> (.not. x?=w1818:bool)
            n1076 = call "VISA WRITE&READ.vi"("byte count"=u32 50, "Delay(mS)"=w1820, "Read?"=w1818, "write buffer"=w1805, "VISA resource name In"=w1804) -> ("read buffer"=w1814:string)  [unwired: 1 in, 5 out]
            n1077 = call <vilib>:"Trim Whitespace.vi"("string"=w1814) -> ("trimmed string"=w1808:string)  [unwired: 1 in]
            n1078 = local write "Result"(w1808) -> ()
            n1079 = case shown="False" w1806 {
              tunnel: w1807 -> [w1822 w1824]
              frame False {
                n1080 = Enqueue Element(queue=w1822, element="COMPARE") -> ()  [unwired: 1 in, 4 out]
              }
              frame True {
                n1081 = Enqueue Element(queue=w1824, element="START") -> ()  [unwired: 1 in, 4 out]
              }
            }
          }
          frame "33210A" {
            n1082 = local read "33210A"() -> (w1829:refnum<visa-resource-name>)
            n1083 = local read "CMD"() -> (w1831:string)
            n1084 = call "VISA WRITE&READ.vi"("Read?"=FALSE, "write buffer"=w1831, "VISA resource name In"=w1829) -> ()  [unwired: 3 in, 6 out]
            n1085 = case shown="True" TRUE {
              tunnel: w1832 -> [w1833 w1835]
              frame False {
                n1086 = Enqueue Element(queue=w1833, element="COMPARE") -> ()  [unwired: 1 in, 4 out]
              }
              frame True {
                n1087 = Enqueue Element(queue=w1835, element="START") -> ()  [unwired: 1 in, 4 out]
              }
            }
          }
          frame "34461A" {
            w1844 = "CONF"
            n1088 = local read "34461A"() -> (w1841:refnum<visa-resource-name>)
            n1089 = local read "CMD"() -> (w1842:string)
            n1090 = Match Pattern(string=w1842, regular expression=w1844) -> (match substring=w1848:string)  [unwired: 4 out]
            n1091 = Equal?(x=w1848, y=w1844) -> (x = y?=w1840:bool)
            n1092 = case shown="False" w1840 {
              tunnel: [u32 30 ("Delay(mS)") u32 0 ("Delay(mS)")] -> w1847
              frame False {
              }
              frame True {
              }
            }
            n1093 = Not(x=w1840) -> (.not. x?=w1845:bool)
            n1094 = call "VISA WRITE&READ.vi"("byte count"=u32 50, "Delay(mS)"=w1847, "Read?"=w1845, "write buffer"=w1842, "VISA resource name In"=w1841) -> ("read buffer"=w1837:string)  [unwired: 1 in, 5 out]
            n1095 = call <vilib>:"Trim Whitespace.vi"("string"=w1837) -> ("trimmed string"=w1838:string)  [unwired: 1 in]
            n1096 = Fract/Exp String To Number(string=w1838) -> (number=w1839:dbl)  [unwired: 3 in, 1 out]
            n1097 = local write "Result(DecimalPoint)"(w1839) -> ()
            n1098 = case shown="False" w1840 {
              tunnel: w1843 -> [w1849 w1851]
              frame False {
                n1099 = Enqueue Element(queue=w1849, element="COMPARE") -> ()  [unwired: 1 in, 4 out]
              }
              frame True {
                n1100 = Enqueue Element(queue=w1851, element="START") -> ()  [unwired: 1 in, 4 out]
              }
            }
          }
          frame "34410A" {
            n1101 = local read "TESTING HEAD#"() -> (w1857:string)
            n1102 = flat-sequence {
              tunnel: w1857 -> [w1859]
              tunnel: [w1864] -> w1855
              tunnel: [w1892] -> w1856
              tunnel: w1855 -> [w1892]
              frame #0 {
                n1103 = case shown="\"HEAD2\"" w1859 {
                  frame "False", Default {
                  }
                  frame "HEAD2" {
                    n1104 = local read "Description"() -> (w1860:string)
                    n1105 = case shown="\"Meas RES at J3 & TP4\"" w1860 {
                      frame "False", Default {
                      }
                      frame "Meas RES at J3 & TP4" {
                        n1106 = local read "MUX RELAY"() -> (w1862:refnum<visa-resource-name>)
                        n1107 = call "ControlRelay_ver10.vi"("VISA session"=w1862, "write buffer"="@b007t", "Relay Setting"=T4."Manual Cmd") -> ()  [unwired: 10 in, 7 out]
                      }
                    }
                  }
                }
              }
              frame #1 {
                n1108 = local read "34410A"() -> (w1865:refnum<visa-resource-name>)
                n1109 = while {
                  tunnel: w1865 -> [w1879]
                  tunnel: [w1872] -> w1864
                  i -> [w1867]
                  stop <- w1869 stop-if-true
                  w1877 = "CONF"
                  n1110 = local read "CMD"() -> (w1878:string)
                  n1111 = Match Pattern(string=w1878, regular expression=w1877) -> (match substring=w1873:string)  [unwired: 4 out]
                  n1112 = Equal?(x=w1873, y=w1877) -> (x = y?=w1872:bool)
                  n1113 = case shown="True" w1872 {
                    tunnel: [u32 30 ("Delay(mS)") u32 0 ("Delay(mS)")] -> w1874
                    frame False {
                    }
                    frame True {
                    }
                  }
                  n1114 = Not(x=w1872) -> (.not. x?=w1876:bool)
                  n1115 = call "VISA WRITE&READ.vi"("byte count"=u32 50, "Delay(mS)"=w1874, "Read?"=w1876, "write buffer"=w1878, "VISA resource name In"=w1879) -> ("read buffer"=w1881:string)  [unwired: 1 in, 5 out]
                  n1116 = local read "Description"() -> (w1871:string)
                  n1117 = call <vilib>:"Trim Whitespace.vi"("string"=w1881) -> ("trimmed string"=w1880:string)  [unwired: 1 in]
                  n1118 = Fract/Exp String To Number(string=w1880) -> (number=w1882:dbl)  [unwired: 3 in, 1 out]
                  n1119 = case shown="\"Meas supply current consumption\"" w1871 {
                    tunnel: w1882 -> [w1884 w1888]
                    tunnel: [TRUE ("OutCompare") w1885] -> w1870
                    frame "False", Default {
                      n1120 = local write "Result(DecimalPoint)"(w1884) -> ()
                    }
                    frame "Meas supply current consumption" {
                      n1121 = local write "Result(DecimalPoint)"(w1888) -> ()
                      n1122 = call "CompareMaxMin.vi"("Min"=0.007, "X"=w1888, "Max"=0.0073) -> ("OutCompare"=w1885:bool)
                    }
                  }
                  n1123 = Equal?(x=w1867, y=100) -> (x = y?=w1868:bool)
                  n1124 = Or(x=w1870, y=w1868) -> (x .or. y?=w1869:bool)
                }
              }
              frame #2 {
                n1125 = local read "TESTING HEAD#"() -> (w1891:string)
                n1126 = case shown="\"HEAD2\"" w1891 {
                  frame "False", Default {
                  }
                  frame "HEAD2" {
                    n1127 = local read "Description"() -> (w1893:string)
                    n1128 = case shown="\"Meas RES at J3 & TP4\"" w1893 {
                      frame "False", Default {
                      }
                      frame "Meas RES at J3 & TP4" {
                        n1129 = local read "MUX RELAY"() -> (w1895:refnum<visa-resource-name>)
                        n1130 = call "ControlRelay_ver10.vi"("VISA session"=w1895, "write buffer"="@b007f", "Relay Setting"=T4."Manual Cmd") -> ()  [unwired: 10 in, 7 out]
                      }
                    }
                  }
                }
              }
            }
            n1131 = case shown="False" w1856 {
              tunnel: w1858 -> [w1897 w1899]
              frame False {
                n1132 = Enqueue Element(queue=w1897, element="COMPARE") -> ()  [unwired: 1 in, 4 out]
              }
              frame True {
                n1133 = Enqueue Element(queue=w1899, element="START") -> ()  [unwired: 1 in, 4 out]
              }
            }
          }
          frame "DSO1072B" {
            n1134 = local read "CMD"() -> (w1901:string)
            n1135 = while {
              tunnel: [w1915] -> w1902
              tunnel: w1901 -> [w1908]
              i -> [w1920]
              stop <- w1910 stop-if-true
              w1928 = ":MEAS"
              # "20"
              n1136 = local read "DSO1052B"() -> (w1927:refnum<visa-resource-name>)
              n1137 = local read "Description"() -> (w1925:string)
              n1138 = Match Pattern(string=w1908, regular expression=w1928) -> (match substring=w1932:string)  [unwired: 4 out]
              n1139 = Match Pattern(string=w1908, regular expression=":MEAS:") -> (after substring=w1913:string)  [unwired: 4 out]
              n1140 = Not Equal?(x=w1932, y=w1928) -> (x != y?=w1915:bool)
              n1141 = Equal?(x=w1925, y="Meas voltage that will deop either 0 to 0.3 or 5.4 to 5.8V") -> (x = y?=w1923:bool)
              n1142 = case shown="False" w1915 {
                tunnel: [u32 500 ("Delay(mS)") u32 0 ("Delay(mS)")] -> w1931
                frame False {
                }
                frame True {
                }
              }
              n1143 = Not(x=w1915) -> (.not. x?=w1929:bool)
              n1144 = call "VISA WRITE&READ.vi"("byte count"=u32 50, "Delay(mS)"=w1931, "Read?"=w1929, "write buffer"=w1908, "VISA resource name In"=w1927) -> ("read buffer"=w1926:string)  [unwired: 1 in, 5 out]
              n1145 = call <vilib>:"Trim Whitespace.vi"("string"=w1926) -> ("trimmed string"=w1912:string)  [unwired: 1 in]
              "trimmed string" <- w1912
              n1146 = Fract/Exp String To Number(string=w1912) -> (number=w1911:dbl)  [unwired: 3 in, 1 out]
              "number" <- w1911
              n1147 = case shown="\"FREQ? CHAN1\", \"FREQ? CHAN2\"" w1913 {
                tunnel: [w1971 w1974 w1980 w1984] -> w1905
                tunnel: w1911 -> [w1971 w1973 w1979 w1983]
                frame "False", Default {
                }
                frame "NDUT? CHAN1", "NDUT? CHAN2", "PDUT? CHAN1", "PDUT? CHAN2" {
                  n1148 = Multiply(x=w1973, y=100.0) -> (x*y=w1974:dbl)
                }
                frame "FREQ? CHAN1", "FREQ? CHAN2" {
                  n1149 = local read "Description"() -> (w1978:string)
                  n1150 = Equal?(x=w1978, y="Meas OSC calibrated frequenc at TP15 wrt TP4") -> (x = y?=w1976:bool)
                  n1151 = case shown="False" w1976 {
                    tunnel: [1000.0 ("y") 1.0 ("y")] -> w1975
                    frame False {
                    }
                    frame True {
                    }
                  }
                  n1152 = Multiply(x=w1979, y=w1975) -> (x*y=w1980:dbl)
                }
                frame "PWID? CHAN2" {
                  n1153 = call "CompareMaxMin.vi"("Min"=0.098, "X"=w1983, "Max"=0.012) -> ("OutCompare"=w1985:bool)
                  n1154 = case shown="True" w1985 {
                    tunnel: [w1989 w1991] -> w1984
                    tunnel: w1983 -> [w1990 w1991]
                    frame False {
                      n1155 = Subtract(x=w1990, y=0.0005) -> (x-y=w1989:dbl)
                    }
                    frame True {
                    }
                  }
                }
              }
              n1156 = case shown="True" w1923 {
                tunnel: w1911 -> [_ w2013]
                tunnel: [w1993 w1999] -> w1922
                tunnel: [w1992 w1997] -> w1921
                frame False {
                  n1157 = local read "HighLimit"() -> (w1994:string)
                  n1158 = local read "LowLimit"() -> (w1995:string)
                  n1159 = Fract/Exp String To Number(string=w1994) -> (number=w1993:dbl)  [unwired: 3 in, 1 out]
                  n1160 = Fract/Exp String To Number(string=w1995) -> (number=w1992:dbl)  [unwired: 3 in, 1 out]
                }
                frame True {
                  # "5.4"
                  # "5.8"
                  n1161 = local read "HighLimit"() -> (w2005:string)
                  n1162 = local read "LowLimit"() -> (w2004:string)
                  n1163 = Match Pattern(string=w2005, regular expression=" or 5.8") -> (before substring=w2001:string)  [unwired: 1 in, 3 out]
                  n1164 = Match Pattern(string=w2005, regular expression="0.3 or ") -> (after substring=w2009:string)  [unwired: 1 in, 3 out]
                  n1165 = Match Pattern(string=w2004, regular expression=" or 5.4") -> (before substring=w2000:string)  [unwired: 1 in, 3 out]
                  n1166 = Match Pattern(string=w2004, regular expression="0.0 or ") -> (after substring=w2008:string)  [unwired: 1 in, 3 out]
                  n1167 = Fract/Exp String To Number(string=w2009) -> (number=w1998:dbl)  [unwired: 3 in, 1 out]
                  n1168 = Fract/Exp String To Number(string=w2008) -> (number=w1996:dbl)  [unwired: 3 in, 1 out]
                  n1169 = call "CompareMaxMin.vi"("Min"=w1996, "X"=w2013, "Max"=w1998) -> ("OutCompare"=w2010:bool)
                  n1170 = case shown="True" w2010 {
                    tunnel: w2009 -> [_ w2021]
                    tunnel: w2008 -> [_ w2020]
                    tunnel: [w2017 w2021] -> w2007
                    tunnel: [w2015 w2020] -> w2006
                    tunnel: w2001 -> [w2017 _]
                    tunnel: w2000 -> [w2015 _]
                    tunnel: [w2016 w2019] -> w1999
                    tunnel: w1998 -> [_ w2019]
                    tunnel: [w2014 w2018] -> w1997
                    tunnel: w1996 -> [_ w2018]
                    frame False {
                      n1171 = Fract/Exp String To Number(string=w2017) -> (number=w2016:dbl)  [unwired: 3 in, 1 out]
                      n1172 = Fract/Exp String To Number(string=w2015) -> (number=w2014:dbl)  [unwired: 3 in, 1 out]
                    }
                    frame True {
                    }
                  }
                  n1173 = local write "HighLimit"(w2007) -> ()
                  n1174 = local write "LowLimit"(w2006) -> ()
                }
              }
              n1175 = local read "Description"() -> (w1907:string)
              n1176 = Absolute Value(x=w1905) -> (abs(x)=w1904:dbl)
              n1177 = case shown="\"False\", Default" w1907 {
                tunnel: w1922 -> [w1941 _ _ _ _ _ _ _ _]
                tunnel: w1921 -> [w1940 _ _ _ _ _ _ _ _]
                tunnel: [w1939 TRUE ("OutCompare") TRUE ("OutCompare") w1947 w1951 w1955 w1959 w1963 w1967] -> w1916
                tunnel: w1904 -> [w1938 _ _ w1946 w1950 w1954 w1958 w1962 w1966]
                frame "False", Default {
                  n1178 = call "CompareMaxMin.vi"("Min"=w1940, "X"=w1938, "Max"=w1941) -> ("OutCompare"=w1939:bool)
                }
                frame "WAVE FORM IS NULL?" {
                }
                frame "CHECK WF IS NULL?" {
                }
                frame "Meas OSC calibrated frequenc at TP15 wrt TP4" {
                  (unwired) 0.0 ("Min")
                  (unwired) 2000.0 ("Max")
                  n1179 = call "CompareMaxMin.vi"("Min"=997.0, "X"=w1946, "Max"=1003.0) -> ("OutCompare"=w1947:bool)
                }
                frame "Meas O/P freq. at TP14 wrt TP4" {
                  (unwired) 74700.0 ("Min")
                  (unwired) 91300.0 ("Max")
                  n1180 = call "CompareMaxMin.vi"("Min"=82998.0, "X"=w1950, "Max"=83002.0) -> ("OutCompare"=w1951:bool)
                }
                frame "Meas O/P freq. at TP15 wrt TP4" {
                  (unwired) 74700.0 ("Min")
                  (unwired) 91300.0 ("Max")
                  n1181 = call "CompareMaxMin.vi"("Min"=82998.0, "X"=w1954, "Max"=83002.0) -> ("OutCompare"=w1955:bool)
                }
                frame "Meas duty cycle at TP15 wrt TP4" {
                  (unwired) 45.0 ("Min")
                  (unwired) 55.0 ("Max")
                  n1182 = call "CompareMaxMin.vi"("Min"=49.8, "X"=w1958, "Max"=50.2) -> ("OutCompare"=w1959:bool)
                }
                frame "Meas phase between TP14 and TP15" {
                  (unwired) 89.8 ("Min")
                  (unwired) 90.2 ("Max")
                  n1183 = call "CompareMaxMin.vi"("Min"=81.0, "X"=w1962, "Max"=99.0) -> ("OutCompare"=w1963:bool)
                }
                frame "Meas duty cycle at TP14 wrt TP4" {
                  (unwired) 55.0 ("Max")
                  (unwired) 45.0 ("Min")
                  n1184 = call "CompareMaxMin.vi"("Min"=49.8, "X"=w1966, "Max"=50.2) -> ("OutCompare"=w1967:bool)
                }
              }
              n1185 = local read "Description"() -> (w1906:string)
              n1186 = Equal?(x=w1920, y=30) -> (x = y?=w1918:bool)
              n1187 = Or(x=w1916, y=w1915) -> (x .or. y?=w1917:bool)
              n1188 = case shown="\"Meas voltage that will deop either 0 to 0.3 or 5.4 to 5.8V\"" w1906 {
                tunnel: w1904 -> [w1933 w1935 w1937]
                frame "False", Default {
                  n1189 = local write "Result(DecimalPoint)"(w1933) -> ()
                }
                frame "Meas voltage that will deop either 0 to 0.3 or 5.4 to 5.8V" {
                  n1190 = Absolute Value(x=w1935) -> (abs(x)=w1934:dbl)
                  n1191 = local write "Result(DecimalPoint)"(w1934) -> ()
                }
                frame "Meas phase between TP14 and TP15" {
                  n1192 = Absolute Value(x=w1937) -> (abs(x)=w1936:dbl)
                  n1193 = local write "Result(DecimalPoint)"(w1936) -> ()
                }
              }
              n1194 = Or(x=w1917, y=w1918) -> (x .or. y?=w1909:bool)
              n1195 = case shown="False" w1909 {
                tunnel: [w1969 w1970] -> w1910
                tunnel: w1909 -> [w1969 w1970]
                frame False {
                  # "250"
                  n1196 = Wait (ms)(milliseconds to wait=u32 150) -> ()  [unwired: 1 out]
                }
                frame True {
                }
              }
              "Numeric" <- w1920
            }
            n1197 = case shown="False" w1902 {
              tunnel: w1903 -> [w2025 w2032]
              frame False {
                n1198 = local read "Description"() -> (w2024:string)
                n1199 = case shown="\"CHECK WF IS NULL?\"" w2024 {
                  tunnel: w2025 -> [w2026 w2028 w2030]
                  frame "False", Default {
                    n1200 = Enqueue Element(queue=w2026, element="COMPARE") -> ()  [unwired: 1 in, 4 out]
                  }
                  frame "WAVE FORM IS NULL?" {
                    n1201 = Enqueue Element(queue=w2028, element="START") -> ()  [unwired: 1 in, 4 out]
                  }
                  frame "CHECK WF IS NULL?" {
                    n1202 = Enqueue Element(queue=w2030, element="START") -> ()  [unwired: 1 in, 4 out]
                  }
                }
              }
              frame True {
                n1203 = Enqueue Element(queue=w2032, element="START") -> ()  [unwired: 1 in, 4 out]
              }
            }
          }
          frame "DSO1072B_ID-PULSE" {
            n1204 = local read "CMD"() -> (w2035:string)
            n1205 = case shown="\"False\", Default" w2035 {
              tunnel: [TRUE TRUE TRUE FALSE FALSE] -> w2034
              frame "False", Default {
              }
              frame "DSO1072B" {
                n1206 = flat-sequence {
                  frame #0 {
                    n1207 = call "Test ID pulse.vi"() -> ("PWIDTH"=→"PWIDTH":dbl, "MAX AMP"=→"MAX AMP":dbl)  [unwired: 10 in]
                  }
                }
              }
              frame "COMPANSATE MOTOR" {
                n1208 = call "Compensate direction motor.vi"() -> ()  [unwired: 12 in]
              }
              frame "ID-PULSE_VOLTAGE" {
                n1209 = local read "MAX AMP"() -> (w2047:dbl)
                n1210 = local write "Result(DecimalPoint)"(w2047) -> ()
              }
              frame "ID-PULSE_TIME" {
                n1211 = local read "PWIDTH"() -> (w2049:dbl)
                n1212 = local write "Result(DecimalPoint)2"(w2049) -> ()
              }
            }
            n1213 = case shown="False" w2034 {
              tunnel: w2036 -> [w2037 w2039]
              frame False {
                n1214 = Enqueue Element(queue=w2037, element="COMPARE") -> ()  [unwired: 1 in, 4 out]
              }
              frame True {
                n1215 = Enqueue Element(queue=w2039, element="START") -> ()  [unwired: 1 in, 4 out]
              }
            }
          }
          frame "DSO1072B_HALL_WF" {
            n1216 = local read "CMD"() -> (w2052:string)
            n1217 = case shown="\"GET_WF_CW\"" w2052 {
              tunnel: [TRUE TRUE TRUE FALSE FALSE FALSE FALSE] -> w2050
              frame "False", Default {
              }
              frame "GET_WF_CW" {
                n1218 = local read "Result(DecimalPoint)"() -> (w2060:sgl)
                n1219 = Greater Or Equal?(x=w2060, y=sgl 9.9e+30) -> (x >= y?=w2059:bool)
                n1220 = case shown="False" w2059 {
                  frame False {
                    n1221 = local read "DSO1052B"() -> (w2063:refnum<visa-resource-name>)
                    n1222 = call "DSO1072B_FeatchWaveCW.vi"("VISA resource name In"=w2063) -> ("Avg4V8"=→"Avg4V8":dbl, "Avg2V9"=→"Avg2V9":dbl, "Avg2V1"=→"Avg2V1":dbl, "Avg1V3"=→"Avg1V3":dbl, "XY Graph CH1"=→"WF_CW":cluster{"Numeric":dbl, "Numeric":dbl}[])  [unwired: 6 in]
                  }
                  frame True {
                    w2068 = 0.0 ("Avg1V3")
                    n1223 = local write "Avg1V3"(w2068) -> ()
                    n1224 = local write "Avg4V8"(w2068) -> ()
                    n1225 = local write "Avg2V1"(w2068) -> ()
                    n1226 = local write "Avg2V9"(w2068) -> ()
                  }
                }
              }
              frame "GET_WF_CCW" {
                n1227 = local read "DSO1052B"() -> (w2071:refnum<visa-resource-name>)
                n1228 = call "DSO1072B_FeatchWaveCCW.vi"("VISA resource name In"=w2071) -> ("Avg4V8"=w2072:dbl, "Avg2V9"=w2073:dbl, "Avg2V1"=w2074:dbl, "Avg1V3"=w2075:dbl, "XY Graph CH1"=→"WF_CCW":cluster{"Numeric":dbl, "Numeric":dbl}[])  [unwired: 6 in]
                n1229 = local write "Avg2V1"(w2074) -> ()
                n1230 = local write "Avg4V8"(w2072) -> ()
                n1231 = local write "Avg1V3"(w2075) -> ()
                n1232 = local write "Avg2V9"(w2073) -> ()
              }
              frame "2V9" {
                n1233 = local read "Avg2V9"() -> (w2077:dbl)
                n1234 = local write "Result(DecimalPoint)"(w2077) -> ()
              }
              frame "1V3" {
                n1235 = local read "Avg1V3"() -> (w2079:dbl)
                n1236 = local write "Result(DecimalPoint)"(w2079) -> ()
              }
              frame "2V1" {
                n1237 = local read "Avg2V1"() -> (w2081:dbl)
                n1238 = local write "Result(DecimalPoint)"(w2081) -> ()
              }
              frame "4V8" {
                n1239 = local read "Avg4V8"() -> (w2083:dbl)
                n1240 = local write "Result(DecimalPoint)"(w2083) -> ()
              }
            }
            n1241 = case shown="False" w2050 {
              tunnel: w2051 -> [w2053 w2055]
              frame False {
                n1242 = Enqueue Element(queue=w2053, element="COMPARE") -> ()  [unwired: 1 in, 4 out]
              }
              frame True {
                n1243 = Enqueue Element(queue=w2055, element="START") -> ()  [unwired: 1 in, 4 out]
              }
            }
          }
          frame "STK500" {
            (unwired) "cmd /c DL12progapp.bat" ("command line")
            (unwired) "cmd /c progtestsw.bat" ("command line")
            n1244 = local read "CMD"() -> (w2091:string)
            n1245 = case shown="\"APP_FW\"" w2091 {
              tunnel: "cmd /c DL12_ProgTestSw_SVI005.bat" ("command line") -> [_ w2118 _]
              tunnel: [w2113 w2116 w2137] -> w2093
              tunnel: ["" ("standard error") w2117 w2138] -> w2092
              tunnel: "DL12_ProgAppSw_SVI005.bat" ("command line") -> [_ _ w2136]
              tunnel: [w2113 w2116 w2137] -> w2090
              tunnel: [path "C:/Program Files/Atmel/AVR Tools/STK500_2ndTester_DL12" ("working directory") w2115 w2135] -> w2086
              frame "False", Default {
                (unwired) path "C:/Program Files/Atmel/AVR Tools/STK500" ("working directory")
                w2113 = "" ("standard output")
              }
              frame "TEST_FW" {
                n1246 = stacked-sequence {
                  tunnel: w2118 -> [_ w2120 _]
                  tunnel: [_ w2123 _] -> w2117
                  tunnel: [_ w2122 _] -> w2116
                  tunnel: [_ w2119 _] -> w2115
                  frame #0 {
                  }
                  frame #1 {
                    w2119 = path "C:/Program Files/Atmel/AVR Tools/STK500_2ndTester_DL12" ("working directory")
                    (unwired) path "C:/Program Files/Atmel/AVR Tools/STK500" ("working directory")
                    n1247 = call <vilib>:"System Exec.vi"("wait until completion? (T)"=TRUE, "working directory"=w2119, "standard input"=w2120, "command line"=w2120) -> ("standard error"=w2123:string, "standard output"=w2122:string)  [unwired: 4 in, 2 out]
                  }
                  frame #2 {
                    n1248 = local read "TESTING HEAD#"() -> (w2124:string)
                    n1249 = case shown="\"HEAD2\"" w2124 {
                      frame "False", Default {
                      }
                      frame "HEAD1" {
                        n1250 = while {
                          i -> [w2129]
                          stop <- w2126 stop-if-true
                          n1251 = Wait (ms)(milliseconds to wait=u32 1) -> ()  [unwired: 1 out]
                          n1252 = property on="SERIAL NUMBER HEAD 2" class="Str"("Key Focus"=TRUE) -> ()  [unwired: 2 in, 2 out]
                          n1253 = Equal?(x=w2129, y=5) -> (x = y?=w2126:bool)
                        }
                      }
                      frame "HEAD2" {
                        n1254 = while {
                          i -> [w2133]
                          stop <- w2130 stop-if-true
                          n1255 = Wait (ms)(milliseconds to wait=u32 1) -> ()  [unwired: 1 out]
                          n1256 = property on="SERIAL NUMBER HEAD 1" class="Str"("Key Focus"=TRUE) -> ()  [unwired: 2 in, 2 out]
                          n1257 = Equal?(x=w2133, y=5) -> (x = y?=w2130:bool)
                        }
                      }
                    }
                  }
                }
              }
              frame "APP_FW" {
                n1258 = stacked-sequence {
                  tunnel: [w2142 _] -> w2138
                  tunnel: [w2141 _] -> w2137
                  tunnel: w2136 -> [w2140 _]
                  tunnel: [w2139 _] -> w2135
                  frame #0 {
                    n1259 = flat-sequence {
                      tunnel: w2140 -> [w2145]
                      tunnel: [w2145] -> w2143
                      tunnel: [w2153] -> w2142
                      tunnel: [w2152] -> w2141
                      tunnel: [w2150] -> w2139
                      tunnel: w2143 -> [w2151]
                      frame #0 {
                        n1260 = local read "TESTING HEAD#"() -> (w2144:string)
                        n1261 = case shown="\"HEAD2\"" w2144 {
                          frame "False", Default {
                          }
                          frame "HEAD1" {
                          }
                          frame "HEAD2" {
                            # "SWAP TO TEST HEAD 2"
                            n1262 = local read "MUX RELAY"() -> (w2147:refnum<visa-resource-name>)
                            n1263 = call "ControlRelay_ver10.vi"("VISA session"=w2147, "write buffer"="@b013t", "Relay Setting"=T4."Manual Cmd") -> ()  [unwired: 10 in, 7 out]
                          }
                        }
                      }
                      frame #1 {
                        n1264 = case shown="False" FALSE {
                          tunnel: [w2155 w2161] -> w2153
                          tunnel: [w2156 w2160] -> w2152
                          tunnel: w2151 -> [_ w2158]
                          tunnel: [path "C:/Program Files/Atmel/AVR Tools/STK500_2ndTester_DL12" ("working directory") w2157] -> w2150
                          frame False {
                            n1265 = call "PGM APP.vi"() -> ("standard error"=w2155:string, "standard output"=w2156:string)  [unwired: 10 in]
                          }
                          frame True {
                            w2157 = path "C:/Program Files/Atmel/AVR Tools/STK500_2ndTester_DL12" ("working directory")
                            (unwired) path "C:/Program Files/Atmel/AVR Tools/STK500" ("working directory")
                            n1266 = call <vilib>:"System Exec.vi"("wait until completion? (T)"=TRUE, "working directory"=w2157, "standard input"=w2158, "command line"=w2158) -> ("standard error"=w2161:string, "standard output"=w2160:string)  [unwired: 4 in, 2 out]
                          }
                        }
                      }
                    }
                  }
                  frame #1 {
                    n1267 = local read "TESTING HEAD#"() -> (w2162:string)
                    n1268 = case shown="\"HEAD2\"" w2162 {
                      frame "False", Default {
                      }
                      frame "HEAD1" {
                        n1269 = while {
                          i -> [w2167]
                          stop <- w2164 stop-if-true
                          n1270 = Wait (ms)(milliseconds to wait=u32 1) -> ()  [unwired: 1 out]
                          n1271 = property on="SERIAL NUMBER HEAD 2" class="Str"("Key Focus"=TRUE) -> ()  [unwired: 2 in, 2 out]
                          n1272 = Equal?(x=w2167, y=5) -> (x = y?=w2164:bool)
                        }
                      }
                      frame "HEAD2" {
                        n1273 = while {
                          i -> [w2171]
                          stop <- w2168 stop-if-true
                          n1274 = Wait (ms)(milliseconds to wait=u32 1) -> ()  [unwired: 1 out]
                          n1275 = property on="SERIAL NUMBER HEAD 1" class="Str"("Key Focus"=TRUE) -> ()  [unwired: 2 in, 2 out]
                          n1276 = Equal?(x=w2171, y=5) -> (x = y?=w2168:bool)
                        }
                      }
                    }
                  }
                }
              }
            }
            "standard output" <- w2093
            "standard error" <- w2092
            n1277 = case shown="\"APP_FW\"" w2091 {
              tunnel: w2090 -> [_ w2099 _]
              tunnel: ["" ("standard output") w2096 w2107] -> w2089
              tunnel: w2086 -> [_ _ w2104]
              frame "False", Default {
              }
              frame "TEST_FW" {
                w2097 = "Programming complete!" ("standard output")
                n1278 = Match Pattern(string=w2099, regular expression=w2097) -> (match substring=w2098:string)  [unwired: 1 in, 3 out]
                n1279 = Equal?(x=w2098, y=w2097) -> (x = y?=w2095:bool)
                n1280 = case shown="False" w2095 {
                  tunnel: ["Programming failed!" ("standard output") "Programming complete!" ("standard output")] -> w2096
                  frame False {
                  }
                  frame True {
                  }
                }
              }
              frame "APP_FW" {
                w2108 = "Programming complete!" ("standard output")
                n1281 = Build Path(base path=w2104, name or relative path="AppSWdebug.txt") -> (appended path=w2102:path)
                n1282 = Read from Text File(file (use dialog)=w2102) -> (text=w2105:string)  [unwired: 3 in, 3 out]
                n1283 = Match Pattern(string=w2105, regular expression=w2108) -> (match substring=w2109:string)  [unwired: 1 in, 3 out]
                n1284 = Equal?(x=w2109, y=w2108) -> (x = y?=w2106:bool)
                n1285 = case shown="True" w2106 {
                  tunnel: ["Programming failed!" ("standard output") "Programming complete!" ("standard output")] -> w2107
                  frame False {
                  }
                  frame True {
                  }
                }
              }
            }
            n1286 = Enqueue Element(queue=w2087, element="COMPARE") -> ()  [unwired: 1 in, 4 out]
            n1287 = local write "Result(string)"(w2089) -> ()
          }
          frame "VISUAL_INSP" {
            n1288 = local read "CMD"() -> (w2180:string)
            n1289 = local read "Description"() -> (w2179:string)
            n1290 = call "VisualInspection.vi"("Picture Name"=w2180, "MessageIn"=w2179) -> ("Result"=w2178:string)  [unwired: 5 in, 3 out]
            n1291 = Equal?(x=w2178, y="1") -> (x = y?=w2176:bool)
            n1292 = case shown="False" w2176 {
              tunnel: [TRUE FALSE] -> w2175
              frame False {
              }
              frame True {
              }
            }
            n1293 = local write "Result(Boolean) 1"(w2175) -> ()
            n1294 = Enqueue Element(queue=w2173, element="COMPARE") -> ()  [unwired: 1 in, 4 out]
          }
          frame "MESSAGE" {
            n1295 = local read "Description"() -> (w2183:string)
            n1296 = One Button Dialog(message=w2183) -> ()  [unwired: 1 in, 1 out]
            n1297 = Enqueue Element(queue=w2184, element="START") -> ()  [unwired: 1 in, 4 out]
          }
          frame "STATUS DATA" {
            n1298 = flat-sequence {
              tunnel: w2186 -> [w2241]
              frame #0 {
                n1299 = local read "Equipment"() -> (w2189:string)
                n1300 = Equal?(x=w2189, y="RECORD") -> (x = y?=w2187:bool)
                n1301 = case shown="False" w2187 {
                  tunnel: [w2191 TRUE] -> w2190
                  frame False {
                    w2194 = ""
                    n1302 = local read "LowLimit"() -> (w2192:string)
                    n1303 = local read "HighLimit"() -> (w2193:string)
                    n1304 = Not Equal?(x=w2193, y=w2194) -> (x != y?=w2195:bool)
                    n1305 = Not Equal?(x=w2192, y=w2194) -> (x != y?=w2196:bool)
                    n1306 = Or(x=w2195, y=w2196) -> (x .or. y?=w2191:bool)
                  }
                  frame True {
                  }
                }
                n1307 = stacked-sequence {
                  tunnel: w2190 -> [w2198 w2236]
                  frame #0 {
                    n1308 = case shown="True" w2198 {
                      frame False {
                      }
                      frame True {
                        w2210 = "\t"
                        n1309 = local read "Reading >> Sum Disp"() -> (w2201:string)
                        n1310 = local read "Test Step# >> Sum Disp"() -> (w2212:string)
                        n1311 = local read "HighLimit"() -> (w2202:string)
                        n1312 = local read "LowLimit"() -> (w2203:string)
                        n1313 = local read "Status >> Sum Disp"() -> (w2199:string)
                        n1314 = local read "Description"() -> (w2211:string)
                        n1315 = local read "All Test Status in Sum Disp"() -> (w2213:string)
                        n1316 = stacked-sequence {
                          seq-local: [w2214 _] -> [_ w2226]
                          tunnel: w2199 -> [_ w2229]
                          frame #0 {
                            n1317 = local read "SumDisp_Low_Inc"() -> (w2214:i32)
                            n1318 = Greater Or Equal?(x=w2214, y=5) -> (x >= y?=w2218:bool)
                            n1319 = Increment(x=w2214) -> (x+1=w2222:i32)
                            n1320 = Select(t=5 ("y"), s=w2218, f=0 ("y")) -> (s? t:f=w2217:i32)
                            n1321 = local write "SumDisp_Low_Inc"(w2222) -> ()
                            n1322 = Subtract(x=w2222, y=w2217) -> (x-y=w2220:i32)
                            n1323 = Bundle(w2220, 0) -> (w2223:cluster{i32, i32})  [unwired: 1 out]
                            n1324 = property on="Summary Display" class="Tbl (strict)"("Active Cell"=w2223, "Index Values"=w2223) -> ()  [unwired: 2 in, 2 out]
                          }
                          frame #1 {
                            n1325 = case shown="\"FAILED\"" w2229 {
                              tunnel: [w2231 w2233 w2235] -> w2227
                              tunnel: w2226 -> [w2231 w2233 w2235]
                              tunnel: [u32 16448250 u32 11075520 u32 16713222] -> w2224
                              frame "False", Default {
                              }
                              frame "PASSED" {
                              }
                              frame "FAILED" {
                              }
                            }
                            n1326 = Bundle("SumDisp_Low_Inc"=w2227, -2) -> (w2228:cluster{"SumDisp_Low_Inc ":i32, i32})  [unwired: 1 out]
                            n1327 = property on="Summary Display" class="Tbl (strict)"("Active Cell"=w2228, "Cell BG Color"=w2224) -> ()  [unwired: 2 in, 2 out]
                          }
                        }
                        n1328 = local write "LWL"(w2203) -> ()
                        n1329 = local write "UPL"(w2202) -> ()
                        n1330 = local write "Reading"(w2201) -> ()
                        n1331 = Concatenate Strings(w2213, w2212, w2210, w2211, w2210, w2201, w2210, w2203, w2210, w2202, w2210, w2199, "\r\n") -> (w2204:string)
                        n1332 = local write "All Test Status in Sum Disp"(w2204) -> ()
                        n1333 = Initialize Array("") -> (w2206:string[][])  [unwired: 2 out]
                        n1334 = Spreadsheet String To Array(delimiter (Tab)="\t", format string="%s", spreadsheet string=w2204, array type (2D Dbl)=w2206) -> (array=w2200:string[][])
                        n1335 = local write "Summary Display"(w2200) -> ()
                      }
                    }
                  }
                  frame #1 {
                    n1336 = case shown="True" w2236 {
                      frame False {
                      }
                      frame True {
                      }
                    }
                  }
                }
              }
              frame #1 {
                n1337 = local read "Status >> Sum Disp"() -> (w2238:string)
                n1338 = To Upper Case(1:w2238) -> (0:w2239:string)
                n1339 = Equal?(x=w2239, y="FAILED") -> (x = y?=w2237:bool)
                n1340 = case shown="True" w2237 {
                  tunnel: w2241 -> [w2243 w2247]
                  frame False {
                    w2242 = "" ("Test Step# >> Sum Disp")
                    n1341 = local read "Test Modes"() -> (w2244:enum32{"Auto", "Step"})
                    n1342 = local write "Test Step# >> Sum Disp"(w2242) -> ()
                    n1343 = local write "Description"(w2242) -> ()
                    n1344 = local write "Reading >> Sum Disp"(w2242) -> ()
                    n1345 = local write "HighLimit"(w2242) -> ()
                    n1346 = local write "LowLimit"(w2242) -> ()
                    n1347 = local write "Status >> Sum Disp"(w2242) -> ()
                    n1348 = case shown="\"Auto\", Default" w2244 {
                      tunnel: w2243 -> [w2245 _]
                      frame "Auto", Default {
                        n1349 = Enqueue Element(queue=w2245, element="START") -> ()  [unwired: 1 in, 4 out]
                      }
                      frame "Step" {
                      }
                    }
                    n1350 = local write "COMPST"(w2242) -> ()
                  }
                  frame True {
                    n1351 = stacked-sequence {
                      tunnel: w2247 -> [_ w2287]
                      frame #0 {
                        w2250 = "FAILED" ("Caption.Text")
                        w2249 = cluster{u32, u32}[] [{16711680, 16711680}] ("Colors [4]")
                        w2264 = "" ("Test Step# >> Sum Disp")
                        n1352 = local read "TESTING HEAD#"() -> (w2248:string)
                        n1353 = local read "FailedCdDisp"() -> (w2252:string)
                        n1354 = local read "FailedStep"() -> (w2260:string)
                        n1355 = Equal?(x=w2252, y="") -> (x = y?=w2255:bool)
                        n1356 = Equal?(x=w2260, y="") -> (x = y?=w2258:bool)
                        n1357 = case shown="True" w2255 {
                          tunnel: [w2271 w2272] -> w2256
                          frame False {
                            n1358 = local read "FailedCode"() -> (w2269:string)
                            n1359 = Concatenate Strings(",", w2269) -> (w2271:string)
                          }
                          frame True {
                            n1360 = local read "FailedCode"() -> (w2272:string)
                          }
                        }
                        n1361 = local write "PASS/FAIL STATUS"(FALSE ("PASS/FAIL STATUS LED")) -> ()
                        n1362 = case shown="True" w2258 {
                          tunnel: [w2275 w2276] -> w2257
                          frame False {
                            n1363 = local read "Step#"() -> (w2273:string)
                            n1364 = Concatenate Strings(",", w2273) -> (w2275:string)
                          }
                          frame True {
                            n1365 = local read "Step#"() -> (w2276:string)
                          }
                        }
                        n1366 = local read "FailedFlag"() -> (w2263:i8)
                        n1367 = property on="PASS/FAIL STATUS" class="Bool (strict)"("Colors [4]"=w2249, "Caption.Text"=w2250) -> ()  [unwired: 2 in, 2 out]
                        n1368 = local write "UNIT  PASS/FAIL STATUS"(w2250) -> ()
                        n1369 = Increment(x=w2263) -> (x+1=w2262:i8)
                        n1370 = local write "FailedFlag"(w2262) -> ()
                        n1371 = Concatenate Strings(w2252, w2256) -> (w2253:string)
                        n1372 = Concatenate Strings(w2260, w2257) -> (w2261:string)
                        n1373 = case shown="\"HEAD2\"" w2248 {
                          tunnel: w2249 -> [_ w2266 w2268]
                          tunnel: w2250 -> [_ w2265 w2267]
                          frame "False", Default {
                          }
                          frame "HEAD1" {
                            n1374 = property on="PASS/FAIL STATUS  HEAD 1" class="Bool (strict)"("Colors [4]"=w2266, "Caption.Text"=w2265) -> ()  [unwired: 2 in, 2 out]
                          }
                          frame "HEAD2" {
                            n1375 = property on="PASS/FAIL STATUS  HEAD 2" class="Bool (strict)"("Colors [4]"=w2268, "Caption.Text"=w2267) -> ()  [unwired: 2 in, 2 out]
                          }
                        }
                        n1376 = local write "FailedCdDisp"(w2253) -> ()
                        n1377 = local write "HighLimit"(w2264) -> ()
                        n1378 = local write "FailedStep"(w2261) -> ()
                        n1379 = local write "Test Step# >> Sum Disp"(w2264) -> ()
                        n1380 = local write "Reading >> Sum Disp"(w2264) -> ()
                        n1381 = local write "LowLimit"(w2264) -> ()
                        n1382 = local write "Status >> Sum Disp"(w2264) -> ()
                        n1383 = local write "COMPST"(w2264) -> ()
                      }
                      frame #1 {
                        w2297 = "\r\n"
                        n1384 = local read "Step&Description"() -> (w2278:string)
                        n1385 = local read "FailedCode"() -> (w2281:string)
                        n1386 = local read "UPL"() -> (w2293:string)
                        n1387 = local read "LWL"() -> (w2295:string)
                        n1388 = local read "Reading"() -> (w2291:string)
                        n1389 = Concatenate Strings(w2281, ":" ("string")) -> (w2279:string)
                        n1390 = Concatenate Strings(w2279, w2278) -> (w2277:string)
                        n1391 = Concatenate Strings("UPL=", w2293) -> (w2282:string)
                        n1392 = Concatenate Strings("LWL=", w2295) -> (w2283:string)
                        n1393 = local read "Fail Test Param"() -> (w2284:string)
                        n1394 = case shown="False" "RunAllSeq?" {
                          tunnel: ["SAVE LOG FILE" "START"] -> w2286
                          frame False {
                          }
                          frame True {
                          }
                        }
                        n1395 = Concatenate Strings(w2277, "=", w2291, w2297, w2283, ", " ("string"), w2282, w2297) -> (w2288:string)
                        n1396 = Concatenate Strings(w2284, w2288) -> (w2289:string)
                        n1397 = local write "Fail Test Param"(w2289) -> ()
                        n1398 = Enqueue Element(queue=w2287, element=w2286) -> ()  [unwired: 1 in, 4 out]
                      }
                    }
                  }
                }
              }
            }
          }
          frame "COMPARE" {
            (unwired) "0.012" ("HighLimit")
            n1399 = local read "Result(DecimalPoint)"() -> (w2306:sgl)
            n1400 = local read "Result(DecimalPoint)2"() -> (w2305:dbl)
            n1401 = local read "Result(Boolean) 1"() -> (w2309:bool)
            n1402 = local read "Result(Boolean) 2"() -> (w2303:bool)
            n1403 = local read "Result(Boolean) 4"() -> (w2301:bool)
            n1404 = local read "Result(Boolean) 3"() -> (w2302:bool)
            n1405 = local read "Result(Boolean)"() -> (w2300:bool)
            n1406 = local read "Result(Number)2"() -> (w2304:i32)
            n1407 = local read "Result(Number)"() -> (w2308:i32)
            n1408 = local read "Result(string)"() -> (w2314:string)
            n1409 = local read "VAR_TYPE"() -> (w2307:string)
            n1410 = local read "LowLimit"() -> (w2315:string)
            n1411 = local read "HighLimit"() -> (w2316:string)
            n1412 = case shown="\"BLE\"" w2307 {
              tunnel: w2316 -> [_ w2327 w2340 w2348 w2358 w2368 w2381 _ _ w2408 w2416 w2424 _ w2438 _ _ _ _ _]
              tunnel: w2315 -> [_ _ _ _ _ _ w2380 _ _ w2407 w2415 w2423 _ _ w2444 w2447 _ w2452 w2454]
              tunnel: [_ w2326 w2339 w2347 w2357 w2367 w2375 w2386 w2395 w2402 w2412 w2420 w2430 w2435 w2441 w2446 TRUE ("OutCompare") w2451 w2453] -> w2317
              tunnel: w2314 -> [_ _ _ _ _ _ _ _ _ _ _ _ _ _ _ w2445 _ w2450 w2456]
              tunnel: [_ w2324 w2335 w2345 w2355 w2365 w2373 w2384 w2393 w2401 w2409 w2418 w2428 w2436 w2442 w2445 w2449 w2450 w2456] -> w2312
              tunnel: w2309 -> [_ w2323 _ _ _ _ _ _ _ _ _ _ _ _ _ _ _ _ _]
              tunnel: w2308 -> [_ _ _ _ _ _ w2374 w2385 w2394 _ _ _ _ _ _ _ _ _ _]
              tunnel: w2306 -> [_ _ _ _ _ _ _ _ _ _ w2411 _ _ w2434 w2439 _ _ _ _]
              tunnel: w2305 -> [_ _ _ _ _ _ _ _ _ _ _ w2417 _ _ _ _ _ _ _]
              tunnel: w2304 -> [_ _ _ _ _ _ _ _ _ w2400 _ _ _ _ _ _ _ _ _]
              tunnel: w2303 -> [_ _ _ w2343 _ _ _ _ _ _ _ _ _ _ _ _ _ _ _]
              tunnel: w2302 -> [_ _ _ _ w2353 _ _ _ _ _ _ _ _ _ _ _ _ _ _]
              tunnel: w2301 -> [_ _ _ _ _ w2363 _ _ _ _ _ _ _ _ _ _ _ _ _]
              tunnel: w2300 -> [_ _ w2338 _ _ _ _ _ _ _ _ _ _ _ _ _ _ _ _]
              frame "False", Default {
                n1413 = One Button Dialog(message="WRONG DATA TYPE!!!") -> ()  [unwired: 1 in, 1 out]
              }
              frame "BLE1" {
                # "F"
                # "T"
                n1414 = Not(x=w2323) -> (.not. x?=w2322:bool)
                n1415 = case shown="\"1\"" w2327 {
                  tunnel: [_ FALSE TRUE] -> w2325
                  frame "False", Default {
                  }
                  frame "0" {
                  }
                  frame "1" {
                  }
                }
                n1416 = case shown="False" w2322 {
                  tunnel: ["0" "1"] -> w2324
                  frame False {
                  }
                  frame True {
                  }
                }
                n1417 = Equal?(x=w2325, y=w2322) -> (x = y?=w2326:bool)
              }
              frame "BLE" {
                # "0"
                # "F"
                # "T"
                n1418 = local read "HighLimit"() -> (w2334:string)
                n1419 = Not Equal?(x=w2334, y="0") -> (x != y?=w2332:bool)
                n1420 = Select(t="1", s=w2338, f="0") -> (s? t:f=w2335:string)
                n1421 = case shown="\"1\"" w2340 {
                  tunnel: [_ FALSE TRUE] -> _
                  frame "False", Default {
                  }
                  frame "0" {
                  }
                  frame "1" {
                  }
                }
                n1422 = Equal?(x=w2332, y=w2338) -> (x = y?=w2339:bool)
              }
              frame "BLE2" {
                n1423 = Not(x=w2343) -> (.not. x?=w2344:bool)
                n1424 = case shown="\"1\"" w2348 {
                  tunnel: [_ FALSE TRUE] -> w2346
                  frame "False", Default {
                  }
                  frame "0" {
                  }
                  frame "1" {
                  }
                }
                n1425 = case shown="True" w2344 {
                  tunnel: ["0" "1"] -> w2345
                  frame False {
                  }
                  frame True {
                  }
                }
                n1426 = Equal?(x=w2346, y=w2344) -> (x = y?=w2347:bool)
              }
              frame "BLE3" {
                n1427 = case shown="\"1\"" w2358 {
                  tunnel: [_ FALSE TRUE] -> w2356
                  frame "False", Default {
                  }
                  frame "0" {
                  }
                  frame "1" {
                  }
                }
                n1428 = Not(x=w2353) -> (.not. x?=w2354:bool)
                n1429 = case shown="True" w2354 {
                  tunnel: ["0" "1"] -> w2355
                  frame False {
                  }
                  frame True {
                  }
                }
                n1430 = Equal?(x=w2356, y=w2354) -> (x = y?=w2357:bool)
              }
              frame "BLE4" {
                n1431 = case shown="\"1\"" w2368 {
                  tunnel: [_ FALSE TRUE] -> w2366
                  frame "False", Default {
                  }
                  frame "0" {
                  }
                  frame "1" {
                  }
                }
                n1432 = Not(x=w2363) -> (.not. x?=w2364:bool)
                n1433 = case shown="True" w2364 {
                  tunnel: ["0" "1"] -> w2365
                  frame False {
                  }
                  frame True {
                  }
                }
                n1434 = Equal?(x=w2366, y=w2364) -> (x = y?=w2367:bool)
              }
              frame "INT1" {
                n1435 = Decimal String To Number(string=w2381) -> (number=w2378:i32)  [unwired: 2 in, 1 out]
                n1436 = Decimal String To Number(string=w2380) -> (number=w2379:i32)  [unwired: 2 in, 1 out]
                n1437 = Greater Or Equal?(x=w2374, y=w2379) -> (x >= y?=w2377:bool)
                n1438 = Less Or Equal?(x=w2374, y=w2378) -> (x <= y?=w2376:bool)
                n1439 = And(x=w2377, y=w2376) -> (x .and. y?=w2375:bool)
                n1440 = Number To Decimal String(number=w2374) -> (decimal integer string=w2373:string)  [unwired: 1 in]
              }
              frame "INT1_InitialValue+400" {
                n1441 = local read "HighLimitForPulseCnt+400"() -> (w2383:string)
                n1442 = local read "LowLimitForPulseCnt+400"() -> (w2382:string)
                n1443 = Decimal String To Number(string=w2382) -> (number=w2390:i32)  [unwired: 2 in, 1 out]
                n1444 = Decimal String To Number(string=w2383) -> (number=w2389:i32)  [unwired: 2 in, 1 out]
                n1445 = Greater Or Equal?(x=w2385, y=w2390) -> (x >= y?=w2388:bool)
                n1446 = Less Or Equal?(x=w2385, y=w2389) -> (x <= y?=w2387:bool)
                n1447 = And(x=w2388, y=w2387) -> (x .and. y?=w2386:bool)
                n1448 = Number To Decimal String(number=w2385) -> (decimal integer string=w2384:string)  [unwired: 1 in]
              }
              frame "INT1_InitialValue" {
                n1449 = local read "HighLimitForIntValue"() -> (w2392:string)
                n1450 = local read "LowLimitForIntValue"() -> (w2391:string)
                n1451 = Decimal String To Number(string=w2391) -> (number=w2399:i32)  [unwired: 2 in, 1 out]
                n1452 = Decimal String To Number(string=w2392) -> (number=w2398:i32)  [unwired: 2 in, 1 out]
                n1453 = Greater Or Equal?(x=w2394, y=w2399) -> (x >= y?=w2397:bool)
                n1454 = Less Or Equal?(x=w2394, y=w2398) -> (x <= y?=w2396:bool)
                n1455 = And(x=w2397, y=w2396) -> (x .and. y?=w2395:bool)
                n1456 = Number To Decimal String(number=w2394) -> (decimal integer string=w2393:string)  [unwired: 1 in]
              }
              frame "INT2" {
                n1457 = Decimal String To Number(string=w2408) -> (number=w2405:i32)  [unwired: 2 in, 1 out]
                n1458 = Decimal String To Number(string=w2407) -> (number=w2406:i32)  [unwired: 2 in, 1 out]
                n1459 = Greater Or Equal?(x=w2400, y=w2406) -> (x >= y?=w2404:bool)
                n1460 = Less Or Equal?(x=w2400, y=w2405) -> (x <= y?=w2403:bool)
                n1461 = And(x=w2404, y=w2403) -> (x .and. y?=w2402:bool)
                n1462 = Number To Decimal String(number=w2400) -> (decimal integer string=w2401:string)  [unwired: 1 in]
              }
              frame "DPO1" {
                n1463 = Fract/Exp String To Number(string=w2416) -> (number=w2414:dbl)  [unwired: 4 out]
                n1464 = Fract/Exp String To Number(string=w2415) -> (number=w2413:dbl)  [unwired: 4 out]
                n1465 = call "CompareMaxMin.vi"("Min"=w2413, "X"=w2411, "Max"=w2414) -> ("OutCompare"=w2412:bool)
                n1466 = Number To Fractional String(number=w2411, precision (6)=i16 4) -> (F-format string=w2409:string)  [unwired: 2 in]
              }
              frame "DPO2" {
                n1467 = Fract/Exp String To Number(string=w2424) -> (number=w2422:dbl)  [unwired: 4 out]
                n1468 = Fract/Exp String To Number(string=w2423) -> (number=w2421:dbl)  [unwired: 4 out]
                n1469 = call "CompareMaxMin.vi"("Min"=w2421, "X"=w2417, "Max"=w2422) -> ("OutCompare"=w2420:bool)
                n1470 = Number To Fractional String(number=w2417, precision (6)=i16 3) -> (F-format string=w2418:string)  [unwired: 2 in]
              }
              frame "SSI_LIMIT" {
                n1471 = local read "Position Get SSI-Neg*-1"() -> (w2425:sgl)
                n1472 = local read "SSI_HighLimit"() -> (w2427:string)
                n1473 = local read "SSI_LowLimit"() -> (w2426:string)
                n1474 = Fract/Exp String To Number(string=w2426) -> (number=w2431:dbl)  [unwired: 4 out]
                n1475 = Fract/Exp String To Number(string=w2427) -> (number=w2432:dbl)  [unwired: 4 out]
                n1476 = call "CompareMaxMin.vi"("Min"=w2431, "X"=w2425, "Max"=w2432) -> ("OutCompare"=w2430:bool)
                n1477 = Number To Fractional String(number=w2425, precision (6)=i16 3) -> (F-format string=w2428:string)  [unwired: 2 in]
              }
              frame "DPO_LESSTHAN" {
                n1478 = Fract/Exp String To Number(string=w2438) -> (number=w2433:dbl)  [unwired: 4 out]
                n1479 = Less Or Equal?(x=w2434, y=w2433) -> (x <= y?=w2435:bool)
                n1480 = Number To Fractional String(number=w2434, precision (6)=i16 3) -> (F-format string=w2436:string)  [unwired: 2 in]
              }
              frame "DPO_GREATHERTHAN" {
                n1481 = Fract/Exp String To Number(string=w2444) -> (number=w2440:dbl)  [unwired: 4 out]
                n1482 = Greater Or Equal?(x=w2439, y=w2440) -> (x >= y?=w2441:bool)
                n1483 = Number To Fractional String(number=w2439, precision (6)=i16 3) -> (F-format string=w2442:string)  [unwired: 2 in]
              }
              frame "STR1" {
                n1484 = Equal?(x=w2445, y=w2447) -> (x = y?=w2446:bool)
                "LowLimit 2" <- w2447
              }
              frame "NOTE" {
                n1485 = local read "NOTE"() -> (w2449:string)
              }
              frame "STR2" {
                n1486 = Equal?(x=w2450, y=w2452) -> (x = y?=w2451:bool)
              }
              frame "STR3" {
                n1487 = Match Pattern(string=w2456, regular expression=w2454) -> (match substring=w2455:string)  [unwired: 1 in, 3 out]
                n1488 = Equal?(x=w2455, y=w2454) -> (x = y?=w2453:bool)
              }
            }
            n1489 = local read "LineLogFile"() -> (w2310:string)
            n1490 = case shown="True" w2317 {
              tunnel: ["FAILED" ("element") "PASSED" ("element")] -> w2318
              frame False {
              }
              frame True {
              }
            }
            n1491 = Concatenate Strings(w2310, ";" ("string"), w2312) -> (w2311:string)
            n1492 = local write "Reading >> Sum Disp"(w2312) -> ()
            n1493 = local write "LineLogFile"(w2311) -> ()
            n1494 = local write "Status >> Sum Disp"(w2318) -> ()
            n1495 = Enqueue Element(queue=w2319, element="STATUS DATA") -> ()  [unwired: 1 in, 4 out]
          }
          frame "RECORD" {
            n1496 = local read "Result(DecimalPoint)"() -> (w2464:sgl)
            n1497 = local read "Result(DecimalPoint)2"() -> (w2463:dbl)
            n1498 = local read "Result(Boolean) 1"() -> (w2467:bool)
            n1499 = local read "Result(Boolean) 2"() -> (w2461:bool)
            n1500 = local read "Result(Boolean) 4"() -> (w2459:bool)
            n1501 = local read "Result(Boolean) 3"() -> (w2460:bool)
            n1502 = local read "Result(Number)2"() -> (w2462:i32)
            n1503 = local read "Result(Number)"() -> (w2466:i32)
            n1504 = local read "Result(string)"() -> (w2472:string)
            n1505 = local read "VAR_TYPE"() -> (w2465:string)
            n1506 = case shown="\"INT1\"" w2465 {
              tunnel: w2472 -> [_ _ _ _ _ _ _ _ _ w2506 w2507]
              tunnel: [_ w2478 w2483 w2488 w2493 w2496 w2499 w2500 w2504 w2506 w2507] -> w2470
              tunnel: w2467 -> [_ w2477 _ _ _ _ _ _ _ _ _]
              tunnel: w2466 -> [_ _ _ _ _ w2497 _ _ _ _ _]
              tunnel: w2464 -> [_ _ _ _ _ _ _ w2502 _ _ _]
              tunnel: w2463 -> [_ _ _ _ _ _ _ _ w2503 _ _]
              tunnel: w2462 -> [_ _ _ _ _ _ w2498 _ _ _ _]
              tunnel: w2461 -> [_ _ w2481 _ _ _ _ _ _ _ _]
              tunnel: w2460 -> [_ _ _ w2486 _ _ _ _ _ _ _]
              tunnel: w2459 -> [_ _ _ _ w2491 _ _ _ _ _ _]
              frame "False", Default {
                n1507 = One Button Dialog(message="WRONG DATA TYPE!!!") -> ()  [unwired: 1 in, 1 out]
              }
              frame "BLE1" {
                n1508 = Not(x=w2477) -> (.not. x?=w2476:bool)
                n1509 = case shown="False" w2476 {
                  tunnel: ["0" "1"] -> w2478
                  frame False {
                  }
                  frame True {
                  }
                }
              }
              frame "BLE2" {
                n1510 = Not(x=w2481) -> (.not. x?=w2482:bool)
                n1511 = case shown="True" w2482 {
                  tunnel: ["0" "1"] -> w2483
                  frame False {
                  }
                  frame True {
                  }
                }
              }
              frame "BLE3" {
                n1512 = Not(x=w2486) -> (.not. x?=w2487:bool)
                n1513 = case shown="True" w2487 {
                  tunnel: ["0" "1"] -> w2488
                  frame False {
                  }
                  frame True {
                  }
                }
              }
              frame "BLE4" {
                n1514 = Not(x=w2491) -> (.not. x?=w2492:bool)
                n1515 = case shown="True" w2492 {
                  tunnel: ["0" "1"] -> w2493
                  frame False {
                  }
                  frame True {
                  }
                }
              }
              frame "INT1" {
                n1516 = Number To Decimal String(number=w2497) -> (decimal integer string=w2496:string)  [unwired: 1 in]
              }
              frame "INT2" {
                n1517 = Number To Decimal String(number=w2498) -> (decimal integer string=w2499:string)  [unwired: 1 in]
              }
              frame "DPO1" {
                n1518 = Number To Fractional String(number=w2502, precision (6)=i16 3) -> (F-format string=w2500:string)  [unwired: 2 in]
              }
              frame "DPO2" {
                n1519 = Number To Fractional String(number=w2503, precision (6)=i16 3) -> (F-format string=w2504:string)  [unwired: 2 in]
              }
              frame "STR1" {
              }
              frame "STR2" {
              }
            }
            n1520 = local read "LineLogFile"() -> (w2468:string)
            n1521 = Concatenate Strings(w2468, ";" ("string"), w2470) -> (w2469:string)
            n1522 = local write "Reading >> Sum Disp"(w2470) -> ()
            n1523 = local write "LineLogFile"(w2469) -> ()
            n1524 = Enqueue Element(queue=w2473, element="STATUS DATA") -> ()  [unwired: 1 in, 4 out]
          }
          frame "SAVE LOG FILE" {
            n1525 = flat-sequence {
              tunnel: [w2511] -> w2508
              tunnel: w2508 -> [w2557]
              frame #0 {
                w2526 = ";" ("y")
                n1526 = local read "Project index"() -> (w2518:i32)
                n1527 = call "MatchProject&GiveLogFile-FileName&Format.vi"("ProjectIndex"=w2518) -> ("CUST P/N"=w2519:string, "FCT_LOG"=w2520:string)  [unwired: 9 out]
                n1528 = local read "Test Time (Sec)"() -> (w2531:dbl)
                n1529 = local read "Serial Number"() -> (w2524:string)
                n1530 = local read "Operator ID"() -> (w2533:string)
                n1531 = local read "UNIT  PASS/FAIL STATUS"() -> (w2511:string)
                n1532 = local read "FailedCdDisp"() -> (w2512:string)
                n1533 = local read "LineLogFile"() -> (w2517:string)
                n1534 = Number To Fractional String(number=w2531, precision (6)=i16 3) -> (F-format string=w2529:string)  [unwired: 2 out]
                "TestTimeStr" <- w2529
                n1535 = local read "StartTime"() -> (w2522:string)
                n1536 = call "WriteSimpleLogFile.vi"("StartTime"=w2522, "Status"=w2511, "SerialNumber"=w2524) -> ("#OfTest"=w2523:string)  [unwired: 8 out]
                n1537 = local read "TESTING HEAD#"() -> (w2513:string)
                n1538 = case shown="False" FALSE {
                  tunnel: w2517 -> [w2541 w2546]
                  tunnel: [w2541 w2542] -> w2516
                  frame False {
                  }
                  frame True {
                    n1539 = Search and Replace String(replace all?=TRUE ("replace all? (F)"), input string=w2546, search string=".", replace string="," ("replace string (\"\")")) -> (result string=w2542:string)  [unwired: 4 in, 3 out]
                  }
                }
                n1540 = local read "LogfileHeaderCSV"() -> (w2525:string)
                n1541 = local read "LogfileHeaderXLS"() -> (w2515:string)
                n1542 = Concatenate Strings("SB" ("string"), w2526, w2519, w2526, w2524, w2526, w2522, w2526, w2523, w2526, w2511, w2526, "Station", w2526, "Fixture/PalletteID", w2526, "TestSoftwareVersion", w2526, w2533, w2526, "Note", w2526, w2512, w2526, w2529, w2526, "Reserve#1", w2526, "Reserve#2", w2516) -> (w2538:string)
                n1543 = case shown="\"HEAD1\"" w2513 {
                  tunnel: w2512 -> [_ w2539 w2540]
                  frame "False", Default {
                  }
                  frame "HEAD1" {
                    n1544 = local write "FailedCdDisp H1"(w2539) -> ()
                  }
                  frame "HEAD2" {
                    n1545 = local write "FailedCdDisp H2"(w2540) -> ()
                  }
                }
                n1546 = stacked-sequence {
                  tunnel: w2538 -> [w2550 w2551]
                  tunnel: w2525 -> [_ w2554]
                  tunnel: TRUE -> [w2549 w2552]
                  tunnel: w2520 -> [w2548 w2553]
                  tunnel: w2515 -> [w2547 _]
                  frame #0 {
                    n1547 = call "SaveExcel.vi"("LogFileHeader"=w2547, "FCT_LOG"=w2548, "Boolean"=w2549, "DataSave"=w2550) -> ()  [unwired: 6 out]
                  }
                  frame #1 {
                    n1548 = call "SaveCSV2.vi"("LogFileHeader"=w2554, "FCT_LOG"=w2553, "Boolean"=w2552, "DataSave"=w2551) -> ()  [unwired: 6 in]
                  }
                }
              }
              frame #1 {
                n1549 = case shown="\"False\", Default" w2557 {
                  tunnel: ["Failed" ("Result") "Passed" ("Result")] -> w2556
                  frame "False", Default {
                  }
                  frame "PASSED" {
                  }
                }
                n1550 = case shown="False" TRUE {
                  tunnel: w2556 -> [w2565 w2576]
                  frame False {
                    # "OCS write new version"
                    n1551 = local read "Serial Number"() -> (w2567:string)
                    n1552 = local read "Project908"() -> (w2558:string)
                    n1553 = Bundle(cluster="DataIn", "W0-SN"=w2567, "W1-CUSTOMER"="LNK" ("Customer"), "W3-TESTER"=w2558, "W4-RESULT"=w2565, "W9-OPNAME"="FCT1") -> (w2563:T1)  [unwired: 13 in]
                    n1554 = local read "Username"() -> (w2559:string)
                    n1555 = disable-structure shown="Disabled" {
                      disable-tunnel: w2563 -> [w2573 _]
                      disable-tunnel: "FCTLOG" ("Table log") -> [w2572 _]
                      disable-tunnel: "OCSAEC" ("OcsThai") -> [w2571 _]
                      disable-tunnel: "True" ("popup") -> [w2570 _]
                      disable-tunnel: w2559 -> [w2569 _]
                      frame Disabled {
                        n1556 = call "OcsWrite.vi"("DataIn"=w2573, "Table log"=w2572, "Operator(False=Dubug)"=w2569, "OcsThai"=w2571, "popup"=w2570) -> ()  [unwired: 21 in, 2 out]
                      }
                      frame Enabled {
                      }
                    }
                  }
                  frame True {
                    # "OCS write old version"
                    n1557 = local read "ProjectFull"() -> (w2581:string)
                    n1558 = local read "Serial Number"() -> (w2577:string)
                    n1559 = Concatenate Strings(w2581, "|" ("OperationWrite"), "LNK1700063" ("Customer")) -> (w2580:string)
                    n1560 = Format Date/Time String(time format string (%c)="%Y/%m/%d %H:%M:%S") -> (date/time string=w2574:string)  [unwired: 2 in]
                    n1561 = disable-structure shown="Disabled" {
                      disable-tunnel: w2580 -> [w2591 _]
                      disable-tunnel: "LNK" ("Customer") -> [w2590 _]
                      disable-tunnel: "FCT1" ("Tester") -> [w2589 _]
                      disable-tunnel: w2577 -> [w2588 _]
                      disable-tunnel: w2576 -> [w2587 _]
                      disable-tunnel: "FCTLOG" ("DatabaseLog") -> [w2586 _]
                      disable-tunnel: w2574 -> [w2585 _]
                      frame Disabled {
                        n1562 = call "OCS_FCTLOC_AEC_Rev1.1.vi"("OPNAME"=w2589, "TEXT1"=w2586, "RESULT"=w2587, "TESTER"=w2591, "TEST_DATE"=w2585, "CUSTOMER"=w2590, "SN"=w2588) -> ()  [unwired: 5 in]
                      }
                      frame Enabled {
                      }
                    }
                  }
                }
              }
            }
            n1563 = Enqueue Element(queue=w2509, element="CLEAR_HW") -> ()  [unwired: 1 in, 4 out]
          }
          frame "SAVE DATABASE" {
          }
          frame "CLEAR_HW" {
            n1564 = flat-sequence {
              frame #0 {
                n1565 = local read "MUX RELAY"() -> (w2599:refnum<visa-resource-name>)
                n1566 = call "ControlRelay_ver10.vi"("VISA session"=w2599, "baud rate (9600)"=u32 19200, "write buffer"="Bb000", "Relay Setting"=T4."Manual Cmd") -> ()  [unwired: 9 in, 7 out]
              }
              frame #1 {
              }
              frame #2 {
                n1567 = case shown="True" FALSE {
                  frame False {
                  }
                  frame True {
                    n1568 = local read "MUX RELAY"() -> (w2603:refnum<visa-resource-name>)
                    n1569 = call "ControlRelay_ver10.vi"("VISA session"=w2603, "write buffer"="Bb000", "Relay Setting"=T4."Manual Cmd") -> ()  [unwired: 10 in, 7 out]
                  }
                }
              }
            }
            n1570 = Enqueue Element(queue=w2595, element="SHOW PASSED/FAILED") -> ()  [unwired: 1 in, 4 out]
          }
          frame "SHOW PASSED/FAILED" {
            (unwired) "BARCODE SCANER" ("element")
            n1571 = case shown="False" FALSE {
              frame False {
                n1572 = local read "UNIT  PASS/FAIL STATUS"() -> (w2609:string)
                n1573 = local read "Fail Test Param"() -> (w2612:string)
                n1574 = local read "TestTimeStr"() -> (w2613:string)
                n1575 = local read "Serial Number"() -> (w2617:string)
                n1576 = local read "Project908"() -> (w2620:string)
                n1577 = Concatenate Strings("F|" ("string"), w2612) -> (w2610:string)
                n1578 = Concatenate Strings("P|TestTime = " ("string"), w2613) -> (w2614:string)
                n1579 = local read "TESTING HEAD#"() -> (w2622:string)
                n1580 = Equal?(x=w2609, y="PASSED") -> (x = y?=w2607:bool)
                n1581 = Select(t=w2614, s=w2607, f=w2610) -> (s? t:f=w2616:string)
                n1582 = Concatenate Strings("LNK1700062-", w2622, "_" ("string"), w2620, "_FCT1-AEC" ("string")) -> (w2618:string)
                n1583 = call "DataInFPYALRev.1.0.vi"("P/F"=w2616, "SN"=w2617, "FixtureName"=w2618) -> ()  [unwired: 9 in]
                n1584 = case shown="\"HEAD1\"" w2622 {
                  frame "False", Default {
                  }
                  frame "HEAD1" {
                    n1585 = disable-structure shown="Disabled" {
                      frame Disabled {
                        w2625 = "" ("Caption.Text")
                        w2626 = cluster{u32, u32}[] [{197379, 197379}] ("Colors [4]")
                        n1586 = property on="PASS/FAIL STATUS" class="Bool (strict)"("Colors [4]"=w2626, "Caption.Text"=w2625) -> ()  [unwired: 2 in, 2 out]
                        n1587 = stacked-sequence {
                          tunnel: w2626 -> [w2628 _]
                          tunnel: w2625 -> [w2627 _]
                          frame #0 {
                            n1588 = property on="PASS/FAIL STATUS  HEAD 2" class="Bool (strict)"("Colors [4]"=w2628, "Caption.Text"=w2627) -> ()  [unwired: 2 in, 2 out]
                          }
                          frame #1 {
                          }
                        }
                      }
                      frame Enabled {
                      }
                    }
                    n1589 = local write "SERIAL NUMBER HEAD 1"("" ("BARCODE HEAD 2")) -> ()
                  }
                  frame "HEAD2" {
                    n1590 = disable-structure shown="Disabled" {
                      frame Disabled {
                        w2630 = "" ("Caption.Text")
                        w2631 = cluster{u32, u32}[] [{197379, 197379}] ("Colors [4]")
                        n1591 = property on="PASS/FAIL STATUS" class="Bool (strict)"("Colors [4]"=w2631, "Caption.Text"=w2630) -> ()  [unwired: 2 in, 2 out]
                        n1592 = stacked-sequence {
                          tunnel: w2631 -> [_ w2633]
                          tunnel: w2630 -> [_ w2632]
                          frame #0 {
                          }
                          frame #1 {
                            n1593 = property on="PASS/FAIL STATUS  HEAD 1" class="Bool (strict)"("Colors [4]"=w2633, "Caption.Text"=w2632) -> ()  [unwired: 2 in, 2 out]
                          }
                        }
                      }
                      frame Enabled {
                      }
                    }
                    n1594 = local write "SERIAL NUMBER HEAD 2"("" ("BARCODE HEAD 2")) -> ()
                  }
                }
              }
              frame True {
                n1595 = local read "FailedFlag"() -> (w2636:i8)
                n1596 = local read "Fail Test Param"() -> (w2634:string)
                n1597 = Equal?(x=w2636, y=i8 0) -> (x = y?=w2637:bool)
                n1598 = case shown="True" w2637 {
                  tunnel: ["FAILED" "PASSED"] -> _
                  tunnel: w2634 -> [w2638 _]
                  frame False {
                    n1599 = flat-sequence {
                      tunnel: w2638 -> [w2640]
                      frame #0 {
                        n1600 = call "PassFail.vi"("Failed: 2"=w2640, "STATUS"=FALSE) -> ()
                      }
                    }
                  }
                  frame True {
                    n1601 = flat-sequence {
                      frame #0 {
                        n1602 = call "PassFail.vi"("STATUS"=TRUE) -> ()  [unwired: 1 in]
                      }
                    }
                  }
                }
              }
            }
            n1603 = Enqueue Element(queue=w2606, element="DUAL-HEAD-TESTING") -> ()  [unwired: 1 in, 4 out]
          }
        }
      }
      n1604 = stacked-sequence {
        frame #0 {
          n1605 = flat-sequence {
            frame #0 {
              n1606 = property on="Break step#" class="CmbBox"("Strings[]"="Clear list of break step") -> ()  [unwired: 2 in, 2 out]
            }
            frame #1 {
              n1607 = Current VI's Path() -> (path=w301:path)
              n1608 = local read "ProjectFull"() -> (w293:string)
              n1609 = Strip Path(path=w301) -> (stripped path=w300:path)  [unwired: 1 out]
              n1610 = Build Path(base path=w300, name or relative path="TestSeqFile") -> (appended path=w298:path)
              n1611 = Concatenate Strings("Seq" ("name or relative path"), w293, ".txt" ("name or relative path")) -> (w294:string)
              "concatenated string" <- w294
              n1612 = Build Path(base path=w298, name or relative path=w294) -> (appended path=w297:path)
              n1613 = File/Directory Info(path=w297) -> (path out=w302:path, error out=w305:errorcluster)  [unwired: 1 in, 5 out]
              n1614 = Unbundle By Name(w305) -> ("status"=w304:bool)
              n1615 = Not(x=w304) -> (.not. x?=w303:bool)
              n1616 = case shown="False" w303 {
                tunnel: w302 -> [_ w324]
                frame False {
                  n1617 = One Button Dialog(message="Test sequence file was not found, Please check!") -> (true=w306:bool)  [unwired: 1 out]
                  n1618 = local write "SeqFileSts"(w306) -> ()
                }
                frame True {
                  w312 = 5 ("index")
                  n1619 = call <vilib>:"Read Characters From File.vi"("file path (dialog if empty)"=w324) -> ("character string"=w319:string)  [unwired: 1 in, 7 out]
                  n1620 = Initialize Array("") -> (w321:string[][])  [unwired: 2 out]
                  n1621 = Spreadsheet String To Array(delimiter (Tab)="\t", format string="%s", spreadsheet string=w319, array type (2D Dbl)=w321) -> (array=w316:string[][])
                  "TESTPLAN ARRAY" <- w316
                  "TESTPLAN ARRAY Display" <- w316
                  n1622 = Transpose 2D Array(2D array=w316) -> (transposed array=w318:string[][])
                  n1623 = Array Size(array=w316) -> (size(s)=w315:i32[])
                  "TestPlanDimensions" <- w315
                  n1624 = Index Array(array=w315, index=0) -> (element=w309:i32)
                  "RowSize" <- w309
                  n1625 = Subtract(x=w309, y=w312) -> (x-y=w313:i32)
                  n1626 = Reshape Array(w318, w309) -> (w317:string[])
                  n1627 = Array Subset(array=w317, index=w312, length=w313) -> (w311:string[])
                  "BreakStep#" <- w311
                  n1628 = property on="Break step#" class="CmbBox"("Strings[]"=w311) -> ()  [unwired: 2 in, 2 out]
                  n1629 = Subtract(x=w309, y=6) -> (x-y=w308:i32)
                  n1630 = property on="HEAD 1" class="Slide (strict)"("Scale.Maximum"=w308) -> ()  [unwired: 2 in, 2 out]
                  n1631 = property on="HEAD 2" class="Slide (strict)"("Scale.Maximum"=w308) -> ()  [unwired: 2 in, 2 out]
                }
              }
            }
            frame #2 {
              n1632 = Initialize Array("") -> (w335:string[][])  [unwired: 2 out]
              n1633 = Bundle(5, 0) -> (w329:cluster{i32, i32})  [unwired: 1 out]
              n1634 = Bundle(0, 0) -> (w325:cluster{i32, i32})  [unwired: 1 out]
              n1635 = Spreadsheet String To Array(delimiter (Tab)="\t", format string="%s", spreadsheet string="", array type (2D Dbl)=w335) -> (array=→"Summary Display":string[][])
              n1636 = property on="TESTPLAN ARRAY Display" class="Tbl (strict)"("Active Cell"=w329, "Index Values"=w329) -> ()  [unwired: 2 in, 2 out]
              n1637 = property on="Summary Display" class="Tbl (strict)"("Active Cell"=w325, "Index Values"=w325) -> ()  [unwired: 2 in, 2 out]
            }
          }
        }
        frame #1 {
          n1638 = stacked-sequence {
            tunnel: [w345 _] -> w342
            tunnel: [_ w370] -> w341
            tunnel: [w343 _] -> w338
            tunnel: [_ w364] -> w337
            frame #0 {
              n1639 = Current VI's Path() -> (path=w355:path)
              n1640 = Strip Path(path=w355) -> (stripped path=w354:path)  [unwired: 1 out]
              n1641 = Build Path(base path=w354, name or relative path="LogFile") -> (appended path=w352:path)
              n1642 = Build Path(base path=w352, name or relative path="Header&Format") -> (appended path=w350:path)
              n1643 = Build Path(base path=w350, name or relative path="GeneralHeaderFormat") -> (appended path=w348:path)
              n1644 = Build Path(base path=w348, name or relative path="GeneralHeaderFormat.txt") -> (appended path=w346:path)
              n1645 = Read from Text File(file (use dialog)=w346) -> (text=w357:string)  [unwired: 1 in, 5 out]
              n1646 = Match Pattern(string=w357, regular expression="\n") -> (before substring=w343:string)  [unwired: 4 out]
              "GeneralHeader" <- w343
              n1647 = case shown="True" TRUE {
                tunnel: w343 -> [w358 w363]
                tunnel: [w358 w359] -> w345
                frame False {
                }
                frame True {
                  n1648 = Search and Replace String(replace all?=TRUE ("replace all? (F)"), input string=w363, search string="\t", replace string=";" ("replace string (\"\")")) -> (result string=w359:string)  [unwired: 4 in, 3 out]
                }
              }
            }
            frame #1 {
              n1649 = local read "TESTPLAN ARRAY"() -> (w366:string[][])
              n1650 = call "GetTestDataHeader.vi"("Boolean"=FALSE, "TESTPLAN ARRAY"=w366) -> ("TestDataHeader"=w368:string)  [unwired: 9 out]
              "TestDataHeader" <- w368
              n1651 = call "GetTestDataHeader.vi"("Boolean"=TRUE, "TESTPLAN ARRAY"=w366) -> ("TestDataHeader"=w364:string)  [unwired: 9 out]
              n1652 = case shown="True" TRUE {
                tunnel: w368 -> [w371 w376]
                tunnel: [w371 w373] -> w370
                frame False {
                }
                frame True {
                  n1653 = Search and Replace String(replace all?=TRUE ("replace all? (F)"), input string=w376, search string=".", replace string="," ("replace string (\"\")")) -> (result string=w373:string)  [unwired: 4 in, 3 out]
                }
              }
            }
          }
          n1654 = Concatenate Strings(w342, w341) -> (→"LogfileHeaderCSV":string)
          n1655 = Concatenate Strings(w338, w337) -> (→"LogfileHeaderXLS":string)
        }
        frame #2 {
          n1656 = while {
            stop <- w379 stop-if-true
            n1657 = event shown="[0] Timeout" {
              selector: _ -> [_ _ _ _ _ _]
              dyn-events: _ -> [_ _ _ _ _ _]
              timeout: _ -> [_ _ _ _ _ _]
              tunnel: [_ w380 _ _ _ _] -> w377
              event Timeout {
                n1658 = event-data() -> ()  [unwired: 3 out]
              }
              event "stop": Value Change {
                n1659 = event-data() -> ()  [unwired: 6 out]
                n1660 = case shown="True" "stop" {
                  selector: "stop" -> [_ w383]
                  tunnel: [FALSE w383] -> w380
                  frame False {
                  }
                  frame True {
                    n1661 = stacked-sequence {
                      frame #0 {
                      }
                    }
                  }
                }
                "Stop_Buffer" <- w380
              }
              event "OK Button": Value Change {
                n1662 = event-data() -> ()  [unwired: 7 out]
                n1663 = case shown="False" "OK Button" {
                  frame False {
                  }
                  frame True {
                    n1664 = local read "MUX RELAY"() -> (w386:refnum<visa-resource-name>)
                    n1665 = call "ControlRelay_ver10.vi"("VISA session"=w386, "write buffer"="Bb048t" ("element"), "Relay Setting"=T4."Manual Cmd") -> ()  [unwired: 10 in, 7 out]
                  }
                }
              }
              event "OK Button 2": Value Change {
                n1666 = event-data() -> ()  [unwired: 7 out]
                n1667 = case shown="True" "OK Button 2" {
                  frame False {
                  }
                  frame True {
                    n1668 = local read "MUX RELAY"() -> (w390:refnum<visa-resource-name>)
                    n1669 = call "ControlRelay_ver10.vi"("VISA session"=w390, "write buffer"="Bb048f" ("element"), "Relay Setting"=T4."Manual Cmd") -> ()  [unwired: 10 in, 7 out]
                  }
                }
              }
              event "RESET_ICT100": Value Change {
                n1670 = event-data() -> ()  [unwired: 7 out]
                n1671 = case shown="False" "RESET_ICT100" {
                  frame False {
                  }
                  frame True {
                    n1672 = flat-sequence {
                      tunnel: [w395] -> w394
                      tunnel: [w397] -> w393
                      tunnel: w394 -> [w397]
                      tunnel: w393 -> [w399]
                      frame #0 {
                        w395 = refnum<k21> "RESET_ICT100" ("task/channels in")
                        # "low"
                        n1673 = call-poly <vilib>:"DAQmx Write.vi"("task/channels in"=w395, "data"=FALSE) -> ()  [unwired: 11 in, 3 out]
                      }
                      frame #1 {
                        n1674 = Wait (ms)(milliseconds to wait=u32 200) -> ()  [unwired: 1 out]
                      }
                      frame #2 {
                        # "high"
                        n1675 = call-poly <vilib>:"DAQmx Write.vi"("task/channels in"=w399, "data"=TRUE) -> ()  [unwired: 11 in, 3 out]
                      }
                    }
                  }
                }
              }
              event "RUNTEST": Value Change {
                n1676 = event-data() -> ()  [unwired: 7 out]
                n1677 = case shown="True" "RUNTEST" {
                  frame False {
                  }
                  frame True {
                    n1678 = flat-sequence {
                      tunnel: [w404] -> w403
                      tunnel: [w406] -> w402
                      tunnel: w403 -> [w406]
                      tunnel: w402 -> [w408]
                      frame #0 {
                        w404 = refnum<k21> "RUNTEST" ("task/channels in")
                        # "LOW"
                        n1679 = call-poly <vilib>:"DAQmx Write.vi"("task/channels in"=w404, "data"=FALSE) -> ()  [unwired: 11 in, 3 out]
                      }
                      frame #1 {
                        n1680 = Wait (ms)(milliseconds to wait=u32 200) -> ()  [unwired: 1 out]
                      }
                      frame #2 {
                        # "HIGH"
                        n1681 = call-poly <vilib>:"DAQmx Write.vi"("task/channels in"=w408, "data"=TRUE) -> ()  [unwired: 11 in, 3 out]
                      }
                    }
                  }
                }
              }
            }
            n1682 = local read "BarCode Exit"() -> (w378:bool)
            n1683 = Or(x=w377, y=w378) -> (x .or. y?=w379:bool)
          }
        }
      }
      "TESTER ID" <- "FCT1" ("TESTER ID")
      "PASS/FAIL STATUS" <- FALSE ("PASS/FAIL STATUS")
      "UNIT  PASS/FAIL STATUS" <- "" ("String")
      "SOFTWARE REV" <- "Rev1.0" ("SOFTWARE REV")
      "FIRMWARE REV" <- "" ("FIRMWARE REV")
      "CUSTOMER" <- w256
      "Project" <- "" ("Project")
      "Comment" <- "" ("Project")
      "SeqFileSts" <- FALSE ("TP CHK")
      "BarCode Exit" <- FALSE ("BarCode Exit")
      "Step&Description" <- "" ("string buffer")
      "LWL" <- "" ("LWL")
      "UPL" <- "" ("UPL")
      "Reading" <- "" ("Reading")
      "SN-STS" <- i16 0 ("Numeric")
      "PASS/FAIL STATUS  HEAD 1" <- FALSE ("PASS/FAIL STATUS  HEAD1")
      "PASS/FAIL STATUS  HEAD 2" <- FALSE ("PASS/FAIL STATUS  HEAD1")
      "Serial number (Hex)" <- w255
      "Check SUM HEX" <- w255
      "AllowToTest" <- FALSE ("AllowToTest")
      "message" <- "" ("message")
    }
  }
